vi "chose distance.vi"(10 "New direction":string, 11 "Current Direction":string) -> (2 "chosen  distance":dbl)   [LabVIEW 2015]
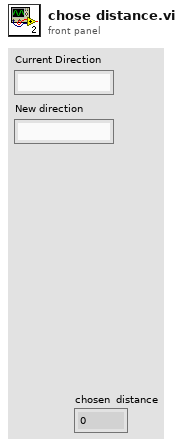
[diagram p1: front panel]
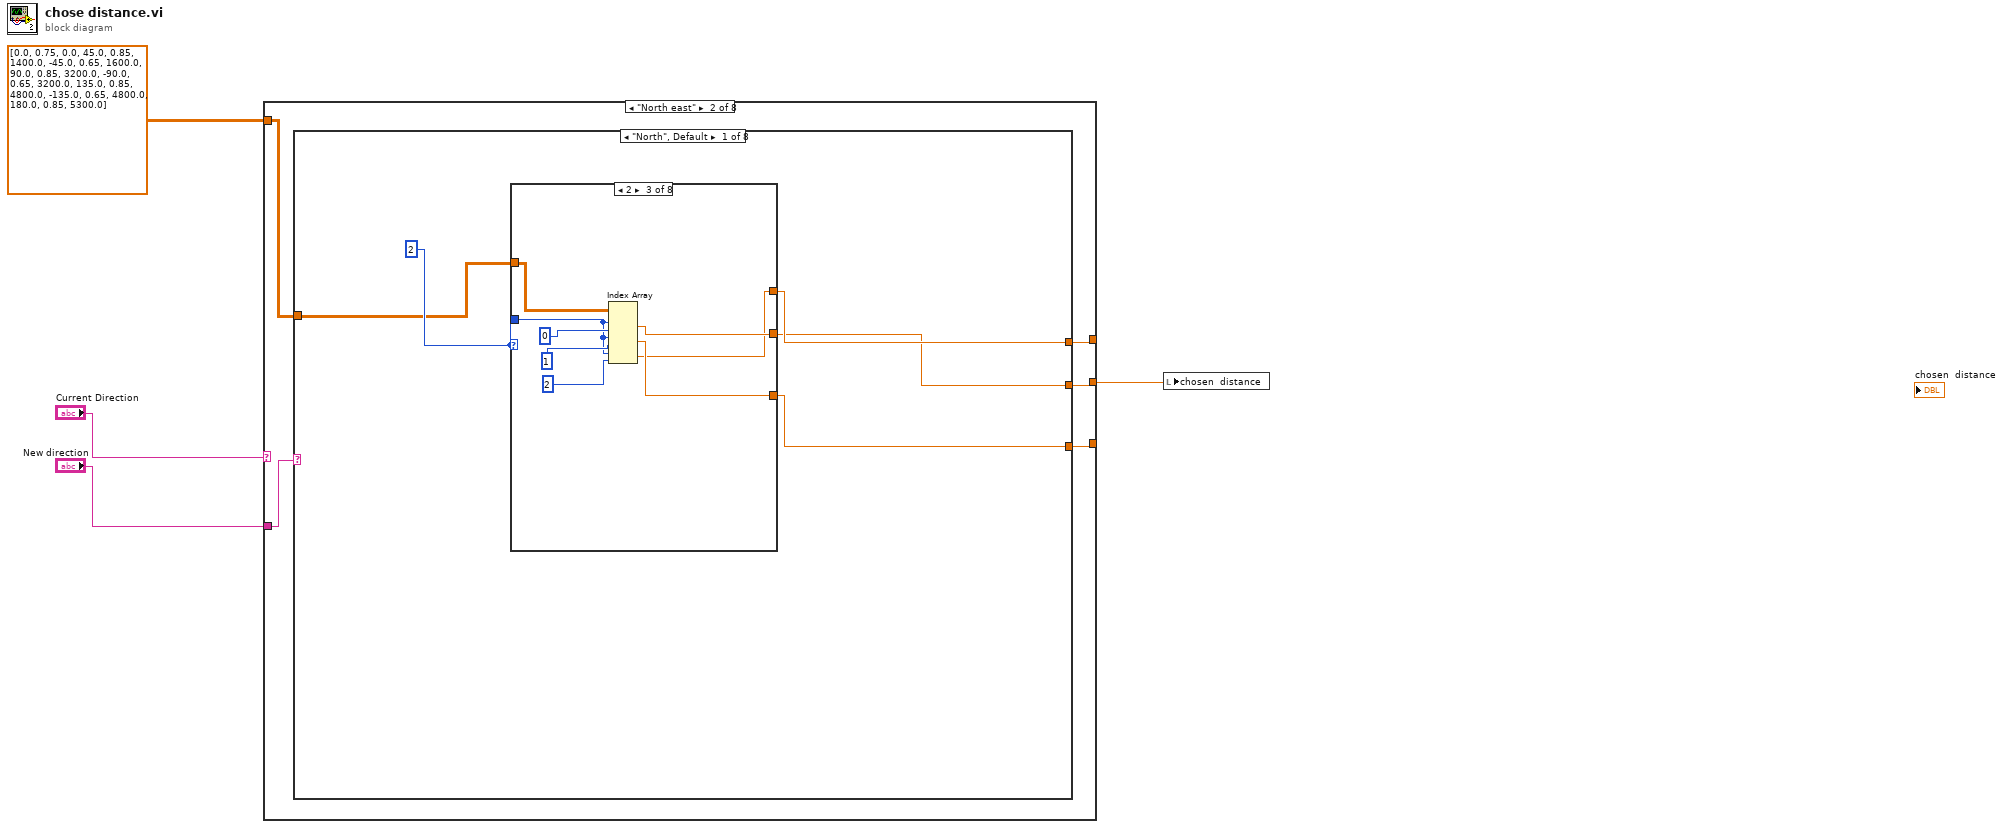
[diagram p0: block diagram]
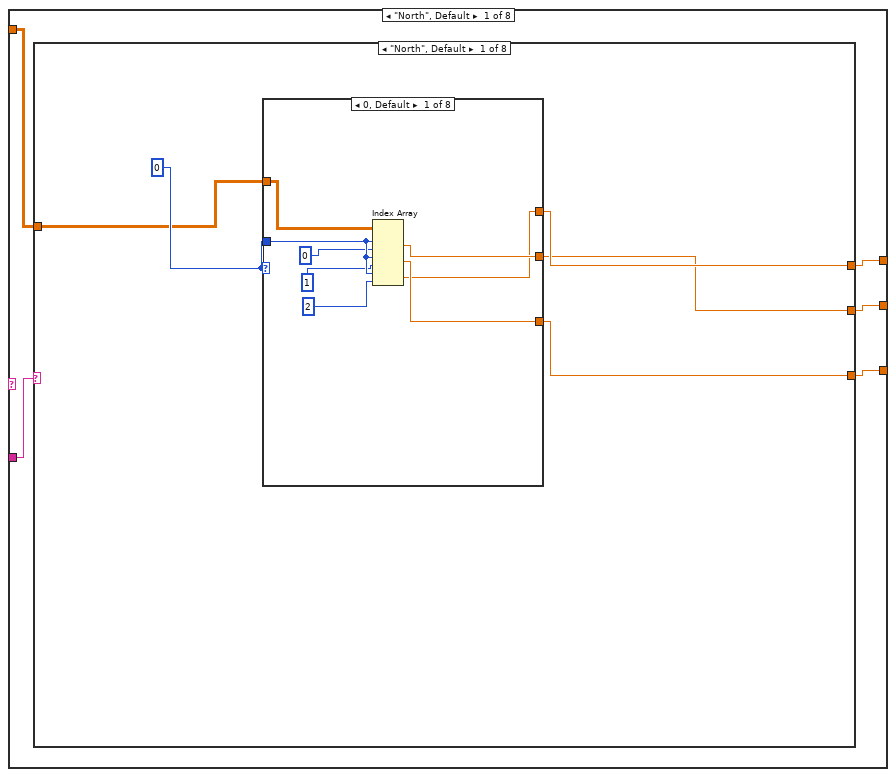
[diagram p2: hidden frame]
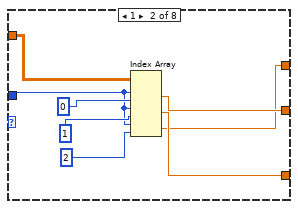
[diagram p3: hidden frame]
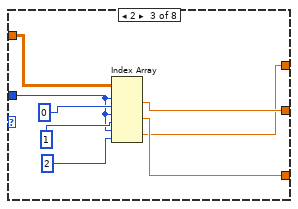
[diagram p4: hidden frame]
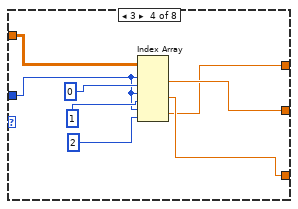
[diagram p5: hidden frame]
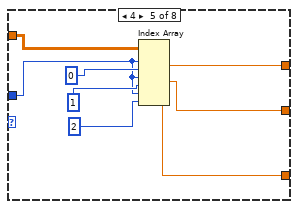
[diagram p6: hidden frame]
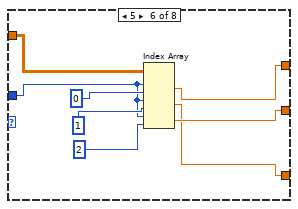
[diagram p7: hidden frame]
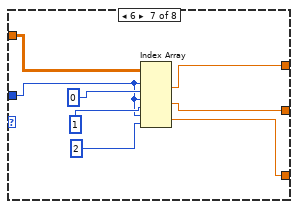
[diagram p8: hidden frame]
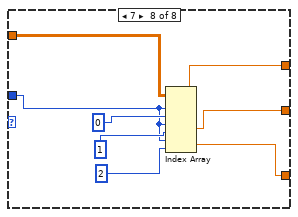
[diagram p9: hidden frame]
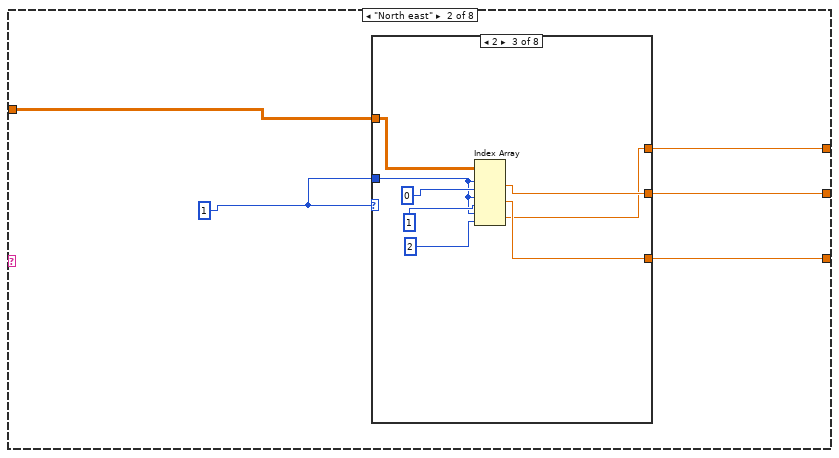
[diagram p10: hidden frame]
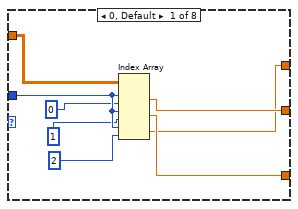
[diagram p11: hidden frame]
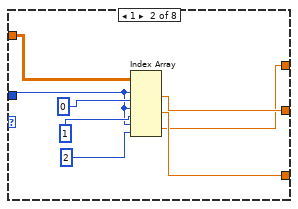
[diagram p12: hidden frame]
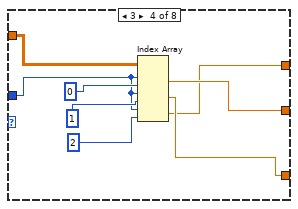
[diagram p13: hidden frame]
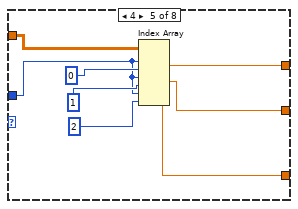
[diagram p14: hidden frame]
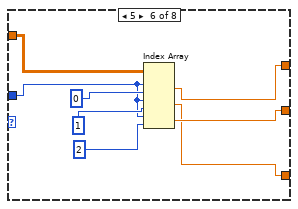
[diagram p15: hidden frame]
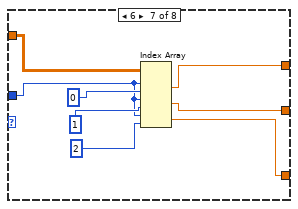
[diagram p16: hidden frame]
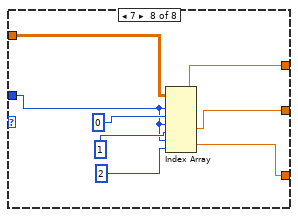
[diagram p17: hidden frame]
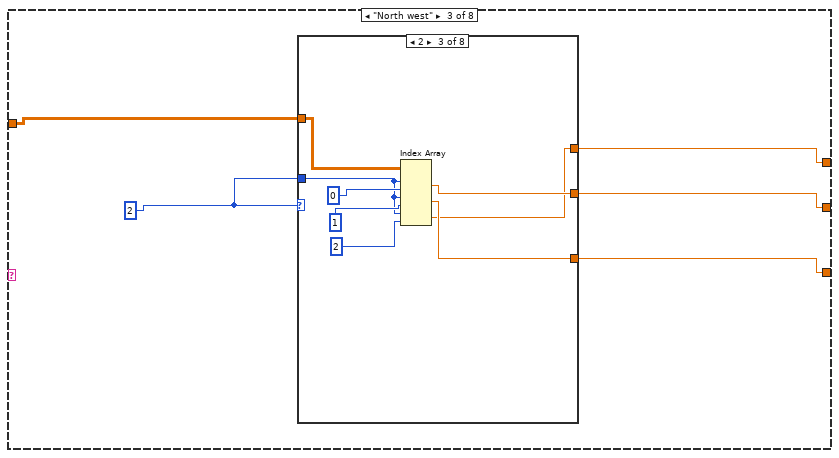
[diagram p18: hidden frame]
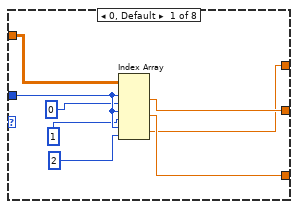
[diagram p19: hidden frame]
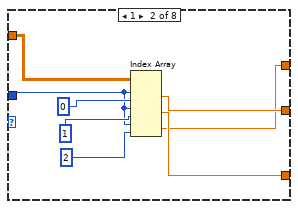
[diagram p20: hidden frame]
diagram:
  n1 = case shown="\"North east\"" "Current Direction" {
    tunnel: [w9 w566 w1123 w1680 w2237 w2794 w3351 w3908] -> _
    tunnel: [w8 w565 w1122 w1679 w2236 w2793 w3350 w3907] -> w1
    tunnel: [w7 w564 w1121 w1678 w2235 w2792 w3349 w3906] -> _
    tunnel: "New direction" -> [w5 w563 w1120 w1677 w2234 w2791 w3348 w3905]
    tunnel: dbl[][] [[0.0, 0.75, 0.0], [45.0, 0.85, 1400.0], [-45.0, 0.65, 1600.0], [90.0, 0.85, 3200.0], [-90.0, 0.65, 3200.0], [135.0, 0.85, 4800.0], [-135.0, 0.65, 4800.0], [180.0, 0.85, 5300.0]] -> [w6 w562 w1119 w1676 w2233 w2790 w3347 w3904]
    frame "North", Default {
      n2 = case shown="\"North\", Default" w5 {
        tunnel: [w13 w83 w151 w218 w288 w358 w426 w496] -> w9
        tunnel: [w12 w82 w150 w219 w287 w356 w425 w495] -> w8
        tunnel: [w11 w81 w149 w217 w286 w355 w424 w494] -> w7
        tunnel: w6 -> [w10 w79 w148 w220 w289 w357 w427 w493]
        frame "North", Default {
          w14 = 0
          n3 = case shown="0, Default" w14 {
            tunnel: [w18 w24 w32 w40 w48 w57 w64 w73] -> w13
            tunnel: [w20 w26 w34 w41 w50 w59 w66 w75] -> w12
            tunnel: [w19 w25 w33 w42 w49 w58 w65 w74] -> w11
            tunnel: w14 -> [w22 w27 w35 w43 w51 w56 w67 w72]
            tunnel: w10 -> [w15 w23 w31 w39 w47 w55 w63 w71]
            frame 0, Default {
              n4 = Index Array(array=w15, index (row) #1=w22, index (col) #1=0, index (row) #2=w22, index (col) #2=1, index (row) #3=w22, index (col) #3=2) -> (element #1=w20:dbl, element #2=w19:dbl, element #3=w18:dbl)
            }
            frame 1 {
              n5 = Index Array(array=w23, index (row) #1=w27, index (col) #1=0, index (row) #2=w27, index (col) #2=1, index (row) #3=w27, index (col) #3=2) -> (element #1=w26:dbl, element #2=w25:dbl, element #3=w24:dbl)
            }
            frame 2 {
              n6 = Index Array(array=w31, index (row) #1=w35, index (col) #1=0, index (row) #2=w35, index (col) #2=1, index (row) #3=w35, index (col) #3=2) -> (element #1=w34:dbl, element #2=w33:dbl, element #3=w32:dbl)
            }
            frame 3 {
              n7 = Index Array(array=w39, index (row) #1=w43, index (col) #1=0, index (row) #2=w43, index (col) #2=1, index (row) #3=w43, index (col) #3=2) -> (element #1=w41:dbl, element #2=w42:dbl, element #3=w40:dbl)
            }
            frame 4 {
              n8 = Index Array(array=w47, index (row) #1=w51, index (col) #1=0, index (row) #2=w51, index (col) #2=1, index (row) #3=w51, index (col) #3=2) -> (element #1=w48:dbl, element #2=w50:dbl, element #3=w49:dbl)
            }
            frame 5 {
              n9 = Index Array(array=w55, index (row) #1=w56, index (col) #1=0, index (row) #2=w56, index (col) #2=1, index (row) #3=w56, index (col) #3=2) -> (element #1=w57:dbl, element #2=w58:dbl, element #3=w59:dbl)
            }
            frame 6 {
              n10 = Index Array(array=w63, index (row) #1=w67, index (col) #1=0, index (row) #2=w67, index (col) #2=1, index (row) #3=w67, index (col) #3=2) -> (element #1=w64:dbl, element #2=w66:dbl, element #3=w65:dbl)
            }
            frame 7 {
              n11 = Index Array(array=w71, index (row) #1=w72, index (col) #1=0, index (row) #2=w72, index (col) #2=1, index (row) #3=w72, index (col) #3=2) -> (element #1=w73:dbl, element #2=w75:dbl, element #3=w74:dbl)
            }
          }
        }
        frame "North east" {
          w80 = 1
          n12 = case shown="2" w80 {
            tunnel: [w87 w93 w101 w109 w117 w126 w133 w142] -> w83
            tunnel: [w89 w95 w103 w110 w119 w128 w135 w144] -> w82
            tunnel: [w88 w94 w102 w111 w118 w127 w134 w143] -> w81
            tunnel: w80 -> [w91 w96 w104 w112 w120 w125 w136 w141]
            tunnel: w79 -> [w84 w92 w100 w108 w116 w124 w132 w140]
            frame 0, Default {
              n13 = Index Array(array=w84, index (row) #1=w91, index (col) #1=0, index (row) #2=w91, index (col) #2=1, index (row) #3=w91, index (col) #3=2) -> (element #1=w89:dbl, element #2=w88:dbl, element #3=w87:dbl)
            }
            frame 1 {
              n14 = Index Array(array=w92, index (row) #1=w96, index (col) #1=0, index (row) #2=w96, index (col) #2=1, index (row) #3=w96, index (col) #3=2) -> (element #1=w95:dbl, element #2=w94:dbl, element #3=w93:dbl)
            }
            frame 2 {
              n15 = Index Array(array=w100, index (row) #1=w104, index (col) #1=0, index (row) #2=w104, index (col) #2=1, index (row) #3=w104, index (col) #3=2) -> (element #1=w103:dbl, element #2=w102:dbl, element #3=w101:dbl)
            }
            frame 3 {
              n16 = Index Array(array=w108, index (row) #1=w112, index (col) #1=0, index (row) #2=w112, index (col) #2=1, index (row) #3=w112, index (col) #3=2) -> (element #1=w110:dbl, element #2=w111:dbl, element #3=w109:dbl)
            }
            frame 4 {
              n17 = Index Array(array=w116, index (row) #1=w120, index (col) #1=0, index (row) #2=w120, index (col) #2=1, index (row) #3=w120, index (col) #3=2) -> (element #1=w117:dbl, element #2=w119:dbl, element #3=w118:dbl)
            }
            frame 5 {
              n18 = Index Array(array=w124, index (row) #1=w125, index (col) #1=0, index (row) #2=w125, index (col) #2=1, index (row) #3=w125, index (col) #3=2) -> (element #1=w126:dbl, element #2=w127:dbl, element #3=w128:dbl)
            }
            frame 6 {
              n19 = Index Array(array=w132, index (row) #1=w136, index (col) #1=0, index (row) #2=w136, index (col) #2=1, index (row) #3=w136, index (col) #3=2) -> (element #1=w133:dbl, element #2=w135:dbl, element #3=w134:dbl)
            }
            frame 7 {
              n20 = Index Array(array=w140, index (row) #1=w141, index (col) #1=0, index (row) #2=w141, index (col) #2=1, index (row) #3=w141, index (col) #3=2) -> (element #1=w142:dbl, element #2=w144:dbl, element #3=w143:dbl)
            }
          }
        }
        frame "North west" {
          w152 = 2
          n21 = case shown="2" w152 {
            tunnel: [w156 w162 w170 w178 w186 w195 w202 w211] -> w151
            tunnel: [w158 w164 w172 w179 w188 w197 w204 w213] -> w150
            tunnel: [w157 w163 w171 w180 w187 w196 w203 w212] -> w149
            tunnel: w152 -> [w160 w165 w173 w181 w189 w194 w205 w210]
            tunnel: w148 -> [w153 w161 w169 w177 w185 w193 w201 w209]
            frame 0, Default {
              n22 = Index Array(array=w153, index (row) #1=w160, index (col) #1=0, index (row) #2=w160, index (col) #2=1, index (row) #3=w160, index (col) #3=2) -> (element #1=w158:dbl, element #2=w157:dbl, element #3=w156:dbl)
            }
            frame 1 {
              n23 = Index Array(array=w161, index (row) #1=w165, index (col) #1=0, index (row) #2=w165, index (col) #2=1, index (row) #3=w165, index (col) #3=2) -> (element #1=w164:dbl, element #2=w163:dbl, element #3=w162:dbl)
            }
            frame 2 {
              n24 = Index Array(array=w169, index (row) #1=w173, index (col) #1=0, index (row) #2=w173, index (col) #2=1, index (row) #3=w173, index (col) #3=2) -> (element #1=w172:dbl, element #2=w171:dbl, element #3=w170:dbl)
            }
            frame 3 {
              n25 = Index Array(array=w177, index (row) #1=w181, index (col) #1=0, index (row) #2=w181, index (col) #2=1, index (row) #3=w181, index (col) #3=2) -> (element #1=w179:dbl, element #2=w180:dbl, element #3=w178:dbl)
            }
            frame 4 {
              n26 = Index Array(array=w185, index (row) #1=w189, index (col) #1=0, index (row) #2=w189, index (col) #2=1, index (row) #3=w189, index (col) #3=2) -> (element #1=w186:dbl, element #2=w188:dbl, element #3=w187:dbl)
            }
            frame 5 {
              n27 = Index Array(array=w193, index (row) #1=w194, index (col) #1=0, index (row) #2=w194, index (col) #2=1, index (row) #3=w194, index (col) #3=2) -> (element #1=w195:dbl, element #2=w196:dbl, element #3=w197:dbl)
            }
            frame 6 {
              n28 = Index Array(array=w201, index (row) #1=w205, index (col) #1=0, index (row) #2=w205, index (col) #2=1, index (row) #3=w205, index (col) #3=2) -> (element #1=w202:dbl, element #2=w204:dbl, element #3=w203:dbl)
            }
            frame 7 {
              n29 = Index Array(array=w209, index (row) #1=w210, index (col) #1=0, index (row) #2=w210, index (col) #2=1, index (row) #3=w210, index (col) #3=2) -> (element #1=w211:dbl, element #2=w213:dbl, element #3=w212:dbl)
            }
          }
        }
        frame "West" {
          w221 = 4
          n30 = case shown="2" w221 {
            tunnel: [w225 w231 w239 w247 w255 w264 w271 w280] -> w218
            tunnel: [w227 w233 w241 w248 w257 w266 w273 w282] -> w219
            tunnel: [w226 w232 w240 w249 w256 w265 w272 w281] -> w217
            tunnel: w221 -> [w229 w234 w242 w250 w258 w263 w274 w279]
            tunnel: w220 -> [w222 w230 w238 w246 w254 w262 w270 w278]
            frame 0, Default {
              n31 = Index Array(array=w222, index (row) #1=w229, index (col) #1=0, index (row) #2=w229, index (col) #2=1, index (row) #3=w229, index (col) #3=2) -> (element #1=w227:dbl, element #2=w226:dbl, element #3=w225:dbl)
            }
            frame 1 {
              n32 = Index Array(array=w230, index (row) #1=w234, index (col) #1=0, index (row) #2=w234, index (col) #2=1, index (row) #3=w234, index (col) #3=2) -> (element #1=w233:dbl, element #2=w232:dbl, element #3=w231:dbl)
            }
            frame 2 {
              n33 = Index Array(array=w238, index (row) #1=w242, index (col) #1=0, index (row) #2=w242, index (col) #2=1, index (row) #3=w242, index (col) #3=2) -> (element #1=w241:dbl, element #2=w240:dbl, element #3=w239:dbl)
            }
            frame 3 {
              n34 = Index Array(array=w246, index (row) #1=w250, index (col) #1=0, index (row) #2=w250, index (col) #2=1, index (row) #3=w250, index (col) #3=2) -> (element #1=w248:dbl, element #2=w249:dbl, element #3=w247:dbl)
            }
            frame 4 {
              n35 = Index Array(array=w254, index (row) #1=w258, index (col) #1=0, index (row) #2=w258, index (col) #2=1, index (row) #3=w258, index (col) #3=2) -> (element #1=w255:dbl, element #2=w257:dbl, element #3=w256:dbl)
            }
            frame 5 {
              n36 = Index Array(array=w262, index (row) #1=w263, index (col) #1=0, index (row) #2=w263, index (col) #2=1, index (row) #3=w263, index (col) #3=2) -> (element #1=w264:dbl, element #2=w265:dbl, element #3=w266:dbl)
            }
            frame 6 {
              n37 = Index Array(array=w270, index (row) #1=w274, index (col) #1=0, index (row) #2=w274, index (col) #2=1, index (row) #3=w274, index (col) #3=2) -> (element #1=w271:dbl, element #2=w273:dbl, element #3=w272:dbl)
            }
            frame 7 {
              n38 = Index Array(array=w278, index (row) #1=w279, index (col) #1=0, index (row) #2=w279, index (col) #2=1, index (row) #3=w279, index (col) #3=2) -> (element #1=w280:dbl, element #2=w282:dbl, element #3=w281:dbl)
            }
          }
        }
        frame "East" {
          w290 = 3
          n39 = case shown="2" w290 {
            tunnel: [w294 w300 w308 w316 w324 w333 w340 w349] -> w288
            tunnel: [w296 w302 w310 w317 w326 w335 w342 w351] -> w287
            tunnel: [w295 w301 w309 w318 w325 w334 w341 w350] -> w286
            tunnel: w290 -> [w298 w303 w311 w319 w327 w332 w343 w348]
            tunnel: w289 -> [w291 w299 w307 w315 w323 w331 w339 w347]
            frame 0, Default {
              n40 = Index Array(array=w291, index (row) #1=w298, index (col) #1=0, index (row) #2=w298, index (col) #2=1, index (row) #3=w298, index (col) #3=2) -> (element #1=w296:dbl, element #2=w295:dbl, element #3=w294:dbl)
            }
            frame 1 {
              n41 = Index Array(array=w299, index (row) #1=w303, index (col) #1=0, index (row) #2=w303, index (col) #2=1, index (row) #3=w303, index (col) #3=2) -> (element #1=w302:dbl, element #2=w301:dbl, element #3=w300:dbl)
            }
            frame 2 {
              n42 = Index Array(array=w307, index (row) #1=w311, index (col) #1=0, index (row) #2=w311, index (col) #2=1, index (row) #3=w311, index (col) #3=2) -> (element #1=w310:dbl, element #2=w309:dbl, element #3=w308:dbl)
            }
            frame 3 {
              n43 = Index Array(array=w315, index (row) #1=w319, index (col) #1=0, index (row) #2=w319, index (col) #2=1, index (row) #3=w319, index (col) #3=2) -> (element #1=w317:dbl, element #2=w318:dbl, element #3=w316:dbl)
            }
            frame 4 {
              n44 = Index Array(array=w323, index (row) #1=w327, index (col) #1=0, index (row) #2=w327, index (col) #2=1, index (row) #3=w327, index (col) #3=2) -> (element #1=w324:dbl, element #2=w326:dbl, element #3=w325:dbl)
            }
            frame 5 {
              n45 = Index Array(array=w331, index (row) #1=w332, index (col) #1=0, index (row) #2=w332, index (col) #2=1, index (row) #3=w332, index (col) #3=2) -> (element #1=w333:dbl, element #2=w334:dbl, element #3=w335:dbl)
            }
            frame 6 {
              n46 = Index Array(array=w339, index (row) #1=w343, index (col) #1=0, index (row) #2=w343, index (col) #2=1, index (row) #3=w343, index (col) #3=2) -> (element #1=w340:dbl, element #2=w342:dbl, element #3=w341:dbl)
            }
            frame 7 {
              n47 = Index Array(array=w347, index (row) #1=w348, index (col) #1=0, index (row) #2=w348, index (col) #2=1, index (row) #3=w348, index (col) #3=2) -> (element #1=w349:dbl, element #2=w351:dbl, element #3=w350:dbl)
            }
          }
        }
        frame "South" {
          w359 = 7
          n48 = case shown="2" w359 {
            tunnel: [w363 w369 w377 w385 w393 w402 w409 w418] -> w358
            tunnel: [w365 w371 w379 w386 w395 w404 w411 w420] -> w356
            tunnel: [w364 w370 w378 w387 w394 w403 w410 w419] -> w355
            tunnel: w359 -> [w367 w372 w380 w388 w396 w401 w412 w417]
            tunnel: w357 -> [w360 w368 w376 w384 w392 w400 w408 w416]
            frame 0, Default {
              n49 = Index Array(array=w360, index (row) #1=w367, index (col) #1=0, index (row) #2=w367, index (col) #2=1, index (row) #3=w367, index (col) #3=2) -> (element #1=w365:dbl, element #2=w364:dbl, element #3=w363:dbl)
            }
            frame 1 {
              n50 = Index Array(array=w368, index (row) #1=w372, index (col) #1=0, index (row) #2=w372, index (col) #2=1, index (row) #3=w372, index (col) #3=2) -> (element #1=w371:dbl, element #2=w370:dbl, element #3=w369:dbl)
            }
            frame 2 {
              n51 = Index Array(array=w376, index (row) #1=w380, index (col) #1=0, index (row) #2=w380, index (col) #2=1, index (row) #3=w380, index (col) #3=2) -> (element #1=w379:dbl, element #2=w378:dbl, element #3=w377:dbl)
            }
            frame 3 {
              n52 = Index Array(array=w384, index (row) #1=w388, index (col) #1=0, index (row) #2=w388, index (col) #2=1, index (row) #3=w388, index (col) #3=2) -> (element #1=w386:dbl, element #2=w387:dbl, element #3=w385:dbl)
            }
            frame 4 {
              n53 = Index Array(array=w392, index (row) #1=w396, index (col) #1=0, index (row) #2=w396, index (col) #2=1, index (row) #3=w396, index (col) #3=2) -> (element #1=w393:dbl, element #2=w395:dbl, element #3=w394:dbl)
            }
            frame 5 {
              n54 = Index Array(array=w400, index (row) #1=w401, index (col) #1=0, index (row) #2=w401, index (col) #2=1, index (row) #3=w401, index (col) #3=2) -> (element #1=w402:dbl, element #2=w403:dbl, element #3=w404:dbl)
            }
            frame 6 {
              n55 = Index Array(array=w408, index (row) #1=w412, index (col) #1=0, index (row) #2=w412, index (col) #2=1, index (row) #3=w412, index (col) #3=2) -> (element #1=w409:dbl, element #2=w411:dbl, element #3=w410:dbl)
            }
            frame 7 {
              n56 = Index Array(array=w416, index (row) #1=w417, index (col) #1=0, index (row) #2=w417, index (col) #2=1, index (row) #3=w417, index (col) #3=2) -> (element #1=w418:dbl, element #2=w420:dbl, element #3=w419:dbl)
            }
          }
        }
        frame "South west" {
          w428 = 6
          n57 = case shown="2" w428 {
            tunnel: [w432 w438 w446 w454 w462 w471 w478 w487] -> w426
            tunnel: [w434 w440 w448 w455 w464 w473 w480 w489] -> w425
            tunnel: [w433 w439 w447 w456 w463 w472 w479 w488] -> w424
            tunnel: w428 -> [w436 w441 w449 w457 w465 w470 w481 w486]
            tunnel: w427 -> [w429 w437 w445 w453 w461 w469 w477 w485]
            frame 0, Default {
              n58 = Index Array(array=w429, index (row) #1=w436, index (col) #1=0, index (row) #2=w436, index (col) #2=1, index (row) #3=w436, index (col) #3=2) -> (element #1=w434:dbl, element #2=w433:dbl, element #3=w432:dbl)
            }
            frame 1 {
              n59 = Index Array(array=w437, index (row) #1=w441, index (col) #1=0, index (row) #2=w441, index (col) #2=1, index (row) #3=w441, index (col) #3=2) -> (element #1=w440:dbl, element #2=w439:dbl, element #3=w438:dbl)
            }
            frame 2 {
              n60 = Index Array(array=w445, index (row) #1=w449, index (col) #1=0, index (row) #2=w449, index (col) #2=1, index (row) #3=w449, index (col) #3=2) -> (element #1=w448:dbl, element #2=w447:dbl, element #3=w446:dbl)
            }
            frame 3 {
              n61 = Index Array(array=w453, index (row) #1=w457, index (col) #1=0, index (row) #2=w457, index (col) #2=1, index (row) #3=w457, index (col) #3=2) -> (element #1=w455:dbl, element #2=w456:dbl, element #3=w454:dbl)
            }
            frame 4 {
              n62 = Index Array(array=w461, index (row) #1=w465, index (col) #1=0, index (row) #2=w465, index (col) #2=1, index (row) #3=w465, index (col) #3=2) -> (element #1=w462:dbl, element #2=w464:dbl, element #3=w463:dbl)
            }
            frame 5 {
              n63 = Index Array(array=w469, index (row) #1=w470, index (col) #1=0, index (row) #2=w470, index (col) #2=1, index (row) #3=w470, index (col) #3=2) -> (element #1=w471:dbl, element #2=w472:dbl, element #3=w473:dbl)
            }
            frame 6 {
              n64 = Index Array(array=w477, index (row) #1=w481, index (col) #1=0, index (row) #2=w481, index (col) #2=1, index (row) #3=w481, index (col) #3=2) -> (element #1=w478:dbl, element #2=w480:dbl, element #3=w479:dbl)
            }
            frame 7 {
              n65 = Index Array(array=w485, index (row) #1=w486, index (col) #1=0, index (row) #2=w486, index (col) #2=1, index (row) #3=w486, index (col) #3=2) -> (element #1=w487:dbl, element #2=w489:dbl, element #3=w488:dbl)
            }
          }
        }
        frame "South east" {
          w497 = 5
          n66 = case shown="2" w497 {
            tunnel: [w501 w507 w515 w523 w531 w540 w547 w556] -> w496
            tunnel: [w503 w509 w517 w524 w533 w542 w549 w558] -> w495
            tunnel: [w502 w508 w516 w525 w532 w541 w548 w557] -> w494
            tunnel: w497 -> [w505 w510 w518 w526 w534 w539 w550 w555]
            tunnel: w493 -> [w498 w506 w514 w522 w530 w538 w546 w554]
            frame 0, Default {
              n67 = Index Array(array=w498, index (row) #1=w505, index (col) #1=0, index (row) #2=w505, index (col) #2=1, index (row) #3=w505, index (col) #3=2) -> (element #1=w503:dbl, element #2=w502:dbl, element #3=w501:dbl)
            }
            frame 1 {
              n68 = Index Array(array=w506, index (row) #1=w510, index (col) #1=0, index (row) #2=w510, index (col) #2=1, index (row) #3=w510, index (col) #3=2) -> (element #1=w509:dbl, element #2=w508:dbl, element #3=w507:dbl)
            }
            frame 2 {
              n69 = Index Array(array=w514, index (row) #1=w518, index (col) #1=0, index (row) #2=w518, index (col) #2=1, index (row) #3=w518, index (col) #3=2) -> (element #1=w517:dbl, element #2=w516:dbl, element #3=w515:dbl)
            }
            frame 3 {
              n70 = Index Array(array=w522, index (row) #1=w526, index (col) #1=0, index (row) #2=w526, index (col) #2=1, index (row) #3=w526, index (col) #3=2) -> (element #1=w524:dbl, element #2=w525:dbl, element #3=w523:dbl)
            }
            frame 4 {
              n71 = Index Array(array=w530, index (row) #1=w534, index (col) #1=0, index (row) #2=w534, index (col) #2=1, index (row) #3=w534, index (col) #3=2) -> (element #1=w531:dbl, element #2=w533:dbl, element #3=w532:dbl)
            }
            frame 5 {
              n72 = Index Array(array=w538, index (row) #1=w539, index (col) #1=0, index (row) #2=w539, index (col) #2=1, index (row) #3=w539, index (col) #3=2) -> (element #1=w540:dbl, element #2=w541:dbl, element #3=w542:dbl)
            }
            frame 6 {
              n73 = Index Array(array=w546, index (row) #1=w550, index (col) #1=0, index (row) #2=w550, index (col) #2=1, index (row) #3=w550, index (col) #3=2) -> (element #1=w547:dbl, element #2=w549:dbl, element #3=w548:dbl)
            }
            frame 7 {
              n74 = Index Array(array=w554, index (row) #1=w555, index (col) #1=0, index (row) #2=w555, index (col) #2=1, index (row) #3=w555, index (col) #3=2) -> (element #1=w556:dbl, element #2=w558:dbl, element #3=w557:dbl)
            }
          }
        }
      }
    }
    frame "North east" {
      n75 = case shown="\"North\", Default" w563 {
        tunnel: [w570 w640 w708 w775 w845 w915 w983 w1053] -> w566
        tunnel: [w569 w639 w707 w776 w844 w913 w982 w1052] -> w565
        tunnel: [w568 w638 w706 w774 w843 w912 w981 w1051] -> w564
        tunnel: w562 -> [w567 w636 w705 w777 w846 w914 w984 w1050]
        frame "North", Default {
          w571 = 2
          n76 = case shown="2" w571 {
            tunnel: [w575 w581 w589 w597 w605 w614 w621 w630] -> w570
            tunnel: [w577 w583 w591 w598 w607 w616 w623 w632] -> w569
            tunnel: [w576 w582 w590 w599 w606 w615 w622 w631] -> w568
            tunnel: w571 -> [w579 w584 w592 w600 w608 w613 w624 w629]
            tunnel: w567 -> [w572 w580 w588 w596 w604 w612 w620 w628]
            frame 0, Default {
              n77 = Index Array(array=w572, index (row) #1=w579, index (col) #1=0, index (row) #2=w579, index (col) #2=1, index (row) #3=w579, index (col) #3=2) -> (element #1=w577:dbl, element #2=w576:dbl, element #3=w575:dbl)
            }
            frame 1 {
              n78 = Index Array(array=w580, index (row) #1=w584, index (col) #1=0, index (row) #2=w584, index (col) #2=1, index (row) #3=w584, index (col) #3=2) -> (element #1=w583:dbl, element #2=w582:dbl, element #3=w581:dbl)
            }
            frame 2 {
              n79 = Index Array(array=w588, index (row) #1=w592, index (col) #1=0, index (row) #2=w592, index (col) #2=1, index (row) #3=w592, index (col) #3=2) -> (element #1=w591:dbl, element #2=w590:dbl, element #3=w589:dbl)
            }
            frame 3 {
              n80 = Index Array(array=w596, index (row) #1=w600, index (col) #1=0, index (row) #2=w600, index (col) #2=1, index (row) #3=w600, index (col) #3=2) -> (element #1=w598:dbl, element #2=w599:dbl, element #3=w597:dbl)
            }
            frame 4 {
              n81 = Index Array(array=w604, index (row) #1=w608, index (col) #1=0, index (row) #2=w608, index (col) #2=1, index (row) #3=w608, index (col) #3=2) -> (element #1=w605:dbl, element #2=w607:dbl, element #3=w606:dbl)
            }
            frame 5 {
              n82 = Index Array(array=w612, index (row) #1=w613, index (col) #1=0, index (row) #2=w613, index (col) #2=1, index (row) #3=w613, index (col) #3=2) -> (element #1=w614:dbl, element #2=w615:dbl, element #3=w616:dbl)
            }
            frame 6 {
              n83 = Index Array(array=w620, index (row) #1=w624, index (col) #1=0, index (row) #2=w624, index (col) #2=1, index (row) #3=w624, index (col) #3=2) -> (element #1=w621:dbl, element #2=w623:dbl, element #3=w622:dbl)
            }
            frame 7 {
              n84 = Index Array(array=w628, index (row) #1=w629, index (col) #1=0, index (row) #2=w629, index (col) #2=1, index (row) #3=w629, index (col) #3=2) -> (element #1=w630:dbl, element #2=w632:dbl, element #3=w631:dbl)
            }
          }
        }
        frame "North east" {
          w637 = 0
          n85 = case shown="2" w637 {
            tunnel: [w644 w650 w658 w666 w674 w683 w690 w699] -> w640
            tunnel: [w646 w652 w660 w667 w676 w685 w692 w701] -> w639
            tunnel: [w645 w651 w659 w668 w675 w684 w691 w700] -> w638
            tunnel: w637 -> [w648 w653 w661 w669 w677 w682 w693 w698]
            tunnel: w636 -> [w641 w649 w657 w665 w673 w681 w689 w697]
            frame 0, Default {
              n86 = Index Array(array=w641, index (row) #1=w648, index (col) #1=0, index (row) #2=w648, index (col) #2=1, index (row) #3=w648, index (col) #3=2) -> (element #1=w646:dbl, element #2=w645:dbl, element #3=w644:dbl)
            }
            frame 1 {
              n87 = Index Array(array=w649, index (row) #1=w653, index (col) #1=0, index (row) #2=w653, index (col) #2=1, index (row) #3=w653, index (col) #3=2) -> (element #1=w652:dbl, element #2=w651:dbl, element #3=w650:dbl)
            }
            frame 2 {
              n88 = Index Array(array=w657, index (row) #1=w661, index (col) #1=0, index (row) #2=w661, index (col) #2=1, index (row) #3=w661, index (col) #3=2) -> (element #1=w660:dbl, element #2=w659:dbl, element #3=w658:dbl)
            }
            frame 3 {
              n89 = Index Array(array=w665, index (row) #1=w669, index (col) #1=0, index (row) #2=w669, index (col) #2=1, index (row) #3=w669, index (col) #3=2) -> (element #1=w667:dbl, element #2=w668:dbl, element #3=w666:dbl)
            }
            frame 4 {
              n90 = Index Array(array=w673, index (row) #1=w677, index (col) #1=0, index (row) #2=w677, index (col) #2=1, index (row) #3=w677, index (col) #3=2) -> (element #1=w674:dbl, element #2=w676:dbl, element #3=w675:dbl)
            }
            frame 5 {
              n91 = Index Array(array=w681, index (row) #1=w682, index (col) #1=0, index (row) #2=w682, index (col) #2=1, index (row) #3=w682, index (col) #3=2) -> (element #1=w683:dbl, element #2=w684:dbl, element #3=w685:dbl)
            }
            frame 6 {
              n92 = Index Array(array=w689, index (row) #1=w693, index (col) #1=0, index (row) #2=w693, index (col) #2=1, index (row) #3=w693, index (col) #3=2) -> (element #1=w690:dbl, element #2=w692:dbl, element #3=w691:dbl)
            }
            frame 7 {
              n93 = Index Array(array=w697, index (row) #1=w698, index (col) #1=0, index (row) #2=w698, index (col) #2=1, index (row) #3=w698, index (col) #3=2) -> (element #1=w699:dbl, element #2=w701:dbl, element #3=w700:dbl)
            }
          }
        }
        frame "North west" {
          w709 = 4
          n94 = case shown="2" w709 {
            tunnel: [w713 w719 w727 w735 w743 w752 w759 w768] -> w708
            tunnel: [w715 w721 w729 w736 w745 w754 w761 w770] -> w707
            tunnel: [w714 w720 w728 w737 w744 w753 w760 w769] -> w706
            tunnel: w709 -> [w717 w722 w730 w738 w746 w751 w762 w767]
            tunnel: w705 -> [w710 w718 w726 w734 w742 w750 w758 w766]
            frame 0, Default {
              n95 = Index Array(array=w710, index (row) #1=w717, index (col) #1=0, index (row) #2=w717, index (col) #2=1, index (row) #3=w717, index (col) #3=2) -> (element #1=w715:dbl, element #2=w714:dbl, element #3=w713:dbl)
            }
            frame 1 {
              n96 = Index Array(array=w718, index (row) #1=w722, index (col) #1=0, index (row) #2=w722, index (col) #2=1, index (row) #3=w722, index (col) #3=2) -> (element #1=w721:dbl, element #2=w720:dbl, element #3=w719:dbl)
            }
            frame 2 {
              n97 = Index Array(array=w726, index (row) #1=w730, index (col) #1=0, index (row) #2=w730, index (col) #2=1, index (row) #3=w730, index (col) #3=2) -> (element #1=w729:dbl, element #2=w728:dbl, element #3=w727:dbl)
            }
            frame 3 {
              n98 = Index Array(array=w734, index (row) #1=w738, index (col) #1=0, index (row) #2=w738, index (col) #2=1, index (row) #3=w738, index (col) #3=2) -> (element #1=w736:dbl, element #2=w737:dbl, element #3=w735:dbl)
            }
            frame 4 {
              n99 = Index Array(array=w742, index (row) #1=w746, index (col) #1=0, index (row) #2=w746, index (col) #2=1, index (row) #3=w746, index (col) #3=2) -> (element #1=w743:dbl, element #2=w745:dbl, element #3=w744:dbl)
            }
            frame 5 {
              n100 = Index Array(array=w750, index (row) #1=w751, index (col) #1=0, index (row) #2=w751, index (col) #2=1, index (row) #3=w751, index (col) #3=2) -> (element #1=w752:dbl, element #2=w753:dbl, element #3=w754:dbl)
            }
            frame 6 {
              n101 = Index Array(array=w758, index (row) #1=w762, index (col) #1=0, index (row) #2=w762, index (col) #2=1, index (row) #3=w762, index (col) #3=2) -> (element #1=w759:dbl, element #2=w761:dbl, element #3=w760:dbl)
            }
            frame 7 {
              n102 = Index Array(array=w766, index (row) #1=w767, index (col) #1=0, index (row) #2=w767, index (col) #2=1, index (row) #3=w767, index (col) #3=2) -> (element #1=w768:dbl, element #2=w770:dbl, element #3=w769:dbl)
            }
          }
        }
        frame "West" {
          w778 = 6
          n103 = case shown="2" w778 {
            tunnel: [w782 w788 w796 w804 w812 w821 w828 w837] -> w775
            tunnel: [w784 w790 w798 w805 w814 w823 w830 w839] -> w776
            tunnel: [w783 w789 w797 w806 w813 w822 w829 w838] -> w774
            tunnel: w778 -> [w786 w791 w799 w807 w815 w820 w831 w836]
            tunnel: w777 -> [w779 w787 w795 w803 w811 w819 w827 w835]
            frame 0, Default {
              n104 = Index Array(array=w779, index (row) #1=w786, index (col) #1=0, index (row) #2=w786, index (col) #2=1, index (row) #3=w786, index (col) #3=2) -> (element #1=w784:dbl, element #2=w783:dbl, element #3=w782:dbl)
            }
            frame 1 {
              n105 = Index Array(array=w787, index (row) #1=w791, index (col) #1=0, index (row) #2=w791, index (col) #2=1, index (row) #3=w791, index (col) #3=2) -> (element #1=w790:dbl, element #2=w789:dbl, element #3=w788:dbl)
            }
            frame 2 {
              n106 = Index Array(array=w795, index (row) #1=w799, index (col) #1=0, index (row) #2=w799, index (col) #2=1, index (row) #3=w799, index (col) #3=2) -> (element #1=w798:dbl, element #2=w797:dbl, element #3=w796:dbl)
            }
            frame 3 {
              n107 = Index Array(array=w803, index (row) #1=w807, index (col) #1=0, index (row) #2=w807, index (col) #2=1, index (row) #3=w807, index (col) #3=2) -> (element #1=w805:dbl, element #2=w806:dbl, element #3=w804:dbl)
            }
            frame 4 {
              n108 = Index Array(array=w811, index (row) #1=w815, index (col) #1=0, index (row) #2=w815, index (col) #2=1, index (row) #3=w815, index (col) #3=2) -> (element #1=w812:dbl, element #2=w814:dbl, element #3=w813:dbl)
            }
            frame 5 {
              n109 = Index Array(array=w819, index (row) #1=w820, index (col) #1=0, index (row) #2=w820, index (col) #2=1, index (row) #3=w820, index (col) #3=2) -> (element #1=w821:dbl, element #2=w822:dbl, element #3=w823:dbl)
            }
            frame 6 {
              n110 = Index Array(array=w827, index (row) #1=w831, index (col) #1=0, index (row) #2=w831, index (col) #2=1, index (row) #3=w831, index (col) #3=2) -> (element #1=w828:dbl, element #2=w830:dbl, element #3=w829:dbl)
            }
            frame 7 {
              n111 = Index Array(array=w835, index (row) #1=w836, index (col) #1=0, index (row) #2=w836, index (col) #2=1, index (row) #3=w836, index (col) #3=2) -> (element #1=w837:dbl, element #2=w839:dbl, element #3=w838:dbl)
            }
          }
        }
        frame "East" {
          w847 = 1
          n112 = case shown="2" w847 {
            tunnel: [w851 w857 w865 w873 w881 w890 w897 w906] -> w845
            tunnel: [w853 w859 w867 w874 w883 w892 w899 w908] -> w844
            tunnel: [w852 w858 w866 w875 w882 w891 w898 w907] -> w843
            tunnel: w847 -> [w855 w860 w868 w876 w884 w889 w900 w905]
            tunnel: w846 -> [w848 w856 w864 w872 w880 w888 w896 w904]
            frame 0, Default {
              n113 = Index Array(array=w848, index (row) #1=w855, index (col) #1=0, index (row) #2=w855, index (col) #2=1, index (row) #3=w855, index (col) #3=2) -> (element #1=w853:dbl, element #2=w852:dbl, element #3=w851:dbl)
            }
            frame 1 {
              n114 = Index Array(array=w856, index (row) #1=w860, index (col) #1=0, index (row) #2=w860, index (col) #2=1, index (row) #3=w860, index (col) #3=2) -> (element #1=w859:dbl, element #2=w858:dbl, element #3=w857:dbl)
            }
            frame 2 {
              n115 = Index Array(array=w864, index (row) #1=w868, index (col) #1=0, index (row) #2=w868, index (col) #2=1, index (row) #3=w868, index (col) #3=2) -> (element #1=w867:dbl, element #2=w866:dbl, element #3=w865:dbl)
            }
            frame 3 {
              n116 = Index Array(array=w872, index (row) #1=w876, index (col) #1=0, index (row) #2=w876, index (col) #2=1, index (row) #3=w876, index (col) #3=2) -> (element #1=w874:dbl, element #2=w875:dbl, element #3=w873:dbl)
            }
            frame 4 {
              n117 = Index Array(array=w880, index (row) #1=w884, index (col) #1=0, index (row) #2=w884, index (col) #2=1, index (row) #3=w884, index (col) #3=2) -> (element #1=w881:dbl, element #2=w883:dbl, element #3=w882:dbl)
            }
            frame 5 {
              n118 = Index Array(array=w888, index (row) #1=w889, index (col) #1=0, index (row) #2=w889, index (col) #2=1, index (row) #3=w889, index (col) #3=2) -> (element #1=w890:dbl, element #2=w891:dbl, element #3=w892:dbl)
            }
            frame 6 {
              n119 = Index Array(array=w896, index (row) #1=w900, index (col) #1=0, index (row) #2=w900, index (col) #2=1, index (row) #3=w900, index (col) #3=2) -> (element #1=w897:dbl, element #2=w899:dbl, element #3=w898:dbl)
            }
            frame 7 {
              n120 = Index Array(array=w904, index (row) #1=w905, index (col) #1=0, index (row) #2=w905, index (col) #2=1, index (row) #3=w905, index (col) #3=2) -> (element #1=w906:dbl, element #2=w908:dbl, element #3=w907:dbl)
            }
          }
        }
        frame "South" {
          w916 = 5
          n121 = case shown="2" w916 {
            tunnel: [w920 w926 w934 w942 w950 w959 w966 w975] -> w915
            tunnel: [w922 w928 w936 w943 w952 w961 w968 w977] -> w913
            tunnel: [w921 w927 w935 w944 w951 w960 w967 w976] -> w912
            tunnel: w916 -> [w924 w929 w937 w945 w953 w958 w969 w974]
            tunnel: w914 -> [w917 w925 w933 w941 w949 w957 w965 w973]
            frame 0, Default {
              n122 = Index Array(array=w917, index (row) #1=w924, index (col) #1=0, index (row) #2=w924, index (col) #2=1, index (row) #3=w924, index (col) #3=2) -> (element #1=w922:dbl, element #2=w921:dbl, element #3=w920:dbl)
            }
            frame 1 {
              n123 = Index Array(array=w925, index (row) #1=w929, index (col) #1=0, index (row) #2=w929, index (col) #2=1, index (row) #3=w929, index (col) #3=2) -> (element #1=w928:dbl, element #2=w927:dbl, element #3=w926:dbl)
            }
            frame 2 {
              n124 = Index Array(array=w933, index (row) #1=w937, index (col) #1=0, index (row) #2=w937, index (col) #2=1, index (row) #3=w937, index (col) #3=2) -> (element #1=w936:dbl, element #2=w935:dbl, element #3=w934:dbl)
            }
            frame 3 {
              n125 = Index Array(array=w941, index (row) #1=w945, index (col) #1=0, index (row) #2=w945, index (col) #2=1, index (row) #3=w945, index (col) #3=2) -> (element #1=w943:dbl, element #2=w944:dbl, element #3=w942:dbl)
            }
            frame 4 {
              n126 = Index Array(array=w949, index (row) #1=w953, index (col) #1=0, index (row) #2=w953, index (col) #2=1, index (row) #3=w953, index (col) #3=2) -> (element #1=w950:dbl, element #2=w952:dbl, element #3=w951:dbl)
            }
            frame 5 {
              n127 = Index Array(array=w957, index (row) #1=w958, index (col) #1=0, index (row) #2=w958, index (col) #2=1, index (row) #3=w958, index (col) #3=2) -> (element #1=w959:dbl, element #2=w960:dbl, element #3=w961:dbl)
            }
            frame 6 {
              n128 = Index Array(array=w965, index (row) #1=w969, index (col) #1=0, index (row) #2=w969, index (col) #2=1, index (row) #3=w969, index (col) #3=2) -> (element #1=w966:dbl, element #2=w968:dbl, element #3=w967:dbl)
            }
            frame 7 {
              n129 = Index Array(array=w973, index (row) #1=w974, index (col) #1=0, index (row) #2=w974, index (col) #2=1, index (row) #3=w974, index (col) #3=2) -> (element #1=w975:dbl, element #2=w977:dbl, element #3=w976:dbl)
            }
          }
        }
        frame "South west" {
          w985 = 7
          n130 = case shown="2" w985 {
            tunnel: [w989 w995 w1003 w1011 w1019 w1028 w1035 w1044] -> w983
            tunnel: [w991 w997 w1005 w1012 w1021 w1030 w1037 w1046] -> w982
            tunnel: [w990 w996 w1004 w1013 w1020 w1029 w1036 w1045] -> w981
            tunnel: w985 -> [w993 w998 w1006 w1014 w1022 w1027 w1038 w1043]
            tunnel: w984 -> [w986 w994 w1002 w1010 w1018 w1026 w1034 w1042]
            frame 0, Default {
              n131 = Index Array(array=w986, index (row) #1=w993, index (col) #1=0, index (row) #2=w993, index (col) #2=1, index (row) #3=w993, index (col) #3=2) -> (element #1=w991:dbl, element #2=w990:dbl, element #3=w989:dbl)
            }
            frame 1 {
              n132 = Index Array(array=w994, index (row) #1=w998, index (col) #1=0, index (row) #2=w998, index (col) #2=1, index (row) #3=w998, index (col) #3=2) -> (element #1=w997:dbl, element #2=w996:dbl, element #3=w995:dbl)
            }
            frame 2 {
              n133 = Index Array(array=w1002, index (row) #1=w1006, index (col) #1=0, index (row) #2=w1006, index (col) #2=1, index (row) #3=w1006, index (col) #3=2) -> (element #1=w1005:dbl, element #2=w1004:dbl, element #3=w1003:dbl)
            }
            frame 3 {
              n134 = Index Array(array=w1010, index (row) #1=w1014, index (col) #1=0, index (row) #2=w1014, index (col) #2=1, index (row) #3=w1014, index (col) #3=2) -> (element #1=w1012:dbl, element #2=w1013:dbl, element #3=w1011:dbl)
            }
            frame 4 {
              n135 = Index Array(array=w1018, index (row) #1=w1022, index (col) #1=0, index (row) #2=w1022, index (col) #2=1, index (row) #3=w1022, index (col) #3=2) -> (element #1=w1019:dbl, element #2=w1021:dbl, element #3=w1020:dbl)
            }
            frame 5 {
              n136 = Index Array(array=w1026, index (row) #1=w1027, index (col) #1=0, index (row) #2=w1027, index (col) #2=1, index (row) #3=w1027, index (col) #3=2) -> (element #1=w1028:dbl, element #2=w1029:dbl, element #3=w1030:dbl)
            }
            frame 6 {
              n137 = Index Array(array=w1034, index (row) #1=w1038, index (col) #1=0, index (row) #2=w1038, index (col) #2=1, index (row) #3=w1038, index (col) #3=2) -> (element #1=w1035:dbl, element #2=w1037:dbl, element #3=w1036:dbl)
            }
            frame 7 {
              n138 = Index Array(array=w1042, index (row) #1=w1043, index (col) #1=0, index (row) #2=w1043, index (col) #2=1, index (row) #3=w1043, index (col) #3=2) -> (element #1=w1044:dbl, element #2=w1046:dbl, element #3=w1045:dbl)
            }
          }
        }
        frame "South east" {
          w1054 = 3
          n139 = case shown="2" w1054 {
            tunnel: [w1058 w1064 w1072 w1080 w1088 w1097 w1104 w1113] -> w1053
            tunnel: [w1060 w1066 w1074 w1081 w1090 w1099 w1106 w1115] -> w1052
            tunnel: [w1059 w1065 w1073 w1082 w1089 w1098 w1105 w1114] -> w1051
            tunnel: w1054 -> [w1062 w1067 w1075 w1083 w1091 w1096 w1107 w1112]
            tunnel: w1050 -> [w1055 w1063 w1071 w1079 w1087 w1095 w1103 w1111]
            frame 0, Default {
              n140 = Index Array(array=w1055, index (row) #1=w1062, index (col) #1=0, index (row) #2=w1062, index (col) #2=1, index (row) #3=w1062, index (col) #3=2) -> (element #1=w1060:dbl, element #2=w1059:dbl, element #3=w1058:dbl)
            }
            frame 1 {
              n141 = Index Array(array=w1063, index (row) #1=w1067, index (col) #1=0, index (row) #2=w1067, index (col) #2=1, index (row) #3=w1067, index (col) #3=2) -> (element #1=w1066:dbl, element #2=w1065:dbl, element #3=w1064:dbl)
            }
            frame 2 {
              n142 = Index Array(array=w1071, index (row) #1=w1075, index (col) #1=0, index (row) #2=w1075, index (col) #2=1, index (row) #3=w1075, index (col) #3=2) -> (element #1=w1074:dbl, element #2=w1073:dbl, element #3=w1072:dbl)
            }
            frame 3 {
              n143 = Index Array(array=w1079, index (row) #1=w1083, index (col) #1=0, index (row) #2=w1083, index (col) #2=1, index (row) #3=w1083, index (col) #3=2) -> (element #1=w1081:dbl, element #2=w1082:dbl, element #3=w1080:dbl)
            }
            frame 4 {
              n144 = Index Array(array=w1087, index (row) #1=w1091, index (col) #1=0, index (row) #2=w1091, index (col) #2=1, index (row) #3=w1091, index (col) #3=2) -> (element #1=w1088:dbl, element #2=w1090:dbl, element #3=w1089:dbl)
            }
            frame 5 {
              n145 = Index Array(array=w1095, index (row) #1=w1096, index (col) #1=0, index (row) #2=w1096, index (col) #2=1, index (row) #3=w1096, index (col) #3=2) -> (element #1=w1097:dbl, element #2=w1098:dbl, element #3=w1099:dbl)
            }
            frame 6 {
              n146 = Index Array(array=w1103, index (row) #1=w1107, index (col) #1=0, index (row) #2=w1107, index (col) #2=1, index (row) #3=w1107, index (col) #3=2) -> (element #1=w1104:dbl, element #2=w1106:dbl, element #3=w1105:dbl)
            }
            frame 7 {
              n147 = Index Array(array=w1111, index (row) #1=w1112, index (col) #1=0, index (row) #2=w1112, index (col) #2=1, index (row) #3=w1112, index (col) #3=2) -> (element #1=w1113:dbl, element #2=w1115:dbl, element #3=w1114:dbl)
            }
          }
        }
      }
    }
    frame "North west" {
      n148 = case shown="\"South east\"" w1120 {
        tunnel: [w1127 w1197 w1265 w1332 w1402 w1472 w1540 w1610] -> w1123
        tunnel: [w1126 w1196 w1264 w1333 w1401 w1470 w1539 w1609] -> w1122
        tunnel: [w1125 w1195 w1263 w1331 w1400 w1469 w1538 w1608] -> w1121
        tunnel: w1119 -> [w1124 w1193 w1262 w1334 w1403 w1471 w1541 w1607]
        frame "North", Default {
          w1128 = 1
          n149 = case shown="2" w1128 {
            tunnel: [w1132 w1138 w1146 w1154 w1162 w1171 w1178 w1187] -> w1127
            tunnel: [w1134 w1140 w1148 w1155 w1164 w1173 w1180 w1189] -> w1126
            tunnel: [w1133 w1139 w1147 w1156 w1163 w1172 w1179 w1188] -> w1125
            tunnel: w1128 -> [w1136 w1141 w1149 w1157 w1165 w1170 w1181 w1186]
            tunnel: w1124 -> [w1129 w1137 w1145 w1153 w1161 w1169 w1177 w1185]
            frame 0, Default {
              n150 = Index Array(array=w1129, index (row) #1=w1136, index (col) #1=0, index (row) #2=w1136, index (col) #2=1, index (row) #3=w1136, index (col) #3=2) -> (element #1=w1134:dbl, element #2=w1133:dbl, element #3=w1132:dbl)
            }
            frame 1 {
              n151 = Index Array(array=w1137, index (row) #1=w1141, index (col) #1=0, index (row) #2=w1141, index (col) #2=1, index (row) #3=w1141, index (col) #3=2) -> (element #1=w1140:dbl, element #2=w1139:dbl, element #3=w1138:dbl)
            }
            frame 2 {
              n152 = Index Array(array=w1145, index (row) #1=w1149, index (col) #1=0, index (row) #2=w1149, index (col) #2=1, index (row) #3=w1149, index (col) #3=2) -> (element #1=w1148:dbl, element #2=w1147:dbl, element #3=w1146:dbl)
            }
            frame 3 {
              n153 = Index Array(array=w1153, index (row) #1=w1157, index (col) #1=0, index (row) #2=w1157, index (col) #2=1, index (row) #3=w1157, index (col) #3=2) -> (element #1=w1155:dbl, element #2=w1156:dbl, element #3=w1154:dbl)
            }
            frame 4 {
              n154 = Index Array(array=w1161, index (row) #1=w1165, index (col) #1=0, index (row) #2=w1165, index (col) #2=1, index (row) #3=w1165, index (col) #3=2) -> (element #1=w1162:dbl, element #2=w1164:dbl, element #3=w1163:dbl)
            }
            frame 5 {
              n155 = Index Array(array=w1169, index (row) #1=w1170, index (col) #1=0, index (row) #2=w1170, index (col) #2=1, index (row) #3=w1170, index (col) #3=2) -> (element #1=w1171:dbl, element #2=w1172:dbl, element #3=w1173:dbl)
            }
            frame 6 {
              n156 = Index Array(array=w1177, index (row) #1=w1181, index (col) #1=0, index (row) #2=w1181, index (col) #2=1, index (row) #3=w1181, index (col) #3=2) -> (element #1=w1178:dbl, element #2=w1180:dbl, element #3=w1179:dbl)
            }
            frame 7 {
              n157 = Index Array(array=w1185, index (row) #1=w1186, index (col) #1=0, index (row) #2=w1186, index (col) #2=1, index (row) #3=w1186, index (col) #3=2) -> (element #1=w1187:dbl, element #2=w1189:dbl, element #3=w1188:dbl)
            }
          }
        }
        frame "North east" {
          w1194 = 3
          n158 = case shown="2" w1194 {
            tunnel: [w1201 w1207 w1215 w1223 w1231 w1240 w1247 w1256] -> w1197
            tunnel: [w1203 w1209 w1217 w1224 w1233 w1242 w1249 w1258] -> w1196
            tunnel: [w1202 w1208 w1216 w1225 w1232 w1241 w1248 w1257] -> w1195
            tunnel: w1194 -> [w1205 w1210 w1218 w1226 w1234 w1239 w1250 w1255]
            tunnel: w1193 -> [w1198 w1206 w1214 w1222 w1230 w1238 w1246 w1254]
            frame 0, Default {
              n159 = Index Array(array=w1198, index (row) #1=w1205, index (col) #1=0, index (row) #2=w1205, index (col) #2=1, index (row) #3=w1205, index (col) #3=2) -> (element #1=w1203:dbl, element #2=w1202:dbl, element #3=w1201:dbl)
            }
            frame 1 {
              n160 = Index Array(array=w1206, index (row) #1=w1210, index (col) #1=0, index (row) #2=w1210, index (col) #2=1, index (row) #3=w1210, index (col) #3=2) -> (element #1=w1209:dbl, element #2=w1208:dbl, element #3=w1207:dbl)
            }
            frame 2 {
              n161 = Index Array(array=w1214, index (row) #1=w1218, index (col) #1=0, index (row) #2=w1218, index (col) #2=1, index (row) #3=w1218, index (col) #3=2) -> (element #1=w1217:dbl, element #2=w1216:dbl, element #3=w1215:dbl)
            }
            frame 3 {
              n162 = Index Array(array=w1222, index (row) #1=w1226, index (col) #1=0, index (row) #2=w1226, index (col) #2=1, index (row) #3=w1226, index (col) #3=2) -> (element #1=w1224:dbl, element #2=w1225:dbl, element #3=w1223:dbl)
            }
            frame 4 {
              n163 = Index Array(array=w1230, index (row) #1=w1234, index (col) #1=0, index (row) #2=w1234, index (col) #2=1, index (row) #3=w1234, index (col) #3=2) -> (element #1=w1231:dbl, element #2=w1233:dbl, element #3=w1232:dbl)
            }
            frame 5 {
              n164 = Index Array(array=w1238, index (row) #1=w1239, index (col) #1=0, index (row) #2=w1239, index (col) #2=1, index (row) #3=w1239, index (col) #3=2) -> (element #1=w1240:dbl, element #2=w1241:dbl, element #3=w1242:dbl)
            }
            frame 6 {
              n165 = Index Array(array=w1246, index (row) #1=w1250, index (col) #1=0, index (row) #2=w1250, index (col) #2=1, index (row) #3=w1250, index (col) #3=2) -> (element #1=w1247:dbl, element #2=w1249:dbl, element #3=w1248:dbl)
            }
            frame 7 {
              n166 = Index Array(array=w1254, index (row) #1=w1255, index (col) #1=0, index (row) #2=w1255, index (col) #2=1, index (row) #3=w1255, index (col) #3=2) -> (element #1=w1256:dbl, element #2=w1258:dbl, element #3=w1257:dbl)
            }
          }
        }
        frame "North west" {
          w1266 = 0
          n167 = case shown="2" w1266 {
            tunnel: [w1270 w1276 w1284 w1292 w1300 w1309 w1316 w1325] -> w1265
            tunnel: [w1272 w1278 w1286 w1293 w1302 w1311 w1318 w1327] -> w1264
            tunnel: [w1271 w1277 w1285 w1294 w1301 w1310 w1317 w1326] -> w1263
            tunnel: w1266 -> [w1274 w1279 w1287 w1295 w1303 w1308 w1319 w1324]
            tunnel: w1262 -> [w1267 w1275 w1283 w1291 w1299 w1307 w1315 w1323]
            frame 0, Default {
              n168 = Index Array(array=w1267, index (row) #1=w1274, index (col) #1=0, index (row) #2=w1274, index (col) #2=1, index (row) #3=w1274, index (col) #3=2) -> (element #1=w1272:dbl, element #2=w1271:dbl, element #3=w1270:dbl)
            }
            frame 1 {
              n169 = Index Array(array=w1275, index (row) #1=w1279, index (col) #1=0, index (row) #2=w1279, index (col) #2=1, index (row) #3=w1279, index (col) #3=2) -> (element #1=w1278:dbl, element #2=w1277:dbl, element #3=w1276:dbl)
            }
            frame 2 {
              n170 = Index Array(array=w1283, index (row) #1=w1287, index (col) #1=0, index (row) #2=w1287, index (col) #2=1, index (row) #3=w1287, index (col) #3=2) -> (element #1=w1286:dbl, element #2=w1285:dbl, element #3=w1284:dbl)
            }
            frame 3 {
              n171 = Index Array(array=w1291, index (row) #1=w1295, index (col) #1=0, index (row) #2=w1295, index (col) #2=1, index (row) #3=w1295, index (col) #3=2) -> (element #1=w1293:dbl, element #2=w1294:dbl, element #3=w1292:dbl)
            }
            frame 4 {
              n172 = Index Array(array=w1299, index (row) #1=w1303, index (col) #1=0, index (row) #2=w1303, index (col) #2=1, index (row) #3=w1303, index (col) #3=2) -> (element #1=w1300:dbl, element #2=w1302:dbl, element #3=w1301:dbl)
            }
            frame 5 {
              n173 = Index Array(array=w1307, index (row) #1=w1308, index (col) #1=0, index (row) #2=w1308, index (col) #2=1, index (row) #3=w1308, index (col) #3=2) -> (element #1=w1309:dbl, element #2=w1310:dbl, element #3=w1311:dbl)
            }
            frame 6 {
              n174 = Index Array(array=w1315, index (row) #1=w1319, index (col) #1=0, index (row) #2=w1319, index (col) #2=1, index (row) #3=w1319, index (col) #3=2) -> (element #1=w1316:dbl, element #2=w1318:dbl, element #3=w1317:dbl)
            }
            frame 7 {
              n175 = Index Array(array=w1323, index (row) #1=w1324, index (col) #1=0, index (row) #2=w1324, index (col) #2=1, index (row) #3=w1324, index (col) #3=2) -> (element #1=w1325:dbl, element #2=w1327:dbl, element #3=w1326:dbl)
            }
          }
        }
        frame "West" {
          w1335 = 2
          n176 = case shown="2" w1335 {
            tunnel: [w1339 w1345 w1353 w1361 w1369 w1378 w1385 w1394] -> w1332
            tunnel: [w1341 w1347 w1355 w1362 w1371 w1380 w1387 w1396] -> w1333
            tunnel: [w1340 w1346 w1354 w1363 w1370 w1379 w1386 w1395] -> w1331
            tunnel: w1335 -> [w1343 w1348 w1356 w1364 w1372 w1377 w1388 w1393]
            tunnel: w1334 -> [w1336 w1344 w1352 w1360 w1368 w1376 w1384 w1392]
            frame 0, Default {
              n177 = Index Array(array=w1336, index (row) #1=w1343, index (col) #1=0, index (row) #2=w1343, index (col) #2=1, index (row) #3=w1343, index (col) #3=2) -> (element #1=w1341:dbl, element #2=w1340:dbl, element #3=w1339:dbl)
            }
            frame 1 {
              n178 = Index Array(array=w1344, index (row) #1=w1348, index (col) #1=0, index (row) #2=w1348, index (col) #2=1, index (row) #3=w1348, index (col) #3=2) -> (element #1=w1347:dbl, element #2=w1346:dbl, element #3=w1345:dbl)
            }
            frame 2 {
              n179 = Index Array(array=w1352, index (row) #1=w1356, index (col) #1=0, index (row) #2=w1356, index (col) #2=1, index (row) #3=w1356, index (col) #3=2) -> (element #1=w1355:dbl, element #2=w1354:dbl, element #3=w1353:dbl)
            }
            frame 3 {
              n180 = Index Array(array=w1360, index (row) #1=w1364, index (col) #1=0, index (row) #2=w1364, index (col) #2=1, index (row) #3=w1364, index (col) #3=2) -> (element #1=w1362:dbl, element #2=w1363:dbl, element #3=w1361:dbl)
            }
            frame 4 {
              n181 = Index Array(array=w1368, index (row) #1=w1372, index (col) #1=0, index (row) #2=w1372, index (col) #2=1, index (row) #3=w1372, index (col) #3=2) -> (element #1=w1369:dbl, element #2=w1371:dbl, element #3=w1370:dbl)
            }
            frame 5 {
              n182 = Index Array(array=w1376, index (row) #1=w1377, index (col) #1=0, index (row) #2=w1377, index (col) #2=1, index (row) #3=w1377, index (col) #3=2) -> (element #1=w1378:dbl, element #2=w1379:dbl, element #3=w1380:dbl)
            }
            frame 6 {
              n183 = Index Array(array=w1384, index (row) #1=w1388, index (col) #1=0, index (row) #2=w1388, index (col) #2=1, index (row) #3=w1388, index (col) #3=2) -> (element #1=w1385:dbl, element #2=w1387:dbl, element #3=w1386:dbl)
            }
            frame 7 {
              n184 = Index Array(array=w1392, index (row) #1=w1393, index (col) #1=0, index (row) #2=w1393, index (col) #2=1, index (row) #3=w1393, index (col) #3=2) -> (element #1=w1394:dbl, element #2=w1396:dbl, element #3=w1395:dbl)
            }
          }
        }
        frame "East" {
          w1404 = 5
          n185 = case shown="2" w1404 {
            tunnel: [w1408 w1414 w1422 w1430 w1438 w1447 w1454 w1463] -> w1402
            tunnel: [w1410 w1416 w1424 w1431 w1440 w1449 w1456 w1465] -> w1401
            tunnel: [w1409 w1415 w1423 w1432 w1439 w1448 w1455 w1464] -> w1400
            tunnel: w1404 -> [w1412 w1417 w1425 w1433 w1441 w1446 w1457 w1462]
            tunnel: w1403 -> [w1405 w1413 w1421 w1429 w1437 w1445 w1453 w1461]
            frame 0, Default {
              n186 = Index Array(array=w1405, index (row) #1=w1412, index (col) #1=0, index (row) #2=w1412, index (col) #2=1, index (row) #3=w1412, index (col) #3=2) -> (element #1=w1410:dbl, element #2=w1409:dbl, element #3=w1408:dbl)
            }
            frame 1 {
              n187 = Index Array(array=w1413, index (row) #1=w1417, index (col) #1=0, index (row) #2=w1417, index (col) #2=1, index (row) #3=w1417, index (col) #3=2) -> (element #1=w1416:dbl, element #2=w1415:dbl, element #3=w1414:dbl)
            }
            frame 2 {
              n188 = Index Array(array=w1421, index (row) #1=w1425, index (col) #1=0, index (row) #2=w1425, index (col) #2=1, index (row) #3=w1425, index (col) #3=2) -> (element #1=w1424:dbl, element #2=w1423:dbl, element #3=w1422:dbl)
            }
            frame 3 {
              n189 = Index Array(array=w1429, index (row) #1=w1433, index (col) #1=0, index (row) #2=w1433, index (col) #2=1, index (row) #3=w1433, index (col) #3=2) -> (element #1=w1431:dbl, element #2=w1432:dbl, element #3=w1430:dbl)
            }
            frame 4 {
              n190 = Index Array(array=w1437, index (row) #1=w1441, index (col) #1=0, index (row) #2=w1441, index (col) #2=1, index (row) #3=w1441, index (col) #3=2) -> (element #1=w1438:dbl, element #2=w1440:dbl, element #3=w1439:dbl)
            }
            frame 5 {
              n191 = Index Array(array=w1445, index (row) #1=w1446, index (col) #1=0, index (row) #2=w1446, index (col) #2=1, index (row) #3=w1446, index (col) #3=2) -> (element #1=w1447:dbl, element #2=w1448:dbl, element #3=w1449:dbl)
            }
            frame 6 {
              n192 = Index Array(array=w1453, index (row) #1=w1457, index (col) #1=0, index (row) #2=w1457, index (col) #2=1, index (row) #3=w1457, index (col) #3=2) -> (element #1=w1454:dbl, element #2=w1456:dbl, element #3=w1455:dbl)
            }
            frame 7 {
              n193 = Index Array(array=w1461, index (row) #1=w1462, index (col) #1=0, index (row) #2=w1462, index (col) #2=1, index (row) #3=w1462, index (col) #3=2) -> (element #1=w1463:dbl, element #2=w1465:dbl, element #3=w1464:dbl)
            }
          }
        }
        frame "South" {
          w1473 = 6
          n194 = case shown="2" w1473 {
            tunnel: [w1477 w1483 w1491 w1499 w1507 w1516 w1523 w1532] -> w1472
            tunnel: [w1479 w1485 w1493 w1500 w1509 w1518 w1525 w1534] -> w1470
            tunnel: [w1478 w1484 w1492 w1501 w1508 w1517 w1524 w1533] -> w1469
            tunnel: w1473 -> [w1481 w1486 w1494 w1502 w1510 w1515 w1526 w1531]
            tunnel: w1471 -> [w1474 w1482 w1490 w1498 w1506 w1514 w1522 w1530]
            frame 0, Default {
              n195 = Index Array(array=w1474, index (row) #1=w1481, index (col) #1=0, index (row) #2=w1481, index (col) #2=1, index (row) #3=w1481, index (col) #3=2) -> (element #1=w1479:dbl, element #2=w1478:dbl, element #3=w1477:dbl)
            }
            frame 1 {
              n196 = Index Array(array=w1482, index (row) #1=w1486, index (col) #1=0, index (row) #2=w1486, index (col) #2=1, index (row) #3=w1486, index (col) #3=2) -> (element #1=w1485:dbl, element #2=w1484:dbl, element #3=w1483:dbl)
            }
            frame 2 {
              n197 = Index Array(array=w1490, index (row) #1=w1494, index (col) #1=0, index (row) #2=w1494, index (col) #2=1, index (row) #3=w1494, index (col) #3=2) -> (element #1=w1493:dbl, element #2=w1492:dbl, element #3=w1491:dbl)
            }
            frame 3 {
              n198 = Index Array(array=w1498, index (row) #1=w1502, index (col) #1=0, index (row) #2=w1502, index (col) #2=1, index (row) #3=w1502, index (col) #3=2) -> (element #1=w1500:dbl, element #2=w1501:dbl, element #3=w1499:dbl)
            }
            frame 4 {
              n199 = Index Array(array=w1506, index (row) #1=w1510, index (col) #1=0, index (row) #2=w1510, index (col) #2=1, index (row) #3=w1510, index (col) #3=2) -> (element #1=w1507:dbl, element #2=w1509:dbl, element #3=w1508:dbl)
            }
            frame 5 {
              n200 = Index Array(array=w1514, index (row) #1=w1515, index (col) #1=0, index (row) #2=w1515, index (col) #2=1, index (row) #3=w1515, index (col) #3=2) -> (element #1=w1516:dbl, element #2=w1517:dbl, element #3=w1518:dbl)
            }
            frame 6 {
              n201 = Index Array(array=w1522, index (row) #1=w1526, index (col) #1=0, index (row) #2=w1526, index (col) #2=1, index (row) #3=w1526, index (col) #3=2) -> (element #1=w1523:dbl, element #2=w1525:dbl, element #3=w1524:dbl)
            }
            frame 7 {
              n202 = Index Array(array=w1530, index (row) #1=w1531, index (col) #1=0, index (row) #2=w1531, index (col) #2=1, index (row) #3=w1531, index (col) #3=2) -> (element #1=w1532:dbl, element #2=w1534:dbl, element #3=w1533:dbl)
            }
          }
        }
        frame "South west" {
          w1542 = 4
          n203 = case shown="2" w1542 {
            tunnel: [w1546 w1552 w1560 w1568 w1576 w1585 w1592 w1601] -> w1540
            tunnel: [w1548 w1554 w1562 w1569 w1578 w1587 w1594 w1603] -> w1539
            tunnel: [w1547 w1553 w1561 w1570 w1577 w1586 w1593 w1602] -> w1538
            tunnel: w1542 -> [w1550 w1555 w1563 w1571 w1579 w1584 w1595 w1600]
            tunnel: w1541 -> [w1543 w1551 w1559 w1567 w1575 w1583 w1591 w1599]
            frame 0, Default {
              n204 = Index Array(array=w1543, index (row) #1=w1550, index (col) #1=0, index (row) #2=w1550, index (col) #2=1, index (row) #3=w1550, index (col) #3=2) -> (element #1=w1548:dbl, element #2=w1547:dbl, element #3=w1546:dbl)
            }
            frame 1 {
              n205 = Index Array(array=w1551, index (row) #1=w1555, index (col) #1=0, index (row) #2=w1555, index (col) #2=1, index (row) #3=w1555, index (col) #3=2) -> (element #1=w1554:dbl, element #2=w1553:dbl, element #3=w1552:dbl)
            }
            frame 2 {
              n206 = Index Array(array=w1559, index (row) #1=w1563, index (col) #1=0, index (row) #2=w1563, index (col) #2=1, index (row) #3=w1563, index (col) #3=2) -> (element #1=w1562:dbl, element #2=w1561:dbl, element #3=w1560:dbl)
            }
            frame 3 {
              n207 = Index Array(array=w1567, index (row) #1=w1571, index (col) #1=0, index (row) #2=w1571, index (col) #2=1, index (row) #3=w1571, index (col) #3=2) -> (element #1=w1569:dbl, element #2=w1570:dbl, element #3=w1568:dbl)
            }
            frame 4 {
              n208 = Index Array(array=w1575, index (row) #1=w1579, index (col) #1=0, index (row) #2=w1579, index (col) #2=1, index (row) #3=w1579, index (col) #3=2) -> (element #1=w1576:dbl, element #2=w1578:dbl, element #3=w1577:dbl)
            }
            frame 5 {
              n209 = Index Array(array=w1583, index (row) #1=w1584, index (col) #1=0, index (row) #2=w1584, index (col) #2=1, index (row) #3=w1584, index (col) #3=2) -> (element #1=w1585:dbl, element #2=w1586:dbl, element #3=w1587:dbl)
            }
            frame 6 {
              n210 = Index Array(array=w1591, index (row) #1=w1595, index (col) #1=0, index (row) #2=w1595, index (col) #2=1, index (row) #3=w1595, index (col) #3=2) -> (element #1=w1592:dbl, element #2=w1594:dbl, element #3=w1593:dbl)
            }
            frame 7 {
              n211 = Index Array(array=w1599, index (row) #1=w1600, index (col) #1=0, index (row) #2=w1600, index (col) #2=1, index (row) #3=w1600, index (col) #3=2) -> (element #1=w1601:dbl, element #2=w1603:dbl, element #3=w1602:dbl)
            }
          }
        }
        frame "South east" {
          w1611 = 7
          n212 = case shown="2" w1611 {
            tunnel: [w1615 w1621 w1629 w1637 w1645 w1654 w1661 w1670] -> w1610
            tunnel: [w1617 w1623 w1631 w1638 w1647 w1656 w1663 w1672] -> w1609
            tunnel: [w1616 w1622 w1630 w1639 w1646 w1655 w1662 w1671] -> w1608
            tunnel: w1611 -> [w1619 w1624 w1632 w1640 w1648 w1653 w1664 w1669]
            tunnel: w1607 -> [w1612 w1620 w1628 w1636 w1644 w1652 w1660 w1668]
            frame 0, Default {
              n213 = Index Array(array=w1612, index (row) #1=w1619, index (col) #1=0, index (row) #2=w1619, index (col) #2=1, index (row) #3=w1619, index (col) #3=2) -> (element #1=w1617:dbl, element #2=w1616:dbl, element #3=w1615:dbl)
            }
            frame 1 {
              n214 = Index Array(array=w1620, index (row) #1=w1624, index (col) #1=0, index (row) #2=w1624, index (col) #2=1, index (row) #3=w1624, index (col) #3=2) -> (element #1=w1623:dbl, element #2=w1622:dbl, element #3=w1621:dbl)
            }
            frame 2 {
              n215 = Index Array(array=w1628, index (row) #1=w1632, index (col) #1=0, index (row) #2=w1632, index (col) #2=1, index (row) #3=w1632, index (col) #3=2) -> (element #1=w1631:dbl, element #2=w1630:dbl, element #3=w1629:dbl)
            }
            frame 3 {
              n216 = Index Array(array=w1636, index (row) #1=w1640, index (col) #1=0, index (row) #2=w1640, index (col) #2=1, index (row) #3=w1640, index (col) #3=2) -> (element #1=w1638:dbl, element #2=w1639:dbl, element #3=w1637:dbl)
            }
            frame 4 {
              n217 = Index Array(array=w1644, index (row) #1=w1648, index (col) #1=0, index (row) #2=w1648, index (col) #2=1, index (row) #3=w1648, index (col) #3=2) -> (element #1=w1645:dbl, element #2=w1647:dbl, element #3=w1646:dbl)
            }
            frame 5 {
              n218 = Index Array(array=w1652, index (row) #1=w1653, index (col) #1=0, index (row) #2=w1653, index (col) #2=1, index (row) #3=w1653, index (col) #3=2) -> (element #1=w1654:dbl, element #2=w1655:dbl, element #3=w1656:dbl)
            }
            frame 6 {
              n219 = Index Array(array=w1660, index (row) #1=w1664, index (col) #1=0, index (row) #2=w1664, index (col) #2=1, index (row) #3=w1664, index (col) #3=2) -> (element #1=w1661:dbl, element #2=w1663:dbl, element #3=w1662:dbl)
            }
            frame 7 {
              n220 = Index Array(array=w1668, index (row) #1=w1669, index (col) #1=0, index (row) #2=w1669, index (col) #2=1, index (row) #3=w1669, index (col) #3=2) -> (element #1=w1670:dbl, element #2=w1672:dbl, element #3=w1671:dbl)
            }
          }
        }
      }
    }
    frame "West" {
      n221 = case shown="\"North\", Default" w1677 {
        tunnel: [w1684 w1754 w1822 w1889 w1959 w2029 w2097 w2167] -> w1680
        tunnel: [w1683 w1753 w1821 w1890 w1958 w2027 w2096 w2166] -> w1679
        tunnel: [w1682 w1752 w1820 w1888 w1957 w2026 w2095 w2165] -> w1678
        tunnel: w1676 -> [w1681 w1750 w1819 w1891 w1960 w2028 w2098 w2164]
        frame "North", Default {
          w1685 = 3
          n222 = case shown="2" w1685 {
            tunnel: [w1689 w1695 w1703 w1711 w1719 w1728 w1735 w1744] -> w1684
            tunnel: [w1691 w1697 w1705 w1712 w1721 w1730 w1737 w1746] -> w1683
            tunnel: [w1690 w1696 w1704 w1713 w1720 w1729 w1736 w1745] -> w1682
            tunnel: w1685 -> [w1693 w1698 w1706 w1714 w1722 w1727 w1738 w1743]
            tunnel: w1681 -> [w1686 w1694 w1702 w1710 w1718 w1726 w1734 w1742]
            frame 0, Default {
              n223 = Index Array(array=w1686, index (row) #1=w1693, index (col) #1=0, index (row) #2=w1693, index (col) #2=1, index (row) #3=w1693, index (col) #3=2) -> (element #1=w1691:dbl, element #2=w1690:dbl, element #3=w1689:dbl)
            }
            frame 1 {
              n224 = Index Array(array=w1694, index (row) #1=w1698, index (col) #1=0, index (row) #2=w1698, index (col) #2=1, index (row) #3=w1698, index (col) #3=2) -> (element #1=w1697:dbl, element #2=w1696:dbl, element #3=w1695:dbl)
            }
            frame 2 {
              n225 = Index Array(array=w1702, index (row) #1=w1706, index (col) #1=0, index (row) #2=w1706, index (col) #2=1, index (row) #3=w1706, index (col) #3=2) -> (element #1=w1705:dbl, element #2=w1704:dbl, element #3=w1703:dbl)
            }
            frame 3 {
              n226 = Index Array(array=w1710, index (row) #1=w1714, index (col) #1=0, index (row) #2=w1714, index (col) #2=1, index (row) #3=w1714, index (col) #3=2) -> (element #1=w1712:dbl, element #2=w1713:dbl, element #3=w1711:dbl)
            }
            frame 4 {
              n227 = Index Array(array=w1718, index (row) #1=w1722, index (col) #1=0, index (row) #2=w1722, index (col) #2=1, index (row) #3=w1722, index (col) #3=2) -> (element #1=w1719:dbl, element #2=w1721:dbl, element #3=w1720:dbl)
            }
            frame 5 {
              n228 = Index Array(array=w1726, index (row) #1=w1727, index (col) #1=0, index (row) #2=w1727, index (col) #2=1, index (row) #3=w1727, index (col) #3=2) -> (element #1=w1728:dbl, element #2=w1729:dbl, element #3=w1730:dbl)
            }
            frame 6 {
              n229 = Index Array(array=w1734, index (row) #1=w1738, index (col) #1=0, index (row) #2=w1738, index (col) #2=1, index (row) #3=w1738, index (col) #3=2) -> (element #1=w1735:dbl, element #2=w1737:dbl, element #3=w1736:dbl)
            }
            frame 7 {
              n230 = Index Array(array=w1742, index (row) #1=w1743, index (col) #1=0, index (row) #2=w1743, index (col) #2=1, index (row) #3=w1743, index (col) #3=2) -> (element #1=w1744:dbl, element #2=w1746:dbl, element #3=w1745:dbl)
            }
          }
        }
        frame "North east" {
          w1751 = 5
          n231 = case shown="2" w1751 {
            tunnel: [w1758 w1764 w1772 w1780 w1788 w1797 w1804 w1813] -> w1754
            tunnel: [w1760 w1766 w1774 w1781 w1790 w1799 w1806 w1815] -> w1753
            tunnel: [w1759 w1765 w1773 w1782 w1789 w1798 w1805 w1814] -> w1752
            tunnel: w1751 -> [w1762 w1767 w1775 w1783 w1791 w1796 w1807 w1812]
            tunnel: w1750 -> [w1755 w1763 w1771 w1779 w1787 w1795 w1803 w1811]
            frame 0, Default {
              n232 = Index Array(array=w1755, index (row) #1=w1762, index (col) #1=0, index (row) #2=w1762, index (col) #2=1, index (row) #3=w1762, index (col) #3=2) -> (element #1=w1760:dbl, element #2=w1759:dbl, element #3=w1758:dbl)
            }
            frame 1 {
              n233 = Index Array(array=w1763, index (row) #1=w1767, index (col) #1=0, index (row) #2=w1767, index (col) #2=1, index (row) #3=w1767, index (col) #3=2) -> (element #1=w1766:dbl, element #2=w1765:dbl, element #3=w1764:dbl)
            }
            frame 2 {
              n234 = Index Array(array=w1771, index (row) #1=w1775, index (col) #1=0, index (row) #2=w1775, index (col) #2=1, index (row) #3=w1775, index (col) #3=2) -> (element #1=w1774:dbl, element #2=w1773:dbl, element #3=w1772:dbl)
            }
            frame 3 {
              n235 = Index Array(array=w1779, index (row) #1=w1783, index (col) #1=0, index (row) #2=w1783, index (col) #2=1, index (row) #3=w1783, index (col) #3=2) -> (element #1=w1781:dbl, element #2=w1782:dbl, element #3=w1780:dbl)
            }
            frame 4 {
              n236 = Index Array(array=w1787, index (row) #1=w1791, index (col) #1=0, index (row) #2=w1791, index (col) #2=1, index (row) #3=w1791, index (col) #3=2) -> (element #1=w1788:dbl, element #2=w1790:dbl, element #3=w1789:dbl)
            }
            frame 5 {
              n237 = Index Array(array=w1795, index (row) #1=w1796, index (col) #1=0, index (row) #2=w1796, index (col) #2=1, index (row) #3=w1796, index (col) #3=2) -> (element #1=w1797:dbl, element #2=w1798:dbl, element #3=w1799:dbl)
            }
            frame 6 {
              n238 = Index Array(array=w1803, index (row) #1=w1807, index (col) #1=0, index (row) #2=w1807, index (col) #2=1, index (row) #3=w1807, index (col) #3=2) -> (element #1=w1804:dbl, element #2=w1806:dbl, element #3=w1805:dbl)
            }
            frame 7 {
              n239 = Index Array(array=w1811, index (row) #1=w1812, index (col) #1=0, index (row) #2=w1812, index (col) #2=1, index (row) #3=w1812, index (col) #3=2) -> (element #1=w1813:dbl, element #2=w1815:dbl, element #3=w1814:dbl)
            }
          }
        }
        frame "North west" {
          w1823 = 1
          n240 = case shown="2" w1823 {
            tunnel: [w1827 w1833 w1841 w1849 w1857 w1866 w1873 w1882] -> w1822
            tunnel: [w1829 w1835 w1843 w1850 w1859 w1868 w1875 w1884] -> w1821
            tunnel: [w1828 w1834 w1842 w1851 w1858 w1867 w1874 w1883] -> w1820
            tunnel: w1823 -> [w1831 w1836 w1844 w1852 w1860 w1865 w1876 w1881]
            tunnel: w1819 -> [w1824 w1832 w1840 w1848 w1856 w1864 w1872 w1880]
            frame 0, Default {
              n241 = Index Array(array=w1824, index (row) #1=w1831, index (col) #1=0, index (row) #2=w1831, index (col) #2=1, index (row) #3=w1831, index (col) #3=2) -> (element #1=w1829:dbl, element #2=w1828:dbl, element #3=w1827:dbl)
            }
            frame 1 {
              n242 = Index Array(array=w1832, index (row) #1=w1836, index (col) #1=0, index (row) #2=w1836, index (col) #2=1, index (row) #3=w1836, index (col) #3=2) -> (element #1=w1835:dbl, element #2=w1834:dbl, element #3=w1833:dbl)
            }
            frame 2 {
              n243 = Index Array(array=w1840, index (row) #1=w1844, index (col) #1=0, index (row) #2=w1844, index (col) #2=1, index (row) #3=w1844, index (col) #3=2) -> (element #1=w1843:dbl, element #2=w1842:dbl, element #3=w1841:dbl)
            }
            frame 3 {
              n244 = Index Array(array=w1848, index (row) #1=w1852, index (col) #1=0, index (row) #2=w1852, index (col) #2=1, index (row) #3=w1852, index (col) #3=2) -> (element #1=w1850:dbl, element #2=w1851:dbl, element #3=w1849:dbl)
            }
            frame 4 {
              n245 = Index Array(array=w1856, index (row) #1=w1860, index (col) #1=0, index (row) #2=w1860, index (col) #2=1, index (row) #3=w1860, index (col) #3=2) -> (element #1=w1857:dbl, element #2=w1859:dbl, element #3=w1858:dbl)
            }
            frame 5 {
              n246 = Index Array(array=w1864, index (row) #1=w1865, index (col) #1=0, index (row) #2=w1865, index (col) #2=1, index (row) #3=w1865, index (col) #3=2) -> (element #1=w1866:dbl, element #2=w1867:dbl, element #3=w1868:dbl)
            }
            frame 6 {
              n247 = Index Array(array=w1872, index (row) #1=w1876, index (col) #1=0, index (row) #2=w1876, index (col) #2=1, index (row) #3=w1876, index (col) #3=2) -> (element #1=w1873:dbl, element #2=w1875:dbl, element #3=w1874:dbl)
            }
            frame 7 {
              n248 = Index Array(array=w1880, index (row) #1=w1881, index (col) #1=0, index (row) #2=w1881, index (col) #2=1, index (row) #3=w1881, index (col) #3=2) -> (element #1=w1882:dbl, element #2=w1884:dbl, element #3=w1883:dbl)
            }
          }
        }
        frame "West" {
          w1892 = 0
          n249 = case shown="2" w1892 {
            tunnel: [w1896 w1902 w1910 w1918 w1926 w1935 w1942 w1951] -> w1889
            tunnel: [w1898 w1904 w1912 w1919 w1928 w1937 w1944 w1953] -> w1890
            tunnel: [w1897 w1903 w1911 w1920 w1927 w1936 w1943 w1952] -> w1888
            tunnel: w1892 -> [w1900 w1905 w1913 w1921 w1929 w1934 w1945 w1950]
            tunnel: w1891 -> [w1893 w1901 w1909 w1917 w1925 w1933 w1941 w1949]
            frame 0, Default {
              n250 = Index Array(array=w1893, index (row) #1=w1900, index (col) #1=0, index (row) #2=w1900, index (col) #2=1, index (row) #3=w1900, index (col) #3=2) -> (element #1=w1898:dbl, element #2=w1897:dbl, element #3=w1896:dbl)
            }
            frame 1 {
              n251 = Index Array(array=w1901, index (row) #1=w1905, index (col) #1=0, index (row) #2=w1905, index (col) #2=1, index (row) #3=w1905, index (col) #3=2) -> (element #1=w1904:dbl, element #2=w1903:dbl, element #3=w1902:dbl)
            }
            frame 2 {
              n252 = Index Array(array=w1909, index (row) #1=w1913, index (col) #1=0, index (row) #2=w1913, index (col) #2=1, index (row) #3=w1913, index (col) #3=2) -> (element #1=w1912:dbl, element #2=w1911:dbl, element #3=w1910:dbl)
            }
            frame 3 {
              n253 = Index Array(array=w1917, index (row) #1=w1921, index (col) #1=0, index (row) #2=w1921, index (col) #2=1, index (row) #3=w1921, index (col) #3=2) -> (element #1=w1919:dbl, element #2=w1920:dbl, element #3=w1918:dbl)
            }
            frame 4 {
              n254 = Index Array(array=w1925, index (row) #1=w1929, index (col) #1=0, index (row) #2=w1929, index (col) #2=1, index (row) #3=w1929, index (col) #3=2) -> (element #1=w1926:dbl, element #2=w1928:dbl, element #3=w1927:dbl)
            }
            frame 5 {
              n255 = Index Array(array=w1933, index (row) #1=w1934, index (col) #1=0, index (row) #2=w1934, index (col) #2=1, index (row) #3=w1934, index (col) #3=2) -> (element #1=w1935:dbl, element #2=w1936:dbl, element #3=w1937:dbl)
            }
            frame 6 {
              n256 = Index Array(array=w1941, index (row) #1=w1945, index (col) #1=0, index (row) #2=w1945, index (col) #2=1, index (row) #3=w1945, index (col) #3=2) -> (element #1=w1942:dbl, element #2=w1944:dbl, element #3=w1943:dbl)
            }
            frame 7 {
              n257 = Index Array(array=w1949, index (row) #1=w1950, index (col) #1=0, index (row) #2=w1950, index (col) #2=1, index (row) #3=w1950, index (col) #3=2) -> (element #1=w1951:dbl, element #2=w1953:dbl, element #3=w1952:dbl)
            }
          }
        }
        frame "East" {
          w1961 = 7
          n258 = case shown="2" w1961 {
            tunnel: [w1965 w1971 w1979 w1987 w1995 w2004 w2011 w2020] -> w1959
            tunnel: [w1967 w1973 w1981 w1988 w1997 w2006 w2013 w2022] -> w1958
            tunnel: [w1966 w1972 w1980 w1989 w1996 w2005 w2012 w2021] -> w1957
            tunnel: w1961 -> [w1969 w1974 w1982 w1990 w1998 w2003 w2014 w2019]
            tunnel: w1960 -> [w1962 w1970 w1978 w1986 w1994 w2002 w2010 w2018]
            frame 0, Default {
              n259 = Index Array(array=w1962, index (row) #1=w1969, index (col) #1=0, index (row) #2=w1969, index (col) #2=1, index (row) #3=w1969, index (col) #3=2) -> (element #1=w1967:dbl, element #2=w1966:dbl, element #3=w1965:dbl)
            }
            frame 1 {
              n260 = Index Array(array=w1970, index (row) #1=w1974, index (col) #1=0, index (row) #2=w1974, index (col) #2=1, index (row) #3=w1974, index (col) #3=2) -> (element #1=w1973:dbl, element #2=w1972:dbl, element #3=w1971:dbl)
            }
            frame 2 {
              n261 = Index Array(array=w1978, index (row) #1=w1982, index (col) #1=0, index (row) #2=w1982, index (col) #2=1, index (row) #3=w1982, index (col) #3=2) -> (element #1=w1981:dbl, element #2=w1980:dbl, element #3=w1979:dbl)
            }
            frame 3 {
              n262 = Index Array(array=w1986, index (row) #1=w1990, index (col) #1=0, index (row) #2=w1990, index (col) #2=1, index (row) #3=w1990, index (col) #3=2) -> (element #1=w1988:dbl, element #2=w1989:dbl, element #3=w1987:dbl)
            }
            frame 4 {
              n263 = Index Array(array=w1994, index (row) #1=w1998, index (col) #1=0, index (row) #2=w1998, index (col) #2=1, index (row) #3=w1998, index (col) #3=2) -> (element #1=w1995:dbl, element #2=w1997:dbl, element #3=w1996:dbl)
            }
            frame 5 {
              n264 = Index Array(array=w2002, index (row) #1=w2003, index (col) #1=0, index (row) #2=w2003, index (col) #2=1, index (row) #3=w2003, index (col) #3=2) -> (element #1=w2004:dbl, element #2=w2005:dbl, element #3=w2006:dbl)
            }
            frame 6 {
              n265 = Index Array(array=w2010, index (row) #1=w2014, index (col) #1=0, index (row) #2=w2014, index (col) #2=1, index (row) #3=w2014, index (col) #3=2) -> (element #1=w2011:dbl, element #2=w2013:dbl, element #3=w2012:dbl)
            }
            frame 7 {
              n266 = Index Array(array=w2018, index (row) #1=w2019, index (col) #1=0, index (row) #2=w2019, index (col) #2=1, index (row) #3=w2019, index (col) #3=2) -> (element #1=w2020:dbl, element #2=w2022:dbl, element #3=w2021:dbl)
            }
          }
        }
        frame "South" {
          w2030 = 4
          n267 = case shown="2" w2030 {
            tunnel: [w2034 w2040 w2048 w2056 w2064 w2073 w2080 w2089] -> w2029
            tunnel: [w2036 w2042 w2050 w2057 w2066 w2075 w2082 w2091] -> w2027
            tunnel: [w2035 w2041 w2049 w2058 w2065 w2074 w2081 w2090] -> w2026
            tunnel: w2030 -> [w2038 w2043 w2051 w2059 w2067 w2072 w2083 w2088]
            tunnel: w2028 -> [w2031 w2039 w2047 w2055 w2063 w2071 w2079 w2087]
            frame 0, Default {
              n268 = Index Array(array=w2031, index (row) #1=w2038, index (col) #1=0, index (row) #2=w2038, index (col) #2=1, index (row) #3=w2038, index (col) #3=2) -> (element #1=w2036:dbl, element #2=w2035:dbl, element #3=w2034:dbl)
            }
            frame 1 {
              n269 = Index Array(array=w2039, index (row) #1=w2043, index (col) #1=0, index (row) #2=w2043, index (col) #2=1, index (row) #3=w2043, index (col) #3=2) -> (element #1=w2042:dbl, element #2=w2041:dbl, element #3=w2040:dbl)
            }
            frame 2 {
              n270 = Index Array(array=w2047, index (row) #1=w2051, index (col) #1=0, index (row) #2=w2051, index (col) #2=1, index (row) #3=w2051, index (col) #3=2) -> (element #1=w2050:dbl, element #2=w2049:dbl, element #3=w2048:dbl)
            }
            frame 3 {
              n271 = Index Array(array=w2055, index (row) #1=w2059, index (col) #1=0, index (row) #2=w2059, index (col) #2=1, index (row) #3=w2059, index (col) #3=2) -> (element #1=w2057:dbl, element #2=w2058:dbl, element #3=w2056:dbl)
            }
            frame 4 {
              n272 = Index Array(array=w2063, index (row) #1=w2067, index (col) #1=0, index (row) #2=w2067, index (col) #2=1, index (row) #3=w2067, index (col) #3=2) -> (element #1=w2064:dbl, element #2=w2066:dbl, element #3=w2065:dbl)
            }
            frame 5 {
              n273 = Index Array(array=w2071, index (row) #1=w2072, index (col) #1=0, index (row) #2=w2072, index (col) #2=1, index (row) #3=w2072, index (col) #3=2) -> (element #1=w2073:dbl, element #2=w2074:dbl, element #3=w2075:dbl)
            }
            frame 6 {
              n274 = Index Array(array=w2079, index (row) #1=w2083, index (col) #1=0, index (row) #2=w2083, index (col) #2=1, index (row) #3=w2083, index (col) #3=2) -> (element #1=w2080:dbl, element #2=w2082:dbl, element #3=w2081:dbl)
            }
            frame 7 {
              n275 = Index Array(array=w2087, index (row) #1=w2088, index (col) #1=0, index (row) #2=w2088, index (col) #2=1, index (row) #3=w2088, index (col) #3=2) -> (element #1=w2089:dbl, element #2=w2091:dbl, element #3=w2090:dbl)
            }
          }
        }
        frame "South west" {
          w2099 = 2
          n276 = case shown="2" w2099 {
            tunnel: [w2103 w2109 w2117 w2125 w2133 w2142 w2149 w2158] -> w2097
            tunnel: [w2105 w2111 w2119 w2126 w2135 w2144 w2151 w2160] -> w2096
            tunnel: [w2104 w2110 w2118 w2127 w2134 w2143 w2150 w2159] -> w2095
            tunnel: w2099 -> [w2107 w2112 w2120 w2128 w2136 w2141 w2152 w2157]
            tunnel: w2098 -> [w2100 w2108 w2116 w2124 w2132 w2140 w2148 w2156]
            frame 0, Default {
              n277 = Index Array(array=w2100, index (row) #1=w2107, index (col) #1=0, index (row) #2=w2107, index (col) #2=1, index (row) #3=w2107, index (col) #3=2) -> (element #1=w2105:dbl, element #2=w2104:dbl, element #3=w2103:dbl)
            }
            frame 1 {
              n278 = Index Array(array=w2108, index (row) #1=w2112, index (col) #1=0, index (row) #2=w2112, index (col) #2=1, index (row) #3=w2112, index (col) #3=2) -> (element #1=w2111:dbl, element #2=w2110:dbl, element #3=w2109:dbl)
            }
            frame 2 {
              n279 = Index Array(array=w2116, index (row) #1=w2120, index (col) #1=0, index (row) #2=w2120, index (col) #2=1, index (row) #3=w2120, index (col) #3=2) -> (element #1=w2119:dbl, element #2=w2118:dbl, element #3=w2117:dbl)
            }
            frame 3 {
              n280 = Index Array(array=w2124, index (row) #1=w2128, index (col) #1=0, index (row) #2=w2128, index (col) #2=1, index (row) #3=w2128, index (col) #3=2) -> (element #1=w2126:dbl, element #2=w2127:dbl, element #3=w2125:dbl)
            }
            frame 4 {
              n281 = Index Array(array=w2132, index (row) #1=w2136, index (col) #1=0, index (row) #2=w2136, index (col) #2=1, index (row) #3=w2136, index (col) #3=2) -> (element #1=w2133:dbl, element #2=w2135:dbl, element #3=w2134:dbl)
            }
            frame 5 {
              n282 = Index Array(array=w2140, index (row) #1=w2141, index (col) #1=0, index (row) #2=w2141, index (col) #2=1, index (row) #3=w2141, index (col) #3=2) -> (element #1=w2142:dbl, element #2=w2143:dbl, element #3=w2144:dbl)
            }
            frame 6 {
              n283 = Index Array(array=w2148, index (row) #1=w2152, index (col) #1=0, index (row) #2=w2152, index (col) #2=1, index (row) #3=w2152, index (col) #3=2) -> (element #1=w2149:dbl, element #2=w2151:dbl, element #3=w2150:dbl)
            }
            frame 7 {
              n284 = Index Array(array=w2156, index (row) #1=w2157, index (col) #1=0, index (row) #2=w2157, index (col) #2=1, index (row) #3=w2157, index (col) #3=2) -> (element #1=w2158:dbl, element #2=w2160:dbl, element #3=w2159:dbl)
            }
          }
        }
        frame "South east" {
          w2168 = 6
          n285 = case shown="2" w2168 {
            tunnel: [w2172 w2178 w2186 w2194 w2202 w2211 w2218 w2227] -> w2167
            tunnel: [w2174 w2180 w2188 w2195 w2204 w2213 w2220 w2229] -> w2166
            tunnel: [w2173 w2179 w2187 w2196 w2203 w2212 w2219 w2228] -> w2165
            tunnel: w2168 -> [w2176 w2181 w2189 w2197 w2205 w2210 w2221 w2226]
            tunnel: w2164 -> [w2169 w2177 w2185 w2193 w2201 w2209 w2217 w2225]
            frame 0, Default {
              n286 = Index Array(array=w2169, index (row) #1=w2176, index (col) #1=0, index (row) #2=w2176, index (col) #2=1, index (row) #3=w2176, index (col) #3=2) -> (element #1=w2174:dbl, element #2=w2173:dbl, element #3=w2172:dbl)
            }
            frame 1 {
              n287 = Index Array(array=w2177, index (row) #1=w2181, index (col) #1=0, index (row) #2=w2181, index (col) #2=1, index (row) #3=w2181, index (col) #3=2) -> (element #1=w2180:dbl, element #2=w2179:dbl, element #3=w2178:dbl)
            }
            frame 2 {
              n288 = Index Array(array=w2185, index (row) #1=w2189, index (col) #1=0, index (row) #2=w2189, index (col) #2=1, index (row) #3=w2189, index (col) #3=2) -> (element #1=w2188:dbl, element #2=w2187:dbl, element #3=w2186:dbl)
            }
            frame 3 {
              n289 = Index Array(array=w2193, index (row) #1=w2197, index (col) #1=0, index (row) #2=w2197, index (col) #2=1, index (row) #3=w2197, index (col) #3=2) -> (element #1=w2195:dbl, element #2=w2196:dbl, element #3=w2194:dbl)
            }
            frame 4 {
              n290 = Index Array(array=w2201, index (row) #1=w2205, index (col) #1=0, index (row) #2=w2205, index (col) #2=1, index (row) #3=w2205, index (col) #3=2) -> (element #1=w2202:dbl, element #2=w2204:dbl, element #3=w2203:dbl)
            }
            frame 5 {
              n291 = Index Array(array=w2209, index (row) #1=w2210, index (col) #1=0, index (row) #2=w2210, index (col) #2=1, index (row) #3=w2210, index (col) #3=2) -> (element #1=w2211:dbl, element #2=w2212:dbl, element #3=w2213:dbl)
            }
            frame 6 {
              n292 = Index Array(array=w2217, index (row) #1=w2221, index (col) #1=0, index (row) #2=w2221, index (col) #2=1, index (row) #3=w2221, index (col) #3=2) -> (element #1=w2218:dbl, element #2=w2220:dbl, element #3=w2219:dbl)
            }
            frame 7 {
              n293 = Index Array(array=w2225, index (row) #1=w2226, index (col) #1=0, index (row) #2=w2226, index (col) #2=1, index (row) #3=w2226, index (col) #3=2) -> (element #1=w2227:dbl, element #2=w2229:dbl, element #3=w2228:dbl)
            }
          }
        }
      }
    }
    frame "East" {
      n294 = case shown="\"North\", Default" w2234 {
        tunnel: [w2241 w2311 w2379 w2446 w2516 w2586 w2654 w2724] -> w2237
        tunnel: [w2240 w2310 w2378 w2447 w2515 w2584 w2653 w2723] -> w2236
        tunnel: [w2239 w2309 w2377 w2445 w2514 w2583 w2652 w2722] -> w2235
        tunnel: w2233 -> [w2238 w2307 w2376 w2448 w2517 w2585 w2655 w2721]
        frame "North", Default {
          w2242 = 4
          n295 = case shown="2" w2242 {
            tunnel: [w2246 w2252 w2260 w2268 w2276 w2285 w2292 w2301] -> w2241
            tunnel: [w2248 w2254 w2262 w2269 w2278 w2287 w2294 w2303] -> w2240
            tunnel: [w2247 w2253 w2261 w2270 w2277 w2286 w2293 w2302] -> w2239
            tunnel: w2242 -> [w2250 w2255 w2263 w2271 w2279 w2284 w2295 w2300]
            tunnel: w2238 -> [w2243 w2251 w2259 w2267 w2275 w2283 w2291 w2299]
            frame 0, Default {
              n296 = Index Array(array=w2243, index (row) #1=w2250, index (col) #1=0, index (row) #2=w2250, index (col) #2=1, index (row) #3=w2250, index (col) #3=2) -> (element #1=w2248:dbl, element #2=w2247:dbl, element #3=w2246:dbl)
            }
            frame 1 {
              n297 = Index Array(array=w2251, index (row) #1=w2255, index (col) #1=0, index (row) #2=w2255, index (col) #2=1, index (row) #3=w2255, index (col) #3=2) -> (element #1=w2254:dbl, element #2=w2253:dbl, element #3=w2252:dbl)
            }
            frame 2 {
              n298 = Index Array(array=w2259, index (row) #1=w2263, index (col) #1=0, index (row) #2=w2263, index (col) #2=1, index (row) #3=w2263, index (col) #3=2) -> (element #1=w2262:dbl, element #2=w2261:dbl, element #3=w2260:dbl)
            }
            frame 3 {
              n299 = Index Array(array=w2267, index (row) #1=w2271, index (col) #1=0, index (row) #2=w2271, index (col) #2=1, index (row) #3=w2271, index (col) #3=2) -> (element #1=w2269:dbl, element #2=w2270:dbl, element #3=w2268:dbl)
            }
            frame 4 {
              n300 = Index Array(array=w2275, index (row) #1=w2279, index (col) #1=0, index (row) #2=w2279, index (col) #2=1, index (row) #3=w2279, index (col) #3=2) -> (element #1=w2276:dbl, element #2=w2278:dbl, element #3=w2277:dbl)
            }
            frame 5 {
              n301 = Index Array(array=w2283, index (row) #1=w2284, index (col) #1=0, index (row) #2=w2284, index (col) #2=1, index (row) #3=w2284, index (col) #3=2) -> (element #1=w2285:dbl, element #2=w2286:dbl, element #3=w2287:dbl)
            }
            frame 6 {
              n302 = Index Array(array=w2291, index (row) #1=w2295, index (col) #1=0, index (row) #2=w2295, index (col) #2=1, index (row) #3=w2295, index (col) #3=2) -> (element #1=w2292:dbl, element #2=w2294:dbl, element #3=w2293:dbl)
            }
            frame 7 {
              n303 = Index Array(array=w2299, index (row) #1=w2300, index (col) #1=0, index (row) #2=w2300, index (col) #2=1, index (row) #3=w2300, index (col) #3=2) -> (element #1=w2301:dbl, element #2=w2303:dbl, element #3=w2302:dbl)
            }
          }
        }
        frame "North east" {
          w2308 = 2
          n304 = case shown="2" w2308 {
            tunnel: [w2315 w2321 w2329 w2337 w2345 w2354 w2361 w2370] -> w2311
            tunnel: [w2317 w2323 w2331 w2338 w2347 w2356 w2363 w2372] -> w2310
            tunnel: [w2316 w2322 w2330 w2339 w2346 w2355 w2362 w2371] -> w2309
            tunnel: w2308 -> [w2319 w2324 w2332 w2340 w2348 w2353 w2364 w2369]
            tunnel: w2307 -> [w2312 w2320 w2328 w2336 w2344 w2352 w2360 w2368]
            frame 0, Default {
              n305 = Index Array(array=w2312, index (row) #1=w2319, index (col) #1=0, index (row) #2=w2319, index (col) #2=1, index (row) #3=w2319, index (col) #3=2) -> (element #1=w2317:dbl, element #2=w2316:dbl, element #3=w2315:dbl)
            }
            frame 1 {
              n306 = Index Array(array=w2320, index (row) #1=w2324, index (col) #1=0, index (row) #2=w2324, index (col) #2=1, index (row) #3=w2324, index (col) #3=2) -> (element #1=w2323:dbl, element #2=w2322:dbl, element #3=w2321:dbl)
            }
            frame 2 {
              n307 = Index Array(array=w2328, index (row) #1=w2332, index (col) #1=0, index (row) #2=w2332, index (col) #2=1, index (row) #3=w2332, index (col) #3=2) -> (element #1=w2331:dbl, element #2=w2330:dbl, element #3=w2329:dbl)
            }
            frame 3 {
              n308 = Index Array(array=w2336, index (row) #1=w2340, index (col) #1=0, index (row) #2=w2340, index (col) #2=1, index (row) #3=w2340, index (col) #3=2) -> (element #1=w2338:dbl, element #2=w2339:dbl, element #3=w2337:dbl)
            }
            frame 4 {
              n309 = Index Array(array=w2344, index (row) #1=w2348, index (col) #1=0, index (row) #2=w2348, index (col) #2=1, index (row) #3=w2348, index (col) #3=2) -> (element #1=w2345:dbl, element #2=w2347:dbl, element #3=w2346:dbl)
            }
            frame 5 {
              n310 = Index Array(array=w2352, index (row) #1=w2353, index (col) #1=0, index (row) #2=w2353, index (col) #2=1, index (row) #3=w2353, index (col) #3=2) -> (element #1=w2354:dbl, element #2=w2355:dbl, element #3=w2356:dbl)
            }
            frame 6 {
              n311 = Index Array(array=w2360, index (row) #1=w2364, index (col) #1=0, index (row) #2=w2364, index (col) #2=1, index (row) #3=w2364, index (col) #3=2) -> (element #1=w2361:dbl, element #2=w2363:dbl, element #3=w2362:dbl)
            }
            frame 7 {
              n312 = Index Array(array=w2368, index (row) #1=w2369, index (col) #1=0, index (row) #2=w2369, index (col) #2=1, index (row) #3=w2369, index (col) #3=2) -> (element #1=w2370:dbl, element #2=w2372:dbl, element #3=w2371:dbl)
            }
          }
        }
        frame "North west" {
          w2380 = 6
          n313 = case shown="2" w2380 {
            tunnel: [w2384 w2390 w2398 w2406 w2414 w2423 w2430 w2439] -> w2379
            tunnel: [w2386 w2392 w2400 w2407 w2416 w2425 w2432 w2441] -> w2378
            tunnel: [w2385 w2391 w2399 w2408 w2415 w2424 w2431 w2440] -> w2377
            tunnel: w2380 -> [w2388 w2393 w2401 w2409 w2417 w2422 w2433 w2438]
            tunnel: w2376 -> [w2381 w2389 w2397 w2405 w2413 w2421 w2429 w2437]
            frame 0, Default {
              n314 = Index Array(array=w2381, index (row) #1=w2388, index (col) #1=0, index (row) #2=w2388, index (col) #2=1, index (row) #3=w2388, index (col) #3=2) -> (element #1=w2386:dbl, element #2=w2385:dbl, element #3=w2384:dbl)
            }
            frame 1 {
              n315 = Index Array(array=w2389, index (row) #1=w2393, index (col) #1=0, index (row) #2=w2393, index (col) #2=1, index (row) #3=w2393, index (col) #3=2) -> (element #1=w2392:dbl, element #2=w2391:dbl, element #3=w2390:dbl)
            }
            frame 2 {
              n316 = Index Array(array=w2397, index (row) #1=w2401, index (col) #1=0, index (row) #2=w2401, index (col) #2=1, index (row) #3=w2401, index (col) #3=2) -> (element #1=w2400:dbl, element #2=w2399:dbl, element #3=w2398:dbl)
            }
            frame 3 {
              n317 = Index Array(array=w2405, index (row) #1=w2409, index (col) #1=0, index (row) #2=w2409, index (col) #2=1, index (row) #3=w2409, index (col) #3=2) -> (element #1=w2407:dbl, element #2=w2408:dbl, element #3=w2406:dbl)
            }
            frame 4 {
              n318 = Index Array(array=w2413, index (row) #1=w2417, index (col) #1=0, index (row) #2=w2417, index (col) #2=1, index (row) #3=w2417, index (col) #3=2) -> (element #1=w2414:dbl, element #2=w2416:dbl, element #3=w2415:dbl)
            }
            frame 5 {
              n319 = Index Array(array=w2421, index (row) #1=w2422, index (col) #1=0, index (row) #2=w2422, index (col) #2=1, index (row) #3=w2422, index (col) #3=2) -> (element #1=w2423:dbl, element #2=w2424:dbl, element #3=w2425:dbl)
            }
            frame 6 {
              n320 = Index Array(array=w2429, index (row) #1=w2433, index (col) #1=0, index (row) #2=w2433, index (col) #2=1, index (row) #3=w2433, index (col) #3=2) -> (element #1=w2430:dbl, element #2=w2432:dbl, element #3=w2431:dbl)
            }
            frame 7 {
              n321 = Index Array(array=w2437, index (row) #1=w2438, index (col) #1=0, index (row) #2=w2438, index (col) #2=1, index (row) #3=w2438, index (col) #3=2) -> (element #1=w2439:dbl, element #2=w2441:dbl, element #3=w2440:dbl)
            }
          }
        }
        frame "West" {
          w2449 = 7
          n322 = case shown="2" w2449 {
            tunnel: [w2453 w2459 w2467 w2475 w2483 w2492 w2499 w2508] -> w2446
            tunnel: [w2455 w2461 w2469 w2476 w2485 w2494 w2501 w2510] -> w2447
            tunnel: [w2454 w2460 w2468 w2477 w2484 w2493 w2500 w2509] -> w2445
            tunnel: w2449 -> [w2457 w2462 w2470 w2478 w2486 w2491 w2502 w2507]
            tunnel: w2448 -> [w2450 w2458 w2466 w2474 w2482 w2490 w2498 w2506]
            frame 0, Default {
              n323 = Index Array(array=w2450, index (row) #1=w2457, index (col) #1=0, index (row) #2=w2457, index (col) #2=1, index (row) #3=w2457, index (col) #3=2) -> (element #1=w2455:dbl, element #2=w2454:dbl, element #3=w2453:dbl)
            }
            frame 1 {
              n324 = Index Array(array=w2458, index (row) #1=w2462, index (col) #1=0, index (row) #2=w2462, index (col) #2=1, index (row) #3=w2462, index (col) #3=2) -> (element #1=w2461:dbl, element #2=w2460:dbl, element #3=w2459:dbl)
            }
            frame 2 {
              n325 = Index Array(array=w2466, index (row) #1=w2470, index (col) #1=0, index (row) #2=w2470, index (col) #2=1, index (row) #3=w2470, index (col) #3=2) -> (element #1=w2469:dbl, element #2=w2468:dbl, element #3=w2467:dbl)
            }
            frame 3 {
              n326 = Index Array(array=w2474, index (row) #1=w2478, index (col) #1=0, index (row) #2=w2478, index (col) #2=1, index (row) #3=w2478, index (col) #3=2) -> (element #1=w2476:dbl, element #2=w2477:dbl, element #3=w2475:dbl)
            }
            frame 4 {
              n327 = Index Array(array=w2482, index (row) #1=w2486, index (col) #1=0, index (row) #2=w2486, index (col) #2=1, index (row) #3=w2486, index (col) #3=2) -> (element #1=w2483:dbl, element #2=w2485:dbl, element #3=w2484:dbl)
            }
            frame 5 {
              n328 = Index Array(array=w2490, index (row) #1=w2491, index (col) #1=0, index (row) #2=w2491, index (col) #2=1, index (row) #3=w2491, index (col) #3=2) -> (element #1=w2492:dbl, element #2=w2493:dbl, element #3=w2494:dbl)
            }
            frame 6 {
              n329 = Index Array(array=w2498, index (row) #1=w2502, index (col) #1=0, index (row) #2=w2502, index (col) #2=1, index (row) #3=w2502, index (col) #3=2) -> (element #1=w2499:dbl, element #2=w2501:dbl, element #3=w2500:dbl)
            }
            frame 7 {
              n330 = Index Array(array=w2506, index (row) #1=w2507, index (col) #1=0, index (row) #2=w2507, index (col) #2=1, index (row) #3=w2507, index (col) #3=2) -> (element #1=w2508:dbl, element #2=w2510:dbl, element #3=w2509:dbl)
            }
          }
        }
        frame "East" {
          w2518 = 0
          n331 = case shown="2" w2518 {
            tunnel: [w2522 w2528 w2536 w2544 w2552 w2561 w2568 w2577] -> w2516
            tunnel: [w2524 w2530 w2538 w2545 w2554 w2563 w2570 w2579] -> w2515
            tunnel: [w2523 w2529 w2537 w2546 w2553 w2562 w2569 w2578] -> w2514
            tunnel: w2518 -> [w2526 w2531 w2539 w2547 w2555 w2560 w2571 w2576]
            tunnel: w2517 -> [w2519 w2527 w2535 w2543 w2551 w2559 w2567 w2575]
            frame 0, Default {
              n332 = Index Array(array=w2519, index (row) #1=w2526, index (col) #1=0, index (row) #2=w2526, index (col) #2=1, index (row) #3=w2526, index (col) #3=2) -> (element #1=w2524:dbl, element #2=w2523:dbl, element #3=w2522:dbl)
            }
            frame 1 {
              n333 = Index Array(array=w2527, index (row) #1=w2531, index (col) #1=0, index (row) #2=w2531, index (col) #2=1, index (row) #3=w2531, index (col) #3=2) -> (element #1=w2530:dbl, element #2=w2529:dbl, element #3=w2528:dbl)
            }
            frame 2 {
              n334 = Index Array(array=w2535, index (row) #1=w2539, index (col) #1=0, index (row) #2=w2539, index (col) #2=1, index (row) #3=w2539, index (col) #3=2) -> (element #1=w2538:dbl, element #2=w2537:dbl, element #3=w2536:dbl)
            }
            frame 3 {
              n335 = Index Array(array=w2543, index (row) #1=w2547, index (col) #1=0, index (row) #2=w2547, index (col) #2=1, index (row) #3=w2547, index (col) #3=2) -> (element #1=w2545:dbl, element #2=w2546:dbl, element #3=w2544:dbl)
            }
            frame 4 {
              n336 = Index Array(array=w2551, index (row) #1=w2555, index (col) #1=0, index (row) #2=w2555, index (col) #2=1, index (row) #3=w2555, index (col) #3=2) -> (element #1=w2552:dbl, element #2=w2554:dbl, element #3=w2553:dbl)
            }
            frame 5 {
              n337 = Index Array(array=w2559, index (row) #1=w2560, index (col) #1=0, index (row) #2=w2560, index (col) #2=1, index (row) #3=w2560, index (col) #3=2) -> (element #1=w2561:dbl, element #2=w2562:dbl, element #3=w2563:dbl)
            }
            frame 6 {
              n338 = Index Array(array=w2567, index (row) #1=w2571, index (col) #1=0, index (row) #2=w2571, index (col) #2=1, index (row) #3=w2571, index (col) #3=2) -> (element #1=w2568:dbl, element #2=w2570:dbl, element #3=w2569:dbl)
            }
            frame 7 {
              n339 = Index Array(array=w2575, index (row) #1=w2576, index (col) #1=0, index (row) #2=w2576, index (col) #2=1, index (row) #3=w2576, index (col) #3=2) -> (element #1=w2577:dbl, element #2=w2579:dbl, element #3=w2578:dbl)
            }
          }
        }
        frame "South" {
          w2587 = 3
          n340 = case shown="2" w2587 {
            tunnel: [w2591 w2597 w2605 w2613 w2621 w2630 w2637 w2646] -> w2586
            tunnel: [w2593 w2599 w2607 w2614 w2623 w2632 w2639 w2648] -> w2584
            tunnel: [w2592 w2598 w2606 w2615 w2622 w2631 w2638 w2647] -> w2583
            tunnel: w2587 -> [w2595 w2600 w2608 w2616 w2624 w2629 w2640 w2645]
            tunnel: w2585 -> [w2588 w2596 w2604 w2612 w2620 w2628 w2636 w2644]
            frame 0, Default {
              n341 = Index Array(array=w2588, index (row) #1=w2595, index (col) #1=0, index (row) #2=w2595, index (col) #2=1, index (row) #3=w2595, index (col) #3=2) -> (element #1=w2593:dbl, element #2=w2592:dbl, element #3=w2591:dbl)
            }
            frame 1 {
              n342 = Index Array(array=w2596, index (row) #1=w2600, index (col) #1=0, index (row) #2=w2600, index (col) #2=1, index (row) #3=w2600, index (col) #3=2) -> (element #1=w2599:dbl, element #2=w2598:dbl, element #3=w2597:dbl)
            }
            frame 2 {
              n343 = Index Array(array=w2604, index (row) #1=w2608, index (col) #1=0, index (row) #2=w2608, index (col) #2=1, index (row) #3=w2608, index (col) #3=2) -> (element #1=w2607:dbl, element #2=w2606:dbl, element #3=w2605:dbl)
            }
            frame 3 {
              n344 = Index Array(array=w2612, index (row) #1=w2616, index (col) #1=0, index (row) #2=w2616, index (col) #2=1, index (row) #3=w2616, index (col) #3=2) -> (element #1=w2614:dbl, element #2=w2615:dbl, element #3=w2613:dbl)
            }
            frame 4 {
              n345 = Index Array(array=w2620, index (row) #1=w2624, index (col) #1=0, index (row) #2=w2624, index (col) #2=1, index (row) #3=w2624, index (col) #3=2) -> (element #1=w2621:dbl, element #2=w2623:dbl, element #3=w2622:dbl)
            }
            frame 5 {
              n346 = Index Array(array=w2628, index (row) #1=w2629, index (col) #1=0, index (row) #2=w2629, index (col) #2=1, index (row) #3=w2629, index (col) #3=2) -> (element #1=w2630:dbl, element #2=w2631:dbl, element #3=w2632:dbl)
            }
            frame 6 {
              n347 = Index Array(array=w2636, index (row) #1=w2640, index (col) #1=0, index (row) #2=w2640, index (col) #2=1, index (row) #3=w2640, index (col) #3=2) -> (element #1=w2637:dbl, element #2=w2639:dbl, element #3=w2638:dbl)
            }
            frame 7 {
              n348 = Index Array(array=w2644, index (row) #1=w2645, index (col) #1=0, index (row) #2=w2645, index (col) #2=1, index (row) #3=w2645, index (col) #3=2) -> (element #1=w2646:dbl, element #2=w2648:dbl, element #3=w2647:dbl)
            }
          }
        }
        frame "South west" {
          w2656 = 5
          n349 = case shown="2" w2656 {
            tunnel: [w2660 w2666 w2674 w2682 w2690 w2699 w2706 w2715] -> w2654
            tunnel: [w2662 w2668 w2676 w2683 w2692 w2701 w2708 w2717] -> w2653
            tunnel: [w2661 w2667 w2675 w2684 w2691 w2700 w2707 w2716] -> w2652
            tunnel: w2656 -> [w2664 w2669 w2677 w2685 w2693 w2698 w2709 w2714]
            tunnel: w2655 -> [w2657 w2665 w2673 w2681 w2689 w2697 w2705 w2713]
            frame 0, Default {
              n350 = Index Array(array=w2657, index (row) #1=w2664, index (col) #1=0, index (row) #2=w2664, index (col) #2=1, index (row) #3=w2664, index (col) #3=2) -> (element #1=w2662:dbl, element #2=w2661:dbl, element #3=w2660:dbl)
            }
            frame 1 {
              n351 = Index Array(array=w2665, index (row) #1=w2669, index (col) #1=0, index (row) #2=w2669, index (col) #2=1, index (row) #3=w2669, index (col) #3=2) -> (element #1=w2668:dbl, element #2=w2667:dbl, element #3=w2666:dbl)
            }
            frame 2 {
              n352 = Index Array(array=w2673, index (row) #1=w2677, index (col) #1=0, index (row) #2=w2677, index (col) #2=1, index (row) #3=w2677, index (col) #3=2) -> (element #1=w2676:dbl, element #2=w2675:dbl, element #3=w2674:dbl)
            }
            frame 3 {
              n353 = Index Array(array=w2681, index (row) #1=w2685, index (col) #1=0, index (row) #2=w2685, index (col) #2=1, index (row) #3=w2685, index (col) #3=2) -> (element #1=w2683:dbl, element #2=w2684:dbl, element #3=w2682:dbl)
            }
            frame 4 {
              n354 = Index Array(array=w2689, index (row) #1=w2693, index (col) #1=0, index (row) #2=w2693, index (col) #2=1, index (row) #3=w2693, index (col) #3=2) -> (element #1=w2690:dbl, element #2=w2692:dbl, element #3=w2691:dbl)
            }
            frame 5 {
              n355 = Index Array(array=w2697, index (row) #1=w2698, index (col) #1=0, index (row) #2=w2698, index (col) #2=1, index (row) #3=w2698, index (col) #3=2) -> (element #1=w2699:dbl, element #2=w2700:dbl, element #3=w2701:dbl)
            }
            frame 6 {
              n356 = Index Array(array=w2705, index (row) #1=w2709, index (col) #1=0, index (row) #2=w2709, index (col) #2=1, index (row) #3=w2709, index (col) #3=2) -> (element #1=w2706:dbl, element #2=w2708:dbl, element #3=w2707:dbl)
            }
            frame 7 {
              n357 = Index Array(array=w2713, index (row) #1=w2714, index (col) #1=0, index (row) #2=w2714, index (col) #2=1, index (row) #3=w2714, index (col) #3=2) -> (element #1=w2715:dbl, element #2=w2717:dbl, element #3=w2716:dbl)
            }
          }
        }
        frame "South east" {
          w2725 = 1
          n358 = case shown="2" w2725 {
            tunnel: [w2729 w2735 w2743 w2751 w2759 w2768 w2775 w2784] -> w2724
            tunnel: [w2731 w2737 w2745 w2752 w2761 w2770 w2777 w2786] -> w2723
            tunnel: [w2730 w2736 w2744 w2753 w2760 w2769 w2776 w2785] -> w2722
            tunnel: w2725 -> [w2733 w2738 w2746 w2754 w2762 w2767 w2778 w2783]
            tunnel: w2721 -> [w2726 w2734 w2742 w2750 w2758 w2766 w2774 w2782]
            frame 0, Default {
              n359 = Index Array(array=w2726, index (row) #1=w2733, index (col) #1=0, index (row) #2=w2733, index (col) #2=1, index (row) #3=w2733, index (col) #3=2) -> (element #1=w2731:dbl, element #2=w2730:dbl, element #3=w2729:dbl)
            }
            frame 1 {
              n360 = Index Array(array=w2734, index (row) #1=w2738, index (col) #1=0, index (row) #2=w2738, index (col) #2=1, index (row) #3=w2738, index (col) #3=2) -> (element #1=w2737:dbl, element #2=w2736:dbl, element #3=w2735:dbl)
            }
            frame 2 {
              n361 = Index Array(array=w2742, index (row) #1=w2746, index (col) #1=0, index (row) #2=w2746, index (col) #2=1, index (row) #3=w2746, index (col) #3=2) -> (element #1=w2745:dbl, element #2=w2744:dbl, element #3=w2743:dbl)
            }
            frame 3 {
              n362 = Index Array(array=w2750, index (row) #1=w2754, index (col) #1=0, index (row) #2=w2754, index (col) #2=1, index (row) #3=w2754, index (col) #3=2) -> (element #1=w2752:dbl, element #2=w2753:dbl, element #3=w2751:dbl)
            }
            frame 4 {
              n363 = Index Array(array=w2758, index (row) #1=w2762, index (col) #1=0, index (row) #2=w2762, index (col) #2=1, index (row) #3=w2762, index (col) #3=2) -> (element #1=w2759:dbl, element #2=w2761:dbl, element #3=w2760:dbl)
            }
            frame 5 {
              n364 = Index Array(array=w2766, index (row) #1=w2767, index (col) #1=0, index (row) #2=w2767, index (col) #2=1, index (row) #3=w2767, index (col) #3=2) -> (element #1=w2768:dbl, element #2=w2769:dbl, element #3=w2770:dbl)
            }
            frame 6 {
              n365 = Index Array(array=w2774, index (row) #1=w2778, index (col) #1=0, index (row) #2=w2778, index (col) #2=1, index (row) #3=w2778, index (col) #3=2) -> (element #1=w2775:dbl, element #2=w2777:dbl, element #3=w2776:dbl)
            }
            frame 7 {
              n366 = Index Array(array=w2782, index (row) #1=w2783, index (col) #1=0, index (row) #2=w2783, index (col) #2=1, index (row) #3=w2783, index (col) #3=2) -> (element #1=w2784:dbl, element #2=w2786:dbl, element #3=w2785:dbl)
            }
          }
        }
      }
    }
    frame "South" {
      n367 = case shown="\"North\", Default" w2791 {
        tunnel: [w2798 w2868 w2936 w3003 w3073 w3143 w3211 w3281] -> w2794
        tunnel: [w2797 w2867 w2935 w3004 w3072 w3141 w3210 w3280] -> w2793
        tunnel: [w2796 w2866 w2934 w3002 w3071 w3140 w3209 w3279] -> w2792
        tunnel: w2790 -> [w2795 w2864 w2933 w3005 w3074 w3142 w3212 w3278]
        frame "North", Default {
          w2799 = 7
          n368 = case shown="2" w2799 {
            tunnel: [w2803 w2809 w2817 w2825 w2833 w2842 w2849 w2858] -> w2798
            tunnel: [w2805 w2811 w2819 w2826 w2835 w2844 w2851 w2860] -> w2797
            tunnel: [w2804 w2810 w2818 w2827 w2834 w2843 w2850 w2859] -> w2796
            tunnel: w2799 -> [w2807 w2812 w2820 w2828 w2836 w2841 w2852 w2857]
            tunnel: w2795 -> [w2800 w2808 w2816 w2824 w2832 w2840 w2848 w2856]
            frame 0, Default {
              n369 = Index Array(array=w2800, index (row) #1=w2807, index (col) #1=0, index (row) #2=w2807, index (col) #2=1, index (row) #3=w2807, index (col) #3=2) -> (element #1=w2805:dbl, element #2=w2804:dbl, element #3=w2803:dbl)
            }
            frame 1 {
              n370 = Index Array(array=w2808, index (row) #1=w2812, index (col) #1=0, index (row) #2=w2812, index (col) #2=1, index (row) #3=w2812, index (col) #3=2) -> (element #1=w2811:dbl, element #2=w2810:dbl, element #3=w2809:dbl)
            }
            frame 2 {
              n371 = Index Array(array=w2816, index (row) #1=w2820, index (col) #1=0, index (row) #2=w2820, index (col) #2=1, index (row) #3=w2820, index (col) #3=2) -> (element #1=w2819:dbl, element #2=w2818:dbl, element #3=w2817:dbl)
            }
            frame 3 {
              n372 = Index Array(array=w2824, index (row) #1=w2828, index (col) #1=0, index (row) #2=w2828, index (col) #2=1, index (row) #3=w2828, index (col) #3=2) -> (element #1=w2826:dbl, element #2=w2827:dbl, element #3=w2825:dbl)
            }
            frame 4 {
              n373 = Index Array(array=w2832, index (row) #1=w2836, index (col) #1=0, index (row) #2=w2836, index (col) #2=1, index (row) #3=w2836, index (col) #3=2) -> (element #1=w2833:dbl, element #2=w2835:dbl, element #3=w2834:dbl)
            }
            frame 5 {
              n374 = Index Array(array=w2840, index (row) #1=w2841, index (col) #1=0, index (row) #2=w2841, index (col) #2=1, index (row) #3=w2841, index (col) #3=2) -> (element #1=w2842:dbl, element #2=w2843:dbl, element #3=w2844:dbl)
            }
            frame 6 {
              n375 = Index Array(array=w2848, index (row) #1=w2852, index (col) #1=0, index (row) #2=w2852, index (col) #2=1, index (row) #3=w2852, index (col) #3=2) -> (element #1=w2849:dbl, element #2=w2851:dbl, element #3=w2850:dbl)
            }
            frame 7 {
              n376 = Index Array(array=w2856, index (row) #1=w2857, index (col) #1=0, index (row) #2=w2857, index (col) #2=1, index (row) #3=w2857, index (col) #3=2) -> (element #1=w2858:dbl, element #2=w2860:dbl, element #3=w2859:dbl)
            }
          }
        }
        frame "North east" {
          w2865 = 6
          n377 = case shown="2" w2865 {
            tunnel: [w2872 w2878 w2886 w2894 w2902 w2911 w2918 w2927] -> w2868
            tunnel: [w2874 w2880 w2888 w2895 w2904 w2913 w2920 w2929] -> w2867
            tunnel: [w2873 w2879 w2887 w2896 w2903 w2912 w2919 w2928] -> w2866
            tunnel: w2865 -> [w2876 w2881 w2889 w2897 w2905 w2910 w2921 w2926]
            tunnel: w2864 -> [w2869 w2877 w2885 w2893 w2901 w2909 w2917 w2925]
            frame 0, Default {
              n378 = Index Array(array=w2869, index (row) #1=w2876, index (col) #1=0, index (row) #2=w2876, index (col) #2=1, index (row) #3=w2876, index (col) #3=2) -> (element #1=w2874:dbl, element #2=w2873:dbl, element #3=w2872:dbl)
            }
            frame 1 {
              n379 = Index Array(array=w2877, index (row) #1=w2881, index (col) #1=0, index (row) #2=w2881, index (col) #2=1, index (row) #3=w2881, index (col) #3=2) -> (element #1=w2880:dbl, element #2=w2879:dbl, element #3=w2878:dbl)
            }
            frame 2 {
              n380 = Index Array(array=w2885, index (row) #1=w2889, index (col) #1=0, index (row) #2=w2889, index (col) #2=1, index (row) #3=w2889, index (col) #3=2) -> (element #1=w2888:dbl, element #2=w2887:dbl, element #3=w2886:dbl)
            }
            frame 3 {
              n381 = Index Array(array=w2893, index (row) #1=w2897, index (col) #1=0, index (row) #2=w2897, index (col) #2=1, index (row) #3=w2897, index (col) #3=2) -> (element #1=w2895:dbl, element #2=w2896:dbl, element #3=w2894:dbl)
            }
            frame 4 {
              n382 = Index Array(array=w2901, index (row) #1=w2905, index (col) #1=0, index (row) #2=w2905, index (col) #2=1, index (row) #3=w2905, index (col) #3=2) -> (element #1=w2902:dbl, element #2=w2904:dbl, element #3=w2903:dbl)
            }
            frame 5 {
              n383 = Index Array(array=w2909, index (row) #1=w2910, index (col) #1=0, index (row) #2=w2910, index (col) #2=1, index (row) #3=w2910, index (col) #3=2) -> (element #1=w2911:dbl, element #2=w2912:dbl, element #3=w2913:dbl)
            }
            frame 6 {
              n384 = Index Array(array=w2917, index (row) #1=w2921, index (col) #1=0, index (row) #2=w2921, index (col) #2=1, index (row) #3=w2921, index (col) #3=2) -> (element #1=w2918:dbl, element #2=w2920:dbl, element #3=w2919:dbl)
            }
            frame 7 {
              n385 = Index Array(array=w2925, index (row) #1=w2926, index (col) #1=0, index (row) #2=w2926, index (col) #2=1, index (row) #3=w2926, index (col) #3=2) -> (element #1=w2927:dbl, element #2=w2929:dbl, element #3=w2928:dbl)
            }
          }
        }
        frame "North west" {
          w2937 = 5
          n386 = case shown="2" w2937 {
            tunnel: [w2941 w2947 w2955 w2963 w2971 w2980 w2987 w2996] -> w2936
            tunnel: [w2943 w2949 w2957 w2964 w2973 w2982 w2989 w2998] -> w2935
            tunnel: [w2942 w2948 w2956 w2965 w2972 w2981 w2988 w2997] -> w2934
            tunnel: w2937 -> [w2945 w2950 w2958 w2966 w2974 w2979 w2990 w2995]
            tunnel: w2933 -> [w2938 w2946 w2954 w2962 w2970 w2978 w2986 w2994]
            frame 0, Default {
              n387 = Index Array(array=w2938, index (row) #1=w2945, index (col) #1=0, index (row) #2=w2945, index (col) #2=1, index (row) #3=w2945, index (col) #3=2) -> (element #1=w2943:dbl, element #2=w2942:dbl, element #3=w2941:dbl)
            }
            frame 1 {
              n388 = Index Array(array=w2946, index (row) #1=w2950, index (col) #1=0, index (row) #2=w2950, index (col) #2=1, index (row) #3=w2950, index (col) #3=2) -> (element #1=w2949:dbl, element #2=w2948:dbl, element #3=w2947:dbl)
            }
            frame 2 {
              n389 = Index Array(array=w2954, index (row) #1=w2958, index (col) #1=0, index (row) #2=w2958, index (col) #2=1, index (row) #3=w2958, index (col) #3=2) -> (element #1=w2957:dbl, element #2=w2956:dbl, element #3=w2955:dbl)
            }
            frame 3 {
              n390 = Index Array(array=w2962, index (row) #1=w2966, index (col) #1=0, index (row) #2=w2966, index (col) #2=1, index (row) #3=w2966, index (col) #3=2) -> (element #1=w2964:dbl, element #2=w2965:dbl, element #3=w2963:dbl)
            }
            frame 4 {
              n391 = Index Array(array=w2970, index (row) #1=w2974, index (col) #1=0, index (row) #2=w2974, index (col) #2=1, index (row) #3=w2974, index (col) #3=2) -> (element #1=w2971:dbl, element #2=w2973:dbl, element #3=w2972:dbl)
            }
            frame 5 {
              n392 = Index Array(array=w2978, index (row) #1=w2979, index (col) #1=0, index (row) #2=w2979, index (col) #2=1, index (row) #3=w2979, index (col) #3=2) -> (element #1=w2980:dbl, element #2=w2981:dbl, element #3=w2982:dbl)
            }
            frame 6 {
              n393 = Index Array(array=w2986, index (row) #1=w2990, index (col) #1=0, index (row) #2=w2990, index (col) #2=1, index (row) #3=w2990, index (col) #3=2) -> (element #1=w2987:dbl, element #2=w2989:dbl, element #3=w2988:dbl)
            }
            frame 7 {
              n394 = Index Array(array=w2994, index (row) #1=w2995, index (col) #1=0, index (row) #2=w2995, index (col) #2=1, index (row) #3=w2995, index (col) #3=2) -> (element #1=w2996:dbl, element #2=w2998:dbl, element #3=w2997:dbl)
            }
          }
        }
        frame "West" {
          w3006 = 3
          n395 = case shown="2" w3006 {
            tunnel: [w3010 w3016 w3024 w3032 w3040 w3049 w3056 w3065] -> w3003
            tunnel: [w3012 w3018 w3026 w3033 w3042 w3051 w3058 w3067] -> w3004
            tunnel: [w3011 w3017 w3025 w3034 w3041 w3050 w3057 w3066] -> w3002
            tunnel: w3006 -> [w3014 w3019 w3027 w3035 w3043 w3048 w3059 w3064]
            tunnel: w3005 -> [w3007 w3015 w3023 w3031 w3039 w3047 w3055 w3063]
            frame 0, Default {
              n396 = Index Array(array=w3007, index (row) #1=w3014, index (col) #1=0, index (row) #2=w3014, index (col) #2=1, index (row) #3=w3014, index (col) #3=2) -> (element #1=w3012:dbl, element #2=w3011:dbl, element #3=w3010:dbl)
            }
            frame 1 {
              n397 = Index Array(array=w3015, index (row) #1=w3019, index (col) #1=0, index (row) #2=w3019, index (col) #2=1, index (row) #3=w3019, index (col) #3=2) -> (element #1=w3018:dbl, element #2=w3017:dbl, element #3=w3016:dbl)
            }
            frame 2 {
              n398 = Index Array(array=w3023, index (row) #1=w3027, index (col) #1=0, index (row) #2=w3027, index (col) #2=1, index (row) #3=w3027, index (col) #3=2) -> (element #1=w3026:dbl, element #2=w3025:dbl, element #3=w3024:dbl)
            }
            frame 3 {
              n399 = Index Array(array=w3031, index (row) #1=w3035, index (col) #1=0, index (row) #2=w3035, index (col) #2=1, index (row) #3=w3035, index (col) #3=2) -> (element #1=w3033:dbl, element #2=w3034:dbl, element #3=w3032:dbl)
            }
            frame 4 {
              n400 = Index Array(array=w3039, index (row) #1=w3043, index (col) #1=0, index (row) #2=w3043, index (col) #2=1, index (row) #3=w3043, index (col) #3=2) -> (element #1=w3040:dbl, element #2=w3042:dbl, element #3=w3041:dbl)
            }
            frame 5 {
              n401 = Index Array(array=w3047, index (row) #1=w3048, index (col) #1=0, index (row) #2=w3048, index (col) #2=1, index (row) #3=w3048, index (col) #3=2) -> (element #1=w3049:dbl, element #2=w3050:dbl, element #3=w3051:dbl)
            }
            frame 6 {
              n402 = Index Array(array=w3055, index (row) #1=w3059, index (col) #1=0, index (row) #2=w3059, index (col) #2=1, index (row) #3=w3059, index (col) #3=2) -> (element #1=w3056:dbl, element #2=w3058:dbl, element #3=w3057:dbl)
            }
            frame 7 {
              n403 = Index Array(array=w3063, index (row) #1=w3064, index (col) #1=0, index (row) #2=w3064, index (col) #2=1, index (row) #3=w3064, index (col) #3=2) -> (element #1=w3065:dbl, element #2=w3067:dbl, element #3=w3066:dbl)
            }
          }
        }
        frame "East" {
          w3075 = 4
          n404 = case shown="2" w3075 {
            tunnel: [w3079 w3085 w3093 w3101 w3109 w3118 w3125 w3134] -> w3073
            tunnel: [w3081 w3087 w3095 w3102 w3111 w3120 w3127 w3136] -> w3072
            tunnel: [w3080 w3086 w3094 w3103 w3110 w3119 w3126 w3135] -> w3071
            tunnel: w3075 -> [w3083 w3088 w3096 w3104 w3112 w3117 w3128 w3133]
            tunnel: w3074 -> [w3076 w3084 w3092 w3100 w3108 w3116 w3124 w3132]
            frame 0, Default {
              n405 = Index Array(array=w3076, index (row) #1=w3083, index (col) #1=0, index (row) #2=w3083, index (col) #2=1, index (row) #3=w3083, index (col) #3=2) -> (element #1=w3081:dbl, element #2=w3080:dbl, element #3=w3079:dbl)
            }
            frame 1 {
              n406 = Index Array(array=w3084, index (row) #1=w3088, index (col) #1=0, index (row) #2=w3088, index (col) #2=1, index (row) #3=w3088, index (col) #3=2) -> (element #1=w3087:dbl, element #2=w3086:dbl, element #3=w3085:dbl)
            }
            frame 2 {
              n407 = Index Array(array=w3092, index (row) #1=w3096, index (col) #1=0, index (row) #2=w3096, index (col) #2=1, index (row) #3=w3096, index (col) #3=2) -> (element #1=w3095:dbl, element #2=w3094:dbl, element #3=w3093:dbl)
            }
            frame 3 {
              n408 = Index Array(array=w3100, index (row) #1=w3104, index (col) #1=0, index (row) #2=w3104, index (col) #2=1, index (row) #3=w3104, index (col) #3=2) -> (element #1=w3102:dbl, element #2=w3103:dbl, element #3=w3101:dbl)
            }
            frame 4 {
              n409 = Index Array(array=w3108, index (row) #1=w3112, index (col) #1=0, index (row) #2=w3112, index (col) #2=1, index (row) #3=w3112, index (col) #3=2) -> (element #1=w3109:dbl, element #2=w3111:dbl, element #3=w3110:dbl)
            }
            frame 5 {
              n410 = Index Array(array=w3116, index (row) #1=w3117, index (col) #1=0, index (row) #2=w3117, index (col) #2=1, index (row) #3=w3117, index (col) #3=2) -> (element #1=w3118:dbl, element #2=w3119:dbl, element #3=w3120:dbl)
            }
            frame 6 {
              n411 = Index Array(array=w3124, index (row) #1=w3128, index (col) #1=0, index (row) #2=w3128, index (col) #2=1, index (row) #3=w3128, index (col) #3=2) -> (element #1=w3125:dbl, element #2=w3127:dbl, element #3=w3126:dbl)
            }
            frame 7 {
              n412 = Index Array(array=w3132, index (row) #1=w3133, index (col) #1=0, index (row) #2=w3133, index (col) #2=1, index (row) #3=w3133, index (col) #3=2) -> (element #1=w3134:dbl, element #2=w3136:dbl, element #3=w3135:dbl)
            }
          }
        }
        frame "South" {
          w3144 = 0
          n413 = case shown="2" w3144 {
            tunnel: [w3148 w3154 w3162 w3170 w3178 w3187 w3194 w3203] -> w3143
            tunnel: [w3150 w3156 w3164 w3171 w3180 w3189 w3196 w3205] -> w3141
            tunnel: [w3149 w3155 w3163 w3172 w3179 w3188 w3195 w3204] -> w3140
            tunnel: w3144 -> [w3152 w3157 w3165 w3173 w3181 w3186 w3197 w3202]
            tunnel: w3142 -> [w3145 w3153 w3161 w3169 w3177 w3185 w3193 w3201]
            frame 0, Default {
              n414 = Index Array(array=w3145, index (row) #1=w3152, index (col) #1=0, index (row) #2=w3152, index (col) #2=1, index (row) #3=w3152, index (col) #3=2) -> (element #1=w3150:dbl, element #2=w3149:dbl, element #3=w3148:dbl)
            }
            frame 1 {
              n415 = Index Array(array=w3153, index (row) #1=w3157, index (col) #1=0, index (row) #2=w3157, index (col) #2=1, index (row) #3=w3157, index (col) #3=2) -> (element #1=w3156:dbl, element #2=w3155:dbl, element #3=w3154:dbl)
            }
            frame 2 {
              n416 = Index Array(array=w3161, index (row) #1=w3165, index (col) #1=0, index (row) #2=w3165, index (col) #2=1, index (row) #3=w3165, index (col) #3=2) -> (element #1=w3164:dbl, element #2=w3163:dbl, element #3=w3162:dbl)
            }
            frame 3 {
              n417 = Index Array(array=w3169, index (row) #1=w3173, index (col) #1=0, index (row) #2=w3173, index (col) #2=1, index (row) #3=w3173, index (col) #3=2) -> (element #1=w3171:dbl, element #2=w3172:dbl, element #3=w3170:dbl)
            }
            frame 4 {
              n418 = Index Array(array=w3177, index (row) #1=w3181, index (col) #1=0, index (row) #2=w3181, index (col) #2=1, index (row) #3=w3181, index (col) #3=2) -> (element #1=w3178:dbl, element #2=w3180:dbl, element #3=w3179:dbl)
            }
            frame 5 {
              n419 = Index Array(array=w3185, index (row) #1=w3186, index (col) #1=0, index (row) #2=w3186, index (col) #2=1, index (row) #3=w3186, index (col) #3=2) -> (element #1=w3187:dbl, element #2=w3188:dbl, element #3=w3189:dbl)
            }
            frame 6 {
              n420 = Index Array(array=w3193, index (row) #1=w3197, index (col) #1=0, index (row) #2=w3197, index (col) #2=1, index (row) #3=w3197, index (col) #3=2) -> (element #1=w3194:dbl, element #2=w3196:dbl, element #3=w3195:dbl)
            }
            frame 7 {
              n421 = Index Array(array=w3201, index (row) #1=w3202, index (col) #1=0, index (row) #2=w3202, index (col) #2=1, index (row) #3=w3202, index (col) #3=2) -> (element #1=w3203:dbl, element #2=w3205:dbl, element #3=w3204:dbl)
            }
          }
        }
        frame "South west" {
          w3213 = 1
          n422 = case shown="2" w3213 {
            tunnel: [w3217 w3223 w3231 w3239 w3247 w3256 w3263 w3272] -> w3211
            tunnel: [w3219 w3225 w3233 w3240 w3249 w3258 w3265 w3274] -> w3210
            tunnel: [w3218 w3224 w3232 w3241 w3248 w3257 w3264 w3273] -> w3209
            tunnel: w3213 -> [w3221 w3226 w3234 w3242 w3250 w3255 w3266 w3271]
            tunnel: w3212 -> [w3214 w3222 w3230 w3238 w3246 w3254 w3262 w3270]
            frame 0, Default {
              n423 = Index Array(array=w3214, index (row) #1=w3221, index (col) #1=0, index (row) #2=w3221, index (col) #2=1, index (row) #3=w3221, index (col) #3=2) -> (element #1=w3219:dbl, element #2=w3218:dbl, element #3=w3217:dbl)
            }
            frame 1 {
              n424 = Index Array(array=w3222, index (row) #1=w3226, index (col) #1=0, index (row) #2=w3226, index (col) #2=1, index (row) #3=w3226, index (col) #3=2) -> (element #1=w3225:dbl, element #2=w3224:dbl, element #3=w3223:dbl)
            }
            frame 2 {
              n425 = Index Array(array=w3230, index (row) #1=w3234, index (col) #1=0, index (row) #2=w3234, index (col) #2=1, index (row) #3=w3234, index (col) #3=2) -> (element #1=w3233:dbl, element #2=w3232:dbl, element #3=w3231:dbl)
            }
            frame 3 {
              n426 = Index Array(array=w3238, index (row) #1=w3242, index (col) #1=0, index (row) #2=w3242, index (col) #2=1, index (row) #3=w3242, index (col) #3=2) -> (element #1=w3240:dbl, element #2=w3241:dbl, element #3=w3239:dbl)
            }
            frame 4 {
              n427 = Index Array(array=w3246, index (row) #1=w3250, index (col) #1=0, index (row) #2=w3250, index (col) #2=1, index (row) #3=w3250, index (col) #3=2) -> (element #1=w3247:dbl, element #2=w3249:dbl, element #3=w3248:dbl)
            }
            frame 5 {
              n428 = Index Array(array=w3254, index (row) #1=w3255, index (col) #1=0, index (row) #2=w3255, index (col) #2=1, index (row) #3=w3255, index (col) #3=2) -> (element #1=w3256:dbl, element #2=w3257:dbl, element #3=w3258:dbl)
            }
            frame 6 {
              n429 = Index Array(array=w3262, index (row) #1=w3266, index (col) #1=0, index (row) #2=w3266, index (col) #2=1, index (row) #3=w3266, index (col) #3=2) -> (element #1=w3263:dbl, element #2=w3265:dbl, element #3=w3264:dbl)
            }
            frame 7 {
              n430 = Index Array(array=w3270, index (row) #1=w3271, index (col) #1=0, index (row) #2=w3271, index (col) #2=1, index (row) #3=w3271, index (col) #3=2) -> (element #1=w3272:dbl, element #2=w3274:dbl, element #3=w3273:dbl)
            }
          }
        }
        frame "South east" {
          w3282 = 2
          n431 = case shown="2" w3282 {
            tunnel: [w3286 w3292 w3300 w3308 w3316 w3325 w3332 w3341] -> w3281
            tunnel: [w3288 w3294 w3302 w3309 w3318 w3327 w3334 w3343] -> w3280
            tunnel: [w3287 w3293 w3301 w3310 w3317 w3326 w3333 w3342] -> w3279
            tunnel: w3282 -> [w3290 w3295 w3303 w3311 w3319 w3324 w3335 w3340]
            tunnel: w3278 -> [w3283 w3291 w3299 w3307 w3315 w3323 w3331 w3339]
            frame 0, Default {
              n432 = Index Array(array=w3283, index (row) #1=w3290, index (col) #1=0, index (row) #2=w3290, index (col) #2=1, index (row) #3=w3290, index (col) #3=2) -> (element #1=w3288:dbl, element #2=w3287:dbl, element #3=w3286:dbl)
            }
            frame 1 {
              n433 = Index Array(array=w3291, index (row) #1=w3295, index (col) #1=0, index (row) #2=w3295, index (col) #2=1, index (row) #3=w3295, index (col) #3=2) -> (element #1=w3294:dbl, element #2=w3293:dbl, element #3=w3292:dbl)
            }
            frame 2 {
              n434 = Index Array(array=w3299, index (row) #1=w3303, index (col) #1=0, index (row) #2=w3303, index (col) #2=1, index (row) #3=w3303, index (col) #3=2) -> (element #1=w3302:dbl, element #2=w3301:dbl, element #3=w3300:dbl)
            }
            frame 3 {
              n435 = Index Array(array=w3307, index (row) #1=w3311, index (col) #1=0, index (row) #2=w3311, index (col) #2=1, index (row) #3=w3311, index (col) #3=2) -> (element #1=w3309:dbl, element #2=w3310:dbl, element #3=w3308:dbl)
            }
            frame 4 {
              n436 = Index Array(array=w3315, index (row) #1=w3319, index (col) #1=0, index (row) #2=w3319, index (col) #2=1, index (row) #3=w3319, index (col) #3=2) -> (element #1=w3316:dbl, element #2=w3318:dbl, element #3=w3317:dbl)
            }
            frame 5 {
              n437 = Index Array(array=w3323, index (row) #1=w3324, index (col) #1=0, index (row) #2=w3324, index (col) #2=1, index (row) #3=w3324, index (col) #3=2) -> (element #1=w3325:dbl, element #2=w3326:dbl, element #3=w3327:dbl)
            }
            frame 6 {
              n438 = Index Array(array=w3331, index (row) #1=w3335, index (col) #1=0, index (row) #2=w3335, index (col) #2=1, index (row) #3=w3335, index (col) #3=2) -> (element #1=w3332:dbl, element #2=w3334:dbl, element #3=w3333:dbl)
            }
            frame 7 {
              n439 = Index Array(array=w3339, index (row) #1=w3340, index (col) #1=0, index (row) #2=w3340, index (col) #2=1, index (row) #3=w3340, index (col) #3=2) -> (element #1=w3341:dbl, element #2=w3343:dbl, element #3=w3342:dbl)
            }
          }
        }
      }
    }
    frame "South west" {
      n440 = case shown="\"North\", Default" w3348 {
        tunnel: [w3355 w3425 w3493 w3560 w3630 w3700 w3768 w3838] -> w3351
        tunnel: [w3354 w3424 w3492 w3561 w3629 w3698 w3767 w3837] -> w3350
        tunnel: [w3353 w3423 w3491 w3559 w3628 w3697 w3766 w3836] -> w3349
        tunnel: w3347 -> [w3352 w3421 w3490 w3562 w3631 w3699 w3769 w3835]
        frame "North", Default {
          w3356 = 6
          n441 = case shown="2" w3356 {
            tunnel: [w3360 w3366 w3374 w3382 w3390 w3399 w3406 w3415] -> w3355
            tunnel: [w3362 w3368 w3376 w3383 w3392 w3401 w3408 w3417] -> w3354
            tunnel: [w3361 w3367 w3375 w3384 w3391 w3400 w3407 w3416] -> w3353
            tunnel: w3356 -> [w3364 w3369 w3377 w3385 w3393 w3398 w3409 w3414]
            tunnel: w3352 -> [w3357 w3365 w3373 w3381 w3389 w3397 w3405 w3413]
            frame 0, Default {
              n442 = Index Array(array=w3357, index (row) #1=w3364, index (col) #1=0, index (row) #2=w3364, index (col) #2=1, index (row) #3=w3364, index (col) #3=2) -> (element #1=w3362:dbl, element #2=w3361:dbl, element #3=w3360:dbl)
            }
            frame 1 {
              n443 = Index Array(array=w3365, index (row) #1=w3369, index (col) #1=0, index (row) #2=w3369, index (col) #2=1, index (row) #3=w3369, index (col) #3=2) -> (element #1=w3368:dbl, element #2=w3367:dbl, element #3=w3366:dbl)
            }
            frame 2 {
              n444 = Index Array(array=w3373, index (row) #1=w3377, index (col) #1=0, index (row) #2=w3377, index (col) #2=1, index (row) #3=w3377, index (col) #3=2) -> (element #1=w3376:dbl, element #2=w3375:dbl, element #3=w3374:dbl)
            }
            frame 3 {
              n445 = Index Array(array=w3381, index (row) #1=w3385, index (col) #1=0, index (row) #2=w3385, index (col) #2=1, index (row) #3=w3385, index (col) #3=2) -> (element #1=w3383:dbl, element #2=w3384:dbl, element #3=w3382:dbl)
            }
            frame 4 {
              n446 = Index Array(array=w3389, index (row) #1=w3393, index (col) #1=0, index (row) #2=w3393, index (col) #2=1, index (row) #3=w3393, index (col) #3=2) -> (element #1=w3390:dbl, element #2=w3392:dbl, element #3=w3391:dbl)
            }
            frame 5 {
              n447 = Index Array(array=w3397, index (row) #1=w3398, index (col) #1=0, index (row) #2=w3398, index (col) #2=1, index (row) #3=w3398, index (col) #3=2) -> (element #1=w3399:dbl, element #2=w3400:dbl, element #3=w3401:dbl)
            }
            frame 6 {
              n448 = Index Array(array=w3405, index (row) #1=w3409, index (col) #1=0, index (row) #2=w3409, index (col) #2=1, index (row) #3=w3409, index (col) #3=2) -> (element #1=w3406:dbl, element #2=w3408:dbl, element #3=w3407:dbl)
            }
            frame 7 {
              n449 = Index Array(array=w3413, index (row) #1=w3414, index (col) #1=0, index (row) #2=w3414, index (col) #2=1, index (row) #3=w3414, index (col) #3=2) -> (element #1=w3415:dbl, element #2=w3417:dbl, element #3=w3416:dbl)
            }
          }
        }
        frame "North east" {
          w3422 = 7
          n450 = case shown="2" w3422 {
            tunnel: [w3429 w3435 w3443 w3451 w3459 w3468 w3475 w3484] -> w3425
            tunnel: [w3431 w3437 w3445 w3452 w3461 w3470 w3477 w3486] -> w3424
            tunnel: [w3430 w3436 w3444 w3453 w3460 w3469 w3476 w3485] -> w3423
            tunnel: w3422 -> [w3433 w3438 w3446 w3454 w3462 w3467 w3478 w3483]
            tunnel: w3421 -> [w3426 w3434 w3442 w3450 w3458 w3466 w3474 w3482]
            frame 0, Default {
              n451 = Index Array(array=w3426, index (row) #1=w3433, index (col) #1=0, index (row) #2=w3433, index (col) #2=1, index (row) #3=w3433, index (col) #3=2) -> (element #1=w3431:dbl, element #2=w3430:dbl, element #3=w3429:dbl)
            }
            frame 1 {
              n452 = Index Array(array=w3434, index (row) #1=w3438, index (col) #1=0, index (row) #2=w3438, index (col) #2=1, index (row) #3=w3438, index (col) #3=2) -> (element #1=w3437:dbl, element #2=w3436:dbl, element #3=w3435:dbl)
            }
            frame 2 {
              n453 = Index Array(array=w3442, index (row) #1=w3446, index (col) #1=0, index (row) #2=w3446, index (col) #2=1, index (row) #3=w3446, index (col) #3=2) -> (element #1=w3445:dbl, element #2=w3444:dbl, element #3=w3443:dbl)
            }
            frame 3 {
              n454 = Index Array(array=w3450, index (row) #1=w3454, index (col) #1=0, index (row) #2=w3454, index (col) #2=1, index (row) #3=w3454, index (col) #3=2) -> (element #1=w3452:dbl, element #2=w3453:dbl, element #3=w3451:dbl)
            }
            frame 4 {
              n455 = Index Array(array=w3458, index (row) #1=w3462, index (col) #1=0, index (row) #2=w3462, index (col) #2=1, index (row) #3=w3462, index (col) #3=2) -> (element #1=w3459:dbl, element #2=w3461:dbl, element #3=w3460:dbl)
            }
            frame 5 {
              n456 = Index Array(array=w3466, index (row) #1=w3467, index (col) #1=0, index (row) #2=w3467, index (col) #2=1, index (row) #3=w3467, index (col) #3=2) -> (element #1=w3468:dbl, element #2=w3469:dbl, element #3=w3470:dbl)
            }
            frame 6 {
              n457 = Index Array(array=w3474, index (row) #1=w3478, index (col) #1=0, index (row) #2=w3478, index (col) #2=1, index (row) #3=w3478, index (col) #3=2) -> (element #1=w3475:dbl, element #2=w3477:dbl, element #3=w3476:dbl)
            }
            frame 7 {
              n458 = Index Array(array=w3482, index (row) #1=w3483, index (col) #1=0, index (row) #2=w3483, index (col) #2=1, index (row) #3=w3483, index (col) #3=2) -> (element #1=w3484:dbl, element #2=w3486:dbl, element #3=w3485:dbl)
            }
          }
        }
        frame "North west" {
          w3494 = 4
          n459 = case shown="2" w3494 {
            tunnel: [w3498 w3504 w3512 w3520 w3528 w3537 w3544 w3553] -> w3493
            tunnel: [w3500 w3506 w3514 w3521 w3530 w3539 w3546 w3555] -> w3492
            tunnel: [w3499 w3505 w3513 w3522 w3529 w3538 w3545 w3554] -> w3491
            tunnel: w3494 -> [w3502 w3507 w3515 w3523 w3531 w3536 w3547 w3552]
            tunnel: w3490 -> [w3495 w3503 w3511 w3519 w3527 w3535 w3543 w3551]
            frame 0, Default {
              n460 = Index Array(array=w3495, index (row) #1=w3502, index (col) #1=0, index (row) #2=w3502, index (col) #2=1, index (row) #3=w3502, index (col) #3=2) -> (element #1=w3500:dbl, element #2=w3499:dbl, element #3=w3498:dbl)
            }
            frame 1 {
              n461 = Index Array(array=w3503, index (row) #1=w3507, index (col) #1=0, index (row) #2=w3507, index (col) #2=1, index (row) #3=w3507, index (col) #3=2) -> (element #1=w3506:dbl, element #2=w3505:dbl, element #3=w3504:dbl)
            }
            frame 2 {
              n462 = Index Array(array=w3511, index (row) #1=w3515, index (col) #1=0, index (row) #2=w3515, index (col) #2=1, index (row) #3=w3515, index (col) #3=2) -> (element #1=w3514:dbl, element #2=w3513:dbl, element #3=w3512:dbl)
            }
            frame 3 {
              n463 = Index Array(array=w3519, index (row) #1=w3523, index (col) #1=0, index (row) #2=w3523, index (col) #2=1, index (row) #3=w3523, index (col) #3=2) -> (element #1=w3521:dbl, element #2=w3522:dbl, element #3=w3520:dbl)
            }
            frame 4 {
              n464 = Index Array(array=w3527, index (row) #1=w3531, index (col) #1=0, index (row) #2=w3531, index (col) #2=1, index (row) #3=w3531, index (col) #3=2) -> (element #1=w3528:dbl, element #2=w3530:dbl, element #3=w3529:dbl)
            }
            frame 5 {
              n465 = Index Array(array=w3535, index (row) #1=w3536, index (col) #1=0, index (row) #2=w3536, index (col) #2=1, index (row) #3=w3536, index (col) #3=2) -> (element #1=w3537:dbl, element #2=w3538:dbl, element #3=w3539:dbl)
            }
            frame 6 {
              n466 = Index Array(array=w3543, index (row) #1=w3547, index (col) #1=0, index (row) #2=w3547, index (col) #2=1, index (row) #3=w3547, index (col) #3=2) -> (element #1=w3544:dbl, element #2=w3546:dbl, element #3=w3545:dbl)
            }
            frame 7 {
              n467 = Index Array(array=w3551, index (row) #1=w3552, index (col) #1=0, index (row) #2=w3552, index (col) #2=1, index (row) #3=w3552, index (col) #3=2) -> (element #1=w3553:dbl, element #2=w3555:dbl, element #3=w3554:dbl)
            }
          }
        }
        frame "West" {
          w3563 = 2
          n468 = case shown="2" w3563 {
            tunnel: [w3567 w3573 w3581 w3589 w3597 w3606 w3613 w3622] -> w3560
            tunnel: [w3569 w3575 w3583 w3590 w3599 w3608 w3615 w3624] -> w3561
            tunnel: [w3568 w3574 w3582 w3591 w3598 w3607 w3614 w3623] -> w3559
            tunnel: w3563 -> [w3571 w3576 w3584 w3592 w3600 w3605 w3616 w3621]
            tunnel: w3562 -> [w3564 w3572 w3580 w3588 w3596 w3604 w3612 w3620]
            frame 0, Default {
              n469 = Index Array(array=w3564, index (row) #1=w3571, index (col) #1=0, index (row) #2=w3571, index (col) #2=1, index (row) #3=w3571, index (col) #3=2) -> (element #1=w3569:dbl, element #2=w3568:dbl, element #3=w3567:dbl)
            }
            frame 1 {
              n470 = Index Array(array=w3572, index (row) #1=w3576, index (col) #1=0, index (row) #2=w3576, index (col) #2=1, index (row) #3=w3576, index (col) #3=2) -> (element #1=w3575:dbl, element #2=w3574:dbl, element #3=w3573:dbl)
            }
            frame 2 {
              n471 = Index Array(array=w3580, index (row) #1=w3584, index (col) #1=0, index (row) #2=w3584, index (col) #2=1, index (row) #3=w3584, index (col) #3=2) -> (element #1=w3583:dbl, element #2=w3582:dbl, element #3=w3581:dbl)
            }
            frame 3 {
              n472 = Index Array(array=w3588, index (row) #1=w3592, index (col) #1=0, index (row) #2=w3592, index (col) #2=1, index (row) #3=w3592, index (col) #3=2) -> (element #1=w3590:dbl, element #2=w3591:dbl, element #3=w3589:dbl)
            }
            frame 4 {
              n473 = Index Array(array=w3596, index (row) #1=w3600, index (col) #1=0, index (row) #2=w3600, index (col) #2=1, index (row) #3=w3600, index (col) #3=2) -> (element #1=w3597:dbl, element #2=w3599:dbl, element #3=w3598:dbl)
            }
            frame 5 {
              n474 = Index Array(array=w3604, index (row) #1=w3605, index (col) #1=0, index (row) #2=w3605, index (col) #2=1, index (row) #3=w3605, index (col) #3=2) -> (element #1=w3606:dbl, element #2=w3607:dbl, element #3=w3608:dbl)
            }
            frame 6 {
              n475 = Index Array(array=w3612, index (row) #1=w3616, index (col) #1=0, index (row) #2=w3616, index (col) #2=1, index (row) #3=w3616, index (col) #3=2) -> (element #1=w3613:dbl, element #2=w3615:dbl, element #3=w3614:dbl)
            }
            frame 7 {
              n476 = Index Array(array=w3620, index (row) #1=w3621, index (col) #1=0, index (row) #2=w3621, index (col) #2=1, index (row) #3=w3621, index (col) #3=2) -> (element #1=w3622:dbl, element #2=w3624:dbl, element #3=w3623:dbl)
            }
          }
        }
        frame "East" {
          w3632 = 5
          n477 = case shown="2" w3632 {
            tunnel: [w3636 w3642 w3650 w3658 w3666 w3675 w3682 w3691] -> w3630
            tunnel: [w3638 w3644 w3652 w3659 w3668 w3677 w3684 w3693] -> w3629
            tunnel: [w3637 w3643 w3651 w3660 w3667 w3676 w3683 w3692] -> w3628
            tunnel: w3632 -> [w3640 w3645 w3653 w3661 w3669 w3674 w3685 w3690]
            tunnel: w3631 -> [w3633 w3641 w3649 w3657 w3665 w3673 w3681 w3689]
            frame 0, Default {
              n478 = Index Array(array=w3633, index (row) #1=w3640, index (col) #1=0, index (row) #2=w3640, index (col) #2=1, index (row) #3=w3640, index (col) #3=2) -> (element #1=w3638:dbl, element #2=w3637:dbl, element #3=w3636:dbl)
            }
            frame 1 {
              n479 = Index Array(array=w3641, index (row) #1=w3645, index (col) #1=0, index (row) #2=w3645, index (col) #2=1, index (row) #3=w3645, index (col) #3=2) -> (element #1=w3644:dbl, element #2=w3643:dbl, element #3=w3642:dbl)
            }
            frame 2 {
              n480 = Index Array(array=w3649, index (row) #1=w3653, index (col) #1=0, index (row) #2=w3653, index (col) #2=1, index (row) #3=w3653, index (col) #3=2) -> (element #1=w3652:dbl, element #2=w3651:dbl, element #3=w3650:dbl)
            }
            frame 3 {
              n481 = Index Array(array=w3657, index (row) #1=w3661, index (col) #1=0, index (row) #2=w3661, index (col) #2=1, index (row) #3=w3661, index (col) #3=2) -> (element #1=w3659:dbl, element #2=w3660:dbl, element #3=w3658:dbl)
            }
            frame 4 {
              n482 = Index Array(array=w3665, index (row) #1=w3669, index (col) #1=0, index (row) #2=w3669, index (col) #2=1, index (row) #3=w3669, index (col) #3=2) -> (element #1=w3666:dbl, element #2=w3668:dbl, element #3=w3667:dbl)
            }
            frame 5 {
              n483 = Index Array(array=w3673, index (row) #1=w3674, index (col) #1=0, index (row) #2=w3674, index (col) #2=1, index (row) #3=w3674, index (col) #3=2) -> (element #1=w3675:dbl, element #2=w3676:dbl, element #3=w3677:dbl)
            }
            frame 6 {
              n484 = Index Array(array=w3681, index (row) #1=w3685, index (col) #1=0, index (row) #2=w3685, index (col) #2=1, index (row) #3=w3685, index (col) #3=2) -> (element #1=w3682:dbl, element #2=w3684:dbl, element #3=w3683:dbl)
            }
            frame 7 {
              n485 = Index Array(array=w3689, index (row) #1=w3690, index (col) #1=0, index (row) #2=w3690, index (col) #2=1, index (row) #3=w3690, index (col) #3=2) -> (element #1=w3691:dbl, element #2=w3693:dbl, element #3=w3692:dbl)
            }
          }
        }
        frame "South" {
          w3701 = 1
          n486 = case shown="2" w3701 {
            tunnel: [w3705 w3711 w3719 w3727 w3735 w3744 w3751 w3760] -> w3700
            tunnel: [w3707 w3713 w3721 w3728 w3737 w3746 w3753 w3762] -> w3698
            tunnel: [w3706 w3712 w3720 w3729 w3736 w3745 w3752 w3761] -> w3697
            tunnel: w3701 -> [w3709 w3714 w3722 w3730 w3738 w3743 w3754 w3759]
            tunnel: w3699 -> [w3702 w3710 w3718 w3726 w3734 w3742 w3750 w3758]
            frame 0, Default {
              n487 = Index Array(array=w3702, index (row) #1=w3709, index (col) #1=0, index (row) #2=w3709, index (col) #2=1, index (row) #3=w3709, index (col) #3=2) -> (element #1=w3707:dbl, element #2=w3706:dbl, element #3=w3705:dbl)
            }
            frame 1 {
              n488 = Index Array(array=w3710, index (row) #1=w3714, index (col) #1=0, index (row) #2=w3714, index (col) #2=1, index (row) #3=w3714, index (col) #3=2) -> (element #1=w3713:dbl, element #2=w3712:dbl, element #3=w3711:dbl)
            }
            frame 2 {
              n489 = Index Array(array=w3718, index (row) #1=w3722, index (col) #1=0, index (row) #2=w3722, index (col) #2=1, index (row) #3=w3722, index (col) #3=2) -> (element #1=w3721:dbl, element #2=w3720:dbl, element #3=w3719:dbl)
            }
            frame 3 {
              n490 = Index Array(array=w3726, index (row) #1=w3730, index (col) #1=0, index (row) #2=w3730, index (col) #2=1, index (row) #3=w3730, index (col) #3=2) -> (element #1=w3728:dbl, element #2=w3729:dbl, element #3=w3727:dbl)
            }
            frame 4 {
              n491 = Index Array(array=w3734, index (row) #1=w3738, index (col) #1=0, index (row) #2=w3738, index (col) #2=1, index (row) #3=w3738, index (col) #3=2) -> (element #1=w3735:dbl, element #2=w3737:dbl, element #3=w3736:dbl)
            }
            frame 5 {
              n492 = Index Array(array=w3742, index (row) #1=w3743, index (col) #1=0, index (row) #2=w3743, index (col) #2=1, index (row) #3=w3743, index (col) #3=2) -> (element #1=w3744:dbl, element #2=w3745:dbl, element #3=w3746:dbl)
            }
            frame 6 {
              n493 = Index Array(array=w3750, index (row) #1=w3754, index (col) #1=0, index (row) #2=w3754, index (col) #2=1, index (row) #3=w3754, index (col) #3=2) -> (element #1=w3751:dbl, element #2=w3753:dbl, element #3=w3752:dbl)
            }
            frame 7 {
              n494 = Index Array(array=w3758, index (row) #1=w3759, index (col) #1=0, index (row) #2=w3759, index (col) #2=1, index (row) #3=w3759, index (col) #3=2) -> (element #1=w3760:dbl, element #2=w3762:dbl, element #3=w3761:dbl)
            }
          }
        }
        frame "South west" {
          w3770 = 0
          n495 = case shown="2" w3770 {
            tunnel: [w3774 w3780 w3788 w3796 w3804 w3813 w3820 w3829] -> w3768
            tunnel: [w3776 w3782 w3790 w3797 w3806 w3815 w3822 w3831] -> w3767
            tunnel: [w3775 w3781 w3789 w3798 w3805 w3814 w3821 w3830] -> w3766
            tunnel: w3770 -> [w3778 w3783 w3791 w3799 w3807 w3812 w3823 w3828]
            tunnel: w3769 -> [w3771 w3779 w3787 w3795 w3803 w3811 w3819 w3827]
            frame 0, Default {
              n496 = Index Array(array=w3771, index (row) #1=w3778, index (col) #1=0, index (row) #2=w3778, index (col) #2=1, index (row) #3=w3778, index (col) #3=2) -> (element #1=w3776:dbl, element #2=w3775:dbl, element #3=w3774:dbl)
            }
            frame 1 {
              n497 = Index Array(array=w3779, index (row) #1=w3783, index (col) #1=0, index (row) #2=w3783, index (col) #2=1, index (row) #3=w3783, index (col) #3=2) -> (element #1=w3782:dbl, element #2=w3781:dbl, element #3=w3780:dbl)
            }
            frame 2 {
              n498 = Index Array(array=w3787, index (row) #1=w3791, index (col) #1=0, index (row) #2=w3791, index (col) #2=1, index (row) #3=w3791, index (col) #3=2) -> (element #1=w3790:dbl, element #2=w3789:dbl, element #3=w3788:dbl)
            }
            frame 3 {
              n499 = Index Array(array=w3795, index (row) #1=w3799, index (col) #1=0, index (row) #2=w3799, index (col) #2=1, index (row) #3=w3799, index (col) #3=2) -> (element #1=w3797:dbl, element #2=w3798:dbl, element #3=w3796:dbl)
            }
            frame 4 {
              n500 = Index Array(array=w3803, index (row) #1=w3807, index (col) #1=0, index (row) #2=w3807, index (col) #2=1, index (row) #3=w3807, index (col) #3=2) -> (element #1=w3804:dbl, element #2=w3806:dbl, element #3=w3805:dbl)
            }
            frame 5 {
              n501 = Index Array(array=w3811, index (row) #1=w3812, index (col) #1=0, index (row) #2=w3812, index (col) #2=1, index (row) #3=w3812, index (col) #3=2) -> (element #1=w3813:dbl, element #2=w3814:dbl, element #3=w3815:dbl)
            }
            frame 6 {
              n502 = Index Array(array=w3819, index (row) #1=w3823, index (col) #1=0, index (row) #2=w3823, index (col) #2=1, index (row) #3=w3823, index (col) #3=2) -> (element #1=w3820:dbl, element #2=w3822:dbl, element #3=w3821:dbl)
            }
            frame 7 {
              n503 = Index Array(array=w3827, index (row) #1=w3828, index (col) #1=0, index (row) #2=w3828, index (col) #2=1, index (row) #3=w3828, index (col) #3=2) -> (element #1=w3829:dbl, element #2=w3831:dbl, element #3=w3830:dbl)
            }
          }
        }
        frame "South east" {
          w3839 = 3
          n504 = case shown="2" w3839 {
            tunnel: [w3843 w3849 w3857 w3865 w3873 w3882 w3889 w3898] -> w3838
            tunnel: [w3845 w3851 w3859 w3866 w3875 w3884 w3891 w3900] -> w3837
            tunnel: [w3844 w3850 w3858 w3867 w3874 w3883 w3890 w3899] -> w3836
            tunnel: w3839 -> [w3847 w3852 w3860 w3868 w3876 w3881 w3892 w3897]
            tunnel: w3835 -> [w3840 w3848 w3856 w3864 w3872 w3880 w3888 w3896]
            frame 0, Default {
              n505 = Index Array(array=w3840, index (row) #1=w3847, index (col) #1=0, index (row) #2=w3847, index (col) #2=1, index (row) #3=w3847, index (col) #3=2) -> (element #1=w3845:dbl, element #2=w3844:dbl, element #3=w3843:dbl)
            }
            frame 1 {
              n506 = Index Array(array=w3848, index (row) #1=w3852, index (col) #1=0, index (row) #2=w3852, index (col) #2=1, index (row) #3=w3852, index (col) #3=2) -> (element #1=w3851:dbl, element #2=w3850:dbl, element #3=w3849:dbl)
            }
            frame 2 {
              n507 = Index Array(array=w3856, index (row) #1=w3860, index (col) #1=0, index (row) #2=w3860, index (col) #2=1, index (row) #3=w3860, index (col) #3=2) -> (element #1=w3859:dbl, element #2=w3858:dbl, element #3=w3857:dbl)
            }
            frame 3 {
              n508 = Index Array(array=w3864, index (row) #1=w3868, index (col) #1=0, index (row) #2=w3868, index (col) #2=1, index (row) #3=w3868, index (col) #3=2) -> (element #1=w3866:dbl, element #2=w3867:dbl, element #3=w3865:dbl)
            }
            frame 4 {
              n509 = Index Array(array=w3872, index (row) #1=w3876, index (col) #1=0, index (row) #2=w3876, index (col) #2=1, index (row) #3=w3876, index (col) #3=2) -> (element #1=w3873:dbl, element #2=w3875:dbl, element #3=w3874:dbl)
            }
            frame 5 {
              n510 = Index Array(array=w3880, index (row) #1=w3881, index (col) #1=0, index (row) #2=w3881, index (col) #2=1, index (row) #3=w3881, index (col) #3=2) -> (element #1=w3882:dbl, element #2=w3883:dbl, element #3=w3884:dbl)
            }
            frame 6 {
              n511 = Index Array(array=w3888, index (row) #1=w3892, index (col) #1=0, index (row) #2=w3892, index (col) #2=1, index (row) #3=w3892, index (col) #3=2) -> (element #1=w3889:dbl, element #2=w3891:dbl, element #3=w3890:dbl)
            }
            frame 7 {
              n512 = Index Array(array=w3896, index (row) #1=w3897, index (col) #1=0, index (row) #2=w3897, index (col) #2=1, index (row) #3=w3897, index (col) #3=2) -> (element #1=w3898:dbl, element #2=w3900:dbl, element #3=w3899:dbl)
            }
          }
        }
      }
    }
    frame "South east" {
      n513 = case shown="\"North\", Default" w3905 {
        tunnel: [w3912 w3982 w4050 w4117 w4187 w4257 w4325 w4395] -> w3908
        tunnel: [w3911 w3981 w4049 w4118 w4186 w4255 w4324 w4394] -> w3907
        tunnel: [w3910 w3980 w4048 w4116 w4185 w4254 w4323 w4393] -> w3906
        tunnel: w3904 -> [w3909 w3978 w4047 w4119 w4188 w4256 w4326 w4392]
        frame "North", Default {
          w3913 = 5
          n514 = case shown="2" w3913 {
            tunnel: [w3917 w3923 w3931 w3939 w3947 w3956 w3963 w3972] -> w3912
            tunnel: [w3919 w3925 w3933 w3940 w3949 w3958 w3965 w3974] -> w3911
            tunnel: [w3918 w3924 w3932 w3941 w3948 w3957 w3964 w3973] -> w3910
            tunnel: w3913 -> [w3921 w3926 w3934 w3942 w3950 w3955 w3966 w3971]
            tunnel: w3909 -> [w3914 w3922 w3930 w3938 w3946 w3954 w3962 w3970]
            frame 0, Default {
              n515 = Index Array(array=w3914, index (row) #1=w3921, index (col) #1=0, index (row) #2=w3921, index (col) #2=1, index (row) #3=w3921, index (col) #3=2) -> (element #1=w3919:dbl, element #2=w3918:dbl, element #3=w3917:dbl)
            }
            frame 1 {
              n516 = Index Array(array=w3922, index (row) #1=w3926, index (col) #1=0, index (row) #2=w3926, index (col) #2=1, index (row) #3=w3926, index (col) #3=2) -> (element #1=w3925:dbl, element #2=w3924:dbl, element #3=w3923:dbl)
            }
            frame 2 {
              n517 = Index Array(array=w3930, index (row) #1=w3934, index (col) #1=0, index (row) #2=w3934, index (col) #2=1, index (row) #3=w3934, index (col) #3=2) -> (element #1=w3933:dbl, element #2=w3932:dbl, element #3=w3931:dbl)
            }
            frame 3 {
              n518 = Index Array(array=w3938, index (row) #1=w3942, index (col) #1=0, index (row) #2=w3942, index (col) #2=1, index (row) #3=w3942, index (col) #3=2) -> (element #1=w3940:dbl, element #2=w3941:dbl, element #3=w3939:dbl)
            }
            frame 4 {
              n519 = Index Array(array=w3946, index (row) #1=w3950, index (col) #1=0, index (row) #2=w3950, index (col) #2=1, index (row) #3=w3950, index (col) #3=2) -> (element #1=w3947:dbl, element #2=w3949:dbl, element #3=w3948:dbl)
            }
            frame 5 {
              n520 = Index Array(array=w3954, index (row) #1=w3955, index (col) #1=0, index (row) #2=w3955, index (col) #2=1, index (row) #3=w3955, index (col) #3=2) -> (element #1=w3956:dbl, element #2=w3957:dbl, element #3=w3958:dbl)
            }
            frame 6 {
              n521 = Index Array(array=w3962, index (row) #1=w3966, index (col) #1=0, index (row) #2=w3966, index (col) #2=1, index (row) #3=w3966, index (col) #3=2) -> (element #1=w3963:dbl, element #2=w3965:dbl, element #3=w3964:dbl)
            }
            frame 7 {
              n522 = Index Array(array=w3970, index (row) #1=w3971, index (col) #1=0, index (row) #2=w3971, index (col) #2=1, index (row) #3=w3971, index (col) #3=2) -> (element #1=w3972:dbl, element #2=w3974:dbl, element #3=w3973:dbl)
            }
          }
        }
        frame "North east" {
          w3979 = 3
          n523 = case shown="2" w3979 {
            tunnel: [w3986 w3992 w4000 w4008 w4016 w4025 w4032 w4041] -> w3982
            tunnel: [w3988 w3994 w4002 w4009 w4018 w4027 w4034 w4043] -> w3981
            tunnel: [w3987 w3993 w4001 w4010 w4017 w4026 w4033 w4042] -> w3980
            tunnel: w3979 -> [w3990 w3995 w4003 w4011 w4019 w4024 w4035 w4040]
            tunnel: w3978 -> [w3983 w3991 w3999 w4007 w4015 w4023 w4031 w4039]
            frame 0, Default {
              n524 = Index Array(array=w3983, index (row) #1=w3990, index (col) #1=0, index (row) #2=w3990, index (col) #2=1, index (row) #3=w3990, index (col) #3=2) -> (element #1=w3988:dbl, element #2=w3987:dbl, element #3=w3986:dbl)
            }
            frame 1 {
              n525 = Index Array(array=w3991, index (row) #1=w3995, index (col) #1=0, index (row) #2=w3995, index (col) #2=1, index (row) #3=w3995, index (col) #3=2) -> (element #1=w3994:dbl, element #2=w3993:dbl, element #3=w3992:dbl)
            }
            frame 2 {
              n526 = Index Array(array=w3999, index (row) #1=w4003, index (col) #1=0, index (row) #2=w4003, index (col) #2=1, index (row) #3=w4003, index (col) #3=2) -> (element #1=w4002:dbl, element #2=w4001:dbl, element #3=w4000:dbl)
            }
            frame 3 {
              n527 = Index Array(array=w4007, index (row) #1=w4011, index (col) #1=0, index (row) #2=w4011, index (col) #2=1, index (row) #3=w4011, index (col) #3=2) -> (element #1=w4009:dbl, element #2=w4010:dbl, element #3=w4008:dbl)
            }
            frame 4 {
              n528 = Index Array(array=w4015, index (row) #1=w4019, index (col) #1=0, index (row) #2=w4019, index (col) #2=1, index (row) #3=w4019, index (col) #3=2) -> (element #1=w4016:dbl, element #2=w4018:dbl, element #3=w4017:dbl)
            }
            frame 5 {
              n529 = Index Array(array=w4023, index (row) #1=w4024, index (col) #1=0, index (row) #2=w4024, index (col) #2=1, index (row) #3=w4024, index (col) #3=2) -> (element #1=w4025:dbl, element #2=w4026:dbl, element #3=w4027:dbl)
            }
            frame 6 {
              n530 = Index Array(array=w4031, index (row) #1=w4035, index (col) #1=0, index (row) #2=w4035, index (col) #2=1, index (row) #3=w4035, index (col) #3=2) -> (element #1=w4032:dbl, element #2=w4034:dbl, element #3=w4033:dbl)
            }
            frame 7 {
              n531 = Index Array(array=w4039, index (row) #1=w4040, index (col) #1=0, index (row) #2=w4040, index (col) #2=1, index (row) #3=w4040, index (col) #3=2) -> (element #1=w4041:dbl, element #2=w4043:dbl, element #3=w4042:dbl)
            }
          }
        }
        frame "North west" {
          w4051 = 7
          n532 = case shown="2" w4051 {
            tunnel: [w4055 w4061 w4069 w4077 w4085 w4094 w4101 w4110] -> w4050
            tunnel: [w4057 w4063 w4071 w4078 w4087 w4096 w4103 w4112] -> w4049
            tunnel: [w4056 w4062 w4070 w4079 w4086 w4095 w4102 w4111] -> w4048
            tunnel: w4051 -> [w4059 w4064 w4072 w4080 w4088 w4093 w4104 w4109]
            tunnel: w4047 -> [w4052 w4060 w4068 w4076 w4084 w4092 w4100 w4108]
            frame 0, Default {
              n533 = Index Array(array=w4052, index (row) #1=w4059, index (col) #1=0, index (row) #2=w4059, index (col) #2=1, index (row) #3=w4059, index (col) #3=2) -> (element #1=w4057:dbl, element #2=w4056:dbl, element #3=w4055:dbl)
            }
            frame 1 {
              n534 = Index Array(array=w4060, index (row) #1=w4064, index (col) #1=0, index (row) #2=w4064, index (col) #2=1, index (row) #3=w4064, index (col) #3=2) -> (element #1=w4063:dbl, element #2=w4062:dbl, element #3=w4061:dbl)
            }
            frame 2 {
              n535 = Index Array(array=w4068, index (row) #1=w4072, index (col) #1=0, index (row) #2=w4072, index (col) #2=1, index (row) #3=w4072, index (col) #3=2) -> (element #1=w4071:dbl, element #2=w4070:dbl, element #3=w4069:dbl)
            }
            frame 3 {
              n536 = Index Array(array=w4076, index (row) #1=w4080, index (col) #1=0, index (row) #2=w4080, index (col) #2=1, index (row) #3=w4080, index (col) #3=2) -> (element #1=w4078:dbl, element #2=w4079:dbl, element #3=w4077:dbl)
            }
            frame 4 {
              n537 = Index Array(array=w4084, index (row) #1=w4088, index (col) #1=0, index (row) #2=w4088, index (col) #2=1, index (row) #3=w4088, index (col) #3=2) -> (element #1=w4085:dbl, element #2=w4087:dbl, element #3=w4086:dbl)
            }
            frame 5 {
              n538 = Index Array(array=w4092, index (row) #1=w4093, index (col) #1=0, index (row) #2=w4093, index (col) #2=1, index (row) #3=w4093, index (col) #3=2) -> (element #1=w4094:dbl, element #2=w4095:dbl, element #3=w4096:dbl)
            }
            frame 6 {
              n539 = Index Array(array=w4100, index (row) #1=w4104, index (col) #1=0, index (row) #2=w4104, index (col) #2=1, index (row) #3=w4104, index (col) #3=2) -> (element #1=w4101:dbl, element #2=w4103:dbl, element #3=w4102:dbl)
            }
            frame 7 {
              n540 = Index Array(array=w4108, index (row) #1=w4109, index (col) #1=0, index (row) #2=w4109, index (col) #2=1, index (row) #3=w4109, index (col) #3=2) -> (element #1=w4110:dbl, element #2=w4112:dbl, element #3=w4111:dbl)
            }
          }
        }
        frame "West" {
          w4120 = 6
          n541 = case shown="2" w4120 {
            tunnel: [w4124 w4130 w4138 w4146 w4154 w4163 w4170 w4179] -> w4117
            tunnel: [w4126 w4132 w4140 w4147 w4156 w4165 w4172 w4181] -> w4118
            tunnel: [w4125 w4131 w4139 w4148 w4155 w4164 w4171 w4180] -> w4116
            tunnel: w4120 -> [w4128 w4133 w4141 w4149 w4157 w4162 w4173 w4178]
            tunnel: w4119 -> [w4121 w4129 w4137 w4145 w4153 w4161 w4169 w4177]
            frame 0, Default {
              n542 = Index Array(array=w4121, index (row) #1=w4128, index (col) #1=0, index (row) #2=w4128, index (col) #2=1, index (row) #3=w4128, index (col) #3=2) -> (element #1=w4126:dbl, element #2=w4125:dbl, element #3=w4124:dbl)
            }
            frame 1 {
              n543 = Index Array(array=w4129, index (row) #1=w4133, index (col) #1=0, index (row) #2=w4133, index (col) #2=1, index (row) #3=w4133, index (col) #3=2) -> (element #1=w4132:dbl, element #2=w4131:dbl, element #3=w4130:dbl)
            }
            frame 2 {
              n544 = Index Array(array=w4137, index (row) #1=w4141, index (col) #1=0, index (row) #2=w4141, index (col) #2=1, index (row) #3=w4141, index (col) #3=2) -> (element #1=w4140:dbl, element #2=w4139:dbl, element #3=w4138:dbl)
            }
            frame 3 {
              n545 = Index Array(array=w4145, index (row) #1=w4149, index (col) #1=0, index (row) #2=w4149, index (col) #2=1, index (row) #3=w4149, index (col) #3=2) -> (element #1=w4147:dbl, element #2=w4148:dbl, element #3=w4146:dbl)
            }
            frame 4 {
              n546 = Index Array(array=w4153, index (row) #1=w4157, index (col) #1=0, index (row) #2=w4157, index (col) #2=1, index (row) #3=w4157, index (col) #3=2) -> (element #1=w4154:dbl, element #2=w4156:dbl, element #3=w4155:dbl)
            }
            frame 5 {
              n547 = Index Array(array=w4161, index (row) #1=w4162, index (col) #1=0, index (row) #2=w4162, index (col) #2=1, index (row) #3=w4162, index (col) #3=2) -> (element #1=w4163:dbl, element #2=w4164:dbl, element #3=w4165:dbl)
            }
            frame 6 {
              n548 = Index Array(array=w4169, index (row) #1=w4173, index (col) #1=0, index (row) #2=w4173, index (col) #2=1, index (row) #3=w4173, index (col) #3=2) -> (element #1=w4170:dbl, element #2=w4172:dbl, element #3=w4171:dbl)
            }
            frame 7 {
              n549 = Index Array(array=w4177, index (row) #1=w4178, index (col) #1=0, index (row) #2=w4178, index (col) #2=1, index (row) #3=w4178, index (col) #3=2) -> (element #1=w4179:dbl, element #2=w4181:dbl, element #3=w4180:dbl)
            }
          }
        }
        frame "East" {
          w4189 = 1
          n550 = case shown="2" w4189 {
            tunnel: [w4193 w4199 w4207 w4215 w4223 w4232 w4239 w4248] -> w4187
            tunnel: [w4195 w4201 w4209 w4216 w4225 w4234 w4241 w4250] -> w4186
            tunnel: [w4194 w4200 w4208 w4217 w4224 w4233 w4240 w4249] -> w4185
            tunnel: w4189 -> [w4197 w4202 w4210 w4218 w4226 w4231 w4242 w4247]
            tunnel: w4188 -> [w4190 w4198 w4206 w4214 w4222 w4230 w4238 w4246]
            frame 0, Default {
              n551 = Index Array(array=w4190, index (row) #1=w4197, index (col) #1=0, index (row) #2=w4197, index (col) #2=1, index (row) #3=w4197, index (col) #3=2) -> (element #1=w4195:dbl, element #2=w4194:dbl, element #3=w4193:dbl)
            }
            frame 1 {
              n552 = Index Array(array=w4198, index (row) #1=w4202, index (col) #1=0, index (row) #2=w4202, index (col) #2=1, index (row) #3=w4202, index (col) #3=2) -> (element #1=w4201:dbl, element #2=w4200:dbl, element #3=w4199:dbl)
            }
            frame 2 {
              n553 = Index Array(array=w4206, index (row) #1=w4210, index (col) #1=0, index (row) #2=w4210, index (col) #2=1, index (row) #3=w4210, index (col) #3=2) -> (element #1=w4209:dbl, element #2=w4208:dbl, element #3=w4207:dbl)
            }
            frame 3 {
              n554 = Index Array(array=w4214, index (row) #1=w4218, index (col) #1=0, index (row) #2=w4218, index (col) #2=1, index (row) #3=w4218, index (col) #3=2) -> (element #1=w4216:dbl, element #2=w4217:dbl, element #3=w4215:dbl)
            }
            frame 4 {
              n555 = Index Array(array=w4222, index (row) #1=w4226, index (col) #1=0, index (row) #2=w4226, index (col) #2=1, index (row) #3=w4226, index (col) #3=2) -> (element #1=w4223:dbl, element #2=w4225:dbl, element #3=w4224:dbl)
            }
            frame 5 {
              n556 = Index Array(array=w4230, index (row) #1=w4231, index (col) #1=0, index (row) #2=w4231, index (col) #2=1, index (row) #3=w4231, index (col) #3=2) -> (element #1=w4232:dbl, element #2=w4233:dbl, element #3=w4234:dbl)
            }
            frame 6 {
              n557 = Index Array(array=w4238, index (row) #1=w4242, index (col) #1=0, index (row) #2=w4242, index (col) #2=1, index (row) #3=w4242, index (col) #3=2) -> (element #1=w4239:dbl, element #2=w4241:dbl, element #3=w4240:dbl)
            }
            frame 7 {
              n558 = Index Array(array=w4246, index (row) #1=w4247, index (col) #1=0, index (row) #2=w4247, index (col) #2=1, index (row) #3=w4247, index (col) #3=2) -> (element #1=w4248:dbl, element #2=w4250:dbl, element #3=w4249:dbl)
            }
          }
        }
        frame "South" {
          w4258 = 2
          n559 = case shown="2" w4258 {
            tunnel: [w4262 w4268 w4276 w4284 w4292 w4301 w4308 w4317] -> w4257
            tunnel: [w4264 w4270 w4278 w4285 w4294 w4303 w4310 w4319] -> w4255
            tunnel: [w4263 w4269 w4277 w4286 w4293 w4302 w4309 w4318] -> w4254
            tunnel: w4258 -> [w4266 w4271 w4279 w4287 w4295 w4300 w4311 w4316]
            tunnel: w4256 -> [w4259 w4267 w4275 w4283 w4291 w4299 w4307 w4315]
            frame 0, Default {
              n560 = Index Array(array=w4259, index (row) #1=w4266, index (col) #1=0, index (row) #2=w4266, index (col) #2=1, index (row) #3=w4266, index (col) #3=2) -> (element #1=w4264:dbl, element #2=w4263:dbl, element #3=w4262:dbl)
            }
            frame 1 {
              n561 = Index Array(array=w4267, index (row) #1=w4271, index (col) #1=0, index (row) #2=w4271, index (col) #2=1, index (row) #3=w4271, index (col) #3=2) -> (element #1=w4270:dbl, element #2=w4269:dbl, element #3=w4268:dbl)
            }
            frame 2 {
              n562 = Index Array(array=w4275, index (row) #1=w4279, index (col) #1=0, index (row) #2=w4279, index (col) #2=1, index (row) #3=w4279, index (col) #3=2) -> (element #1=w4278:dbl, element #2=w4277:dbl, element #3=w4276:dbl)
            }
            frame 3 {
              n563 = Index Array(array=w4283, index (row) #1=w4287, index (col) #1=0, index (row) #2=w4287, index (col) #2=1, index (row) #3=w4287, index (col) #3=2) -> (element #1=w4285:dbl, element #2=w4286:dbl, element #3=w4284:dbl)
            }
            frame 4 {
              n564 = Index Array(array=w4291, index (row) #1=w4295, index (col) #1=0, index (row) #2=w4295, index (col) #2=1, index (row) #3=w4295, index (col) #3=2) -> (element #1=w4292:dbl, element #2=w4294:dbl, element #3=w4293:dbl)
            }
            frame 5 {
              n565 = Index Array(array=w4299, index (row) #1=w4300, index (col) #1=0, index (row) #2=w4300, index (col) #2=1, index (row) #3=w4300, index (col) #3=2) -> (element #1=w4301:dbl, element #2=w4302:dbl, element #3=w4303:dbl)
            }
            frame 6 {
              n566 = Index Array(array=w4307, index (row) #1=w4311, index (col) #1=0, index (row) #2=w4311, index (col) #2=1, index (row) #3=w4311, index (col) #3=2) -> (element #1=w4308:dbl, element #2=w4310:dbl, element #3=w4309:dbl)
            }
            frame 7 {
              n567 = Index Array(array=w4315, index (row) #1=w4316, index (col) #1=0, index (row) #2=w4316, index (col) #2=1, index (row) #3=w4316, index (col) #3=2) -> (element #1=w4317:dbl, element #2=w4319:dbl, element #3=w4318:dbl)
            }
          }
        }
        frame "South west" {
          w4327 = 4
          n568 = case shown="2" w4327 {
            tunnel: [w4331 w4337 w4345 w4353 w4361 w4370 w4377 w4386] -> w4325
            tunnel: [w4333 w4339 w4347 w4354 w4363 w4372 w4379 w4388] -> w4324
            tunnel: [w4332 w4338 w4346 w4355 w4362 w4371 w4378 w4387] -> w4323
            tunnel: w4327 -> [w4335 w4340 w4348 w4356 w4364 w4369 w4380 w4385]
            tunnel: w4326 -> [w4328 w4336 w4344 w4352 w4360 w4368 w4376 w4384]
            frame 0, Default {
              n569 = Index Array(array=w4328, index (row) #1=w4335, index (col) #1=0, index (row) #2=w4335, index (col) #2=1, index (row) #3=w4335, index (col) #3=2) -> (element #1=w4333:dbl, element #2=w4332:dbl, element #3=w4331:dbl)
            }
            frame 1 {
              n570 = Index Array(array=w4336, index (row) #1=w4340, index (col) #1=0, index (row) #2=w4340, index (col) #2=1, index (row) #3=w4340, index (col) #3=2) -> (element #1=w4339:dbl, element #2=w4338:dbl, element #3=w4337:dbl)
            }
            frame 2 {
              n571 = Index Array(array=w4344, index (row) #1=w4348, index (col) #1=0, index (row) #2=w4348, index (col) #2=1, index (row) #3=w4348, index (col) #3=2) -> (element #1=w4347:dbl, element #2=w4346:dbl, element #3=w4345:dbl)
            }
            frame 3 {
              n572 = Index Array(array=w4352, index (row) #1=w4356, index (col) #1=0, index (row) #2=w4356, index (col) #2=1, index (row) #3=w4356, index (col) #3=2) -> (element #1=w4354:dbl, element #2=w4355:dbl, element #3=w4353:dbl)
            }
            frame 4 {
              n573 = Index Array(array=w4360, index (row) #1=w4364, index (col) #1=0, index (row) #2=w4364, index (col) #2=1, index (row) #3=w4364, index (col) #3=2) -> (element #1=w4361:dbl, element #2=w4363:dbl, element #3=w4362:dbl)
            }
            frame 5 {
              n574 = Index Array(array=w4368, index (row) #1=w4369, index (col) #1=0, index (row) #2=w4369, index (col) #2=1, index (row) #3=w4369, index (col) #3=2) -> (element #1=w4370:dbl, element #2=w4371:dbl, element #3=w4372:dbl)
            }
            frame 6 {
              n575 = Index Array(array=w4376, index (row) #1=w4380, index (col) #1=0, index (row) #2=w4380, index (col) #2=1, index (row) #3=w4380, index (col) #3=2) -> (element #1=w4377:dbl, element #2=w4379:dbl, element #3=w4378:dbl)
            }
            frame 7 {
              n576 = Index Array(array=w4384, index (row) #1=w4385, index (col) #1=0, index (row) #2=w4385, index (col) #2=1, index (row) #3=w4385, index (col) #3=2) -> (element #1=w4386:dbl, element #2=w4388:dbl, element #3=w4387:dbl)
            }
          }
        }
        frame "South east" {
          w4396 = 0
          n577 = case shown="2" w4396 {
            tunnel: [w4400 w4406 w4414 w4422 w4430 w4439 w4446 w4455] -> w4395
            tunnel: [w4402 w4408 w4416 w4423 w4432 w4441 w4448 w4457] -> w4394
            tunnel: [w4401 w4407 w4415 w4424 w4431 w4440 w4447 w4456] -> w4393
            tunnel: w4396 -> [w4404 w4409 w4417 w4425 w4433 w4438 w4449 w4454]
            tunnel: w4392 -> [w4397 w4405 w4413 w4421 w4429 w4437 w4445 w4453]
            frame 0, Default {
              n578 = Index Array(array=w4397, index (row) #1=w4404, index (col) #1=0, index (row) #2=w4404, index (col) #2=1, index (row) #3=w4404, index (col) #3=2) -> (element #1=w4402:dbl, element #2=w4401:dbl, element #3=w4400:dbl)
            }
            frame 1 {
              n579 = Index Array(array=w4405, index (row) #1=w4409, index (col) #1=0, index (row) #2=w4409, index (col) #2=1, index (row) #3=w4409, index (col) #3=2) -> (element #1=w4408:dbl, element #2=w4407:dbl, element #3=w4406:dbl)
            }
            frame 2 {
              n580 = Index Array(array=w4413, index (row) #1=w4417, index (col) #1=0, index (row) #2=w4417, index (col) #2=1, index (row) #3=w4417, index (col) #3=2) -> (element #1=w4416:dbl, element #2=w4415:dbl, element #3=w4414:dbl)
            }
            frame 3 {
              n581 = Index Array(array=w4421, index (row) #1=w4425, index (col) #1=0, index (row) #2=w4425, index (col) #2=1, index (row) #3=w4425, index (col) #3=2) -> (element #1=w4423:dbl, element #2=w4424:dbl, element #3=w4422:dbl)
            }
            frame 4 {
              n582 = Index Array(array=w4429, index (row) #1=w4433, index (col) #1=0, index (row) #2=w4433, index (col) #2=1, index (row) #3=w4433, index (col) #3=2) -> (element #1=w4430:dbl, element #2=w4432:dbl, element #3=w4431:dbl)
            }
            frame 5 {
              n583 = Index Array(array=w4437, index (row) #1=w4438, index (col) #1=0, index (row) #2=w4438, index (col) #2=1, index (row) #3=w4438, index (col) #3=2) -> (element #1=w4439:dbl, element #2=w4440:dbl, element #3=w4441:dbl)
            }
            frame 6 {
              n584 = Index Array(array=w4445, index (row) #1=w4449, index (col) #1=0, index (row) #2=w4449, index (col) #2=1, index (row) #3=w4449, index (col) #3=2) -> (element #1=w4446:dbl, element #2=w4448:dbl, element #3=w4447:dbl)
            }
            frame 7 {
              n585 = Index Array(array=w4453, index (row) #1=w4454, index (col) #1=0, index (row) #2=w4454, index (col) #2=1, index (row) #3=w4454, index (col) #3=2) -> (element #1=w4455:dbl, element #2=w4457:dbl, element #3=w4456:dbl)
            }
          }
        }
      }
    }
  }
  n586 = local write "chosen  distance"(w1) -> ()
